vi "Core_Chem_User_Interface_v3.2_test.vi"() -> ()   [LabVIEW 2014]
uses:
  <vilib>/dex/Stream Element Allocation Mode.ctl
  C:/Program Files (x86)/National Instruments/LabVIEW 2014/examples/Data Communication/Network Streams/Simple Network Streams/support/Network Stream Command.ctl
  <vilib>/Platform/TimedLoop/XDataNode/timing_clust.ctl
  <vilib>/Platform/TimedLoop/XDataNode/nitl_modes.ctl
  <vilib>/Platform/TimedLoop/XDataNode/wakeup.ctl
  <vilib>/Utility/tcp.llb/UDP Multicast Read-Only Open.vi
  <vilib>/platform/TimedLoop/XDataNode/XDataNode.xnode
  <vilib>/Platform/TimedLoop/XDataNode/XDNodeRunTimeDep.lvlib
  <vilib>/FTP/NI_FTP.lvlib
panel:
  out "CO_fault":bool
  out "Network disconnected":bool
  out "cRIO connection status":bool
  out "Network Check error out":errorcluster
  out "SO2 Zeroing (Inflight)\nTime Remain (sec)":u32
  in  "eV6 User set time \n(Inflight) (sec)":i32=120
  in  "SO2 Inflight \nZeroing":bool
  out "Create folder error out 2":errorcluster
  out "Create folder error out":errorcluster
  in  "Confirm Flight Number":bool
  out "PRTAFT_UDP_In":string
  out "TWBOZO01":string
  out "CABOZO01":string
  out "TEIOZO01":string
  out "CHTSOO01":string
  out "CHFGGA01":string
  out "AL52CO01":string
  in  "Flight Number":string
  in  "Tab Control":T1(tab)
  out "FGGA preflight Des 17":string="Preflight - Start minimum 2 hours before take-off\n\n1. Ensure no bags/jackets are stowed on seat backs and behind seats in front of core chemistry rack at all times.\n\n2. Remove inlet covers if applicable.\n\n3. Connect Lilliput mini TFT/LCD VGA cable to FGGA VIDEO (back panel) and PS2 Keyboard/Mouse cables to FGGA Connectors (back panel). TFT/LCD screen kept in WAS/GAS rack Zargers Box. Keyboard/Mouse kept bottom of chemistry rack. (DO NOT disconnect PS2 cable). Connect TFT/LCD AC/DC PSU to 6026-8-98 Amphenol (SSP9) and make 230 Vac CB.\n\n4. Ensure all circuit breakers are pushed in, except 230Vac and 28Vdc, UPS switch off (down) and AL5002 CO Plasma Lamp switch off (down), WoW key to normal (horizontal).\n\n5. Wait for ALL network switches on the aircraft to be up and running before start-up. On the Flight Manager's Interface on the Flight Manager laptop, check SSP icons status (top row) should be all green.  \n\n6. Check AboutTime has synchronised laptop clock to aircraft timeservers (Filiberto/Gaston).\n\nClick the PowerUp Tab."
  out "FGGA preflight Des 16":string="PowerUp\n\n1.\tSSP9 forward face\tMake 3 CBs\n\n2.\tPWRDIST \t\tMake 230Vac CB \n                     Switch UPS On \t[UP]\n                     Make 28Vdc CB\n                     Check 28VDC OK Green Light comes on\n\n3.\tCore Chemistry e-Log\nComplete Core Chemistry e-Log in WordPad (Bnnn_CoreChemLog_v2.2), save on Flight Manager's laptop (192.168.101.180/      flt_folders/Bnnn); Fill in header with date, flight number and your name/initials.\n\n4. Wait for MFM flow rate to display non zero value.\n\n5.\tSAMPUMP\t\t\n - Switch WoW override key (vertical) to check pump starts, and MFM flowrate increase (>20 LPM) on the right hand plot. \n - Switch off WoW override\t\t\t\t [NORM, key horizontal]\n\nClick the 2B Ozone tab if operated, otherwise, click the UDP tab.\n\n\n"
  out "MFM":dbl(graph)
  in  "Ambient = OFF\nCabin = ON":bool
  out "FGGA preflight Des 15":string="2B Ozone Preflight\n\n1.\tSelect either Ambient or Cabin Air mode (default should be OFF for Ambient air mode).\n\n2. Check flowrate is greater than 2000 sccm on the right hand plot.\n\nClick the UDP tab."
  out "2B Ozone concentration":dbl(graph)
  out "2B Ozone flow rate":dbl(graph)
  out "2BOzone Event error out":errorcluster
  out "2BOzone command sender error out":errorcluster
  out "FGGA preflight Des 20":string="4. Check derived parameters in DECADES (192.168.101.110 & 192.168.101.108). 574 Ozone TEi49C; 588 CO AL5002; 611 SO2 TEi43i; 903 - 905 FGGA; 910 / 920 Ozone 2B."
  out "FGGA preflight Des 14":string="UDP Preflight\n1. Check all UDP packets are updating.  Unix time increasing by 1 sec (3rd parameter).\n2. Check flight number is correct.\n3. Confirm flight number and check it appears in the UDP packet (6th parameter). "
  in  "name":string="239.1.4.6"
  in  "Port":u16=50001
  out "FGGA":string
  out "CO":string
  out "TEi49 Ozone":string
  out "2B Cabin Ozone":string
  out "2B Ambient Ozone":string
  out "SO2":string
  in  "Ozone Zeroing Abort":bool
  out "Ozone Zeroing\nTime Remain (sec)":u32
  in  "Ozone Zeroing":bool
  out "TEI49 Sample Flow B":dbl(graph)
  out "TEi49 Concentration":dbl(graph)
  out "TEI49 Sample Flow A":dbl(graph)
  out "FGGA preflight Des 13":string="TEi49 Ozone PRE-FLIGHT - LAST ACTIONS BEFORE SEAT-BELTING DOWN (PRIOR TO ENGINES START)\n\n1. Ozone monitor zeroing\t\t[10 min minimum]\n\n\n2. Check TEi49 zero value and note down value in e-Log. \n"
  out "FGGA preflight Des 12":string="TEi49 Ozone Preflight\n\n1. Check nominal sample flowrate on both channels is ~0.7 LPM."
  out "Ozone Event error out":errorcluster
  out "Ozone command sender error out":errorcluster
  in  "Ozone UDP Time Offset":i32=1
  in  "eV8 span\n(sec)":i32=120
  in  "eV9 span\nflush (sec)":i32=60
  in  "SO2 Span Calibration":bool
  in  "eV9 zero\nflush (sec)":i32=15
  in  "SO2 Zero Calibration":bool
  in  "eV8 zero\n(sec)":i32=30
  in  "SO2 Calibration Abort":bool
  out "SO2 react pressure":dbl(graph)
  in  "Prepare SO2 Zero Gas":bool
  in  "Prepare SO2 Span Gas":bool
  in  "Auto Zeroing \ninterval (sec)":i32=600
  out "Next Auto Zero\nStarts in (sec)":u32
  out "Auto Zero\nIndicator":string="Auto Zero Inactive; Manual Zero Allow"
  out "SO2 Resume Zeroing\nCount down timer (sec)":u32
  in  "SO2 Pause\nAuto Zeroing":bool
  out "TEi43i Concentration scaled / raw":cluster{dbl, dbl}(graph)
  in  "SO2 Auto Zeroing":bool
  out "mean zero\ncal status":bool
  out "SO2 Sensitivity":dbl format="%.2g"
  out "SO2 Zero":dbl format="%.2g"
  in  "eV9 Flush User\nset time (sec)":i32=15
  in  "MFC_3 User Set Value":dbl=2.0
  in  "MFC_2 User Set Value":dbl=2.5
  in  "eV6 User\nset time (sec)":i32=600
  out "SO2 Flush\nTime Remain (sec)":u32
  out "TEI43i MFC3 Sample Flow":dbl(graph)
  out "TEI43C Sample Flow":dbl(graph)
  out "TEI43i MFC2 Cal Flow":dbl(graph)
  out "SO2 Zero CAL\nTime Remain (sec)":u32
  out "SO2 Zero CAL Flush\nTime Remain (sec)":u32
  in  "SO2 Zero CAL":bool
  out "FGGA preflight Des 11":string="TEi43 SO2 Inflight Zero Calibration"
  in  "SO2 GND Zeroing":bool
  out "SO2 Zeroing\nTime Remain (sec)":u32
  out "FGGA preflight Des 10":string="TEi43 SO2 PRE-FLIGHT - LAST ACTIONS BEFORE SEAT-BELTING DOWN (PRIOR TO ENGINES START)\n\n1. SO2 monitors zeroing\t\t[10 min minimum]\n\n2. Check TEi43i or TEi43C zero value and note down value in e-Log.\n\n3. Enable SO2 auto zeroing (if required) and check zeroing interval. "
  in  "SO2 Flush":bool
  out "FGGA preflight Des 9":string="TEi43 SO2 Preflight\n\n1. Check nominal sample flowrate is (2.0 LPM / 1.5 LPM) on the (TEi43i / TEi43c) right hand plot.\n\nSPAN GAS\n1. Connect SO2 Calibration gas to caldeck, then.\n\n2. Press SO2 flush button, MFC2 cal flow should increase to 2.5 SLPM.\nMonitor MFC2 flow rate to make sure the reading decreases from 2.5 SLPM to 0.0 SLPM.\nCheck pressure content and delivery gauges also reads zero.\nIf pressure content & delivery gauges do NOT read zero, press SO2 flush button again until they do.\n\n3. Back out V2, Quickly open and close cylinder valve 1, Set delivery pressure to 3 bar on V2. \n\n4. Repeat step 2) to 3) three times.\n\n5. Open cylinder valve 1, system is ready. Note down content pressure in elog.\n\n6. Press SO2 Span Calibration button to start Span calibration. \n\nZERO AIR\n1. Connect BTCA Zero Air gas to caldeck, then.\n\n2. Set ev9 flush user time to 60 secs and press SO2 Flush button.\n\n3. Press SO2 Zero Calibration button to start Zero Air calibration."
  in  "eV9 flush User\nset time (sec)":i32=30
  in  "eV8 User\nset time (sec)":i32=60
  out "SO2 Event error out":errorcluster
  out "SO2 command sender \nerror out":errorcluster
  in  "SO2 UDP Time Offset":i32=1
  in  "CO Monitor Troubleshooting":bool
  out "Lamp Temperature":dbl(graph)
  out "CO CAL Status":bool
  in  "CO CAL":bool
  out "FGGA preflight Des 8":string="CO Preflight and Inflight Calibrations\nHold down the CAL button for 2 secs then release, CAL status should then lit up.\nCheck CO LED lit up at front instrument. If not, refer to\nInflight calibration performed on 45 minutes interval or more frequently if lamp temperature > 35.5 degC."
  in  "Prepare Gases":bool
  out "FGGA preflight Des 7":string="AL5002 CO Preflight Checks\n\n1.\n\n2. Start CO Vacuum. NB: If there is problem with the software control, use manual override switch [up] on CALDECK front panel\n\n3. CO Checks - charts on the right hand side\n    Lamp Flow Controller ~ 40 ml/min\n    Monochromator Flow Controller ~ 30 ml/min\n    Fluorescence Cell Pressure ~ 7.5 Torr\n\nIf Lamp/Mono flows are low, manual valves (V1 -> V5) may still be shut, or pressure adjusting valves (ALREG1 & 2) have not been set > 2 bar\n\nIf Cell pressure is 10 Torr (max range), check that COPUMP is running and eV7 is opened (CO Vacuum eV7 is ON).\n\n4. Switch Plasma Lamp at the front panel UP\n\nDetector count rate (on 'Raw Signal' or F2 instrument touchscreen) should increase to >=10000 Hz within a minute.  Recycle plasma lamp switch (off/on) if no significant increase in count rate after 10 mins.  CO concentration should increase (100s ppb). \n     \n\n"
  in  "CO Vaccum (eV7)":bool
  out "Raw Signal":dbl(graph)
  out "CO Concentration":dbl(graph)
  out "Fluorescence Cell Pressure":dbl(graph)
  out "Monochromator Flow":dbl(graph)
  out "Lamp Flow Controller":dbl(graph)
  in  "CO UDP Time Offset":i32=1
  out "CO2 Pressure\nDelivery (PSIA)":dbl(slide) scale=0.0..100.0
  out "Std\nContent (barG)":dbl(slide) scale=0.0..220.0
  out "N2\nContent (barG)":dbl(slide) scale=0.0..220.0
  out "CO2\nContent (barG)":dbl(slide) scale=0.0..170.0
  out "CO Event error out":errorcluster
  out "CO command sender error out":errorcluster
  out "CO Zero":T2(array[cluster])
  out "CO Sensitivity":T3(array[cluster])
  in  "FGGA Calibration Abort":bool
  out "Ring Down Time RDA & RDB":cluster{dbl, dbl}(graph)
  in  "Line Lock Setting Change":bool
  out "Cell temperature":dbl(graph)
  out "Cell pressure":dbl(graph)
  in  "Manual FGGA Pump":bool
  out "CO2":dbl(graph)
  out "CH4":dbl(graph)
  out "H2O":dbl(graph)
  out "WoW Flag":string="0"
  in  "FGGA pump\nsync to WoW":bool
  out "CH4 Dry":dbl(graph)
  out "CO2 Dry":dbl(graph)
  out "MFC1 Cal Flow":dbl(graph)
  out "Flush Target Tank\nTime Remain (sec)":u32
  out "Flush Low Tank\nTime Remain (sec)":u32
  out "Flush High Tank\nTime Remain (sec)":u32
  in  "Flush Target Tank":bool
  in  "Flush Low Tank":bool
  in  "Flush High Tank":bool
  in  "FGGA Restart":bool
  out "FGGA preflight Des 6":string="FGGA Instrument Controls"
  in  "High Cal":bool
  out "High Cal\nFlush Time Remain (sec)":u32
  out "High Cal\nCal Time Remain (sec)":u32
  in  "Low Cal":bool
  in  "Target Cal":bool
  in  "Span Cal - \nHigh Cal, CO Cal, Low Cal":bool
  out "Low Cal\nFlush Time Remain (sec)":u32
  out "Low Cal\nCal Time Remain (sec)":u32
  out "Target Cal\nFlush Time Remain (sec)":u32
  out "Target Cal\nCal Time Remain (sec)":u32
  in  "MFC_1 User Set Value":dbl=2.0
  out "FGGA preflight Des 5":string="FGGA Inflight Calibrations"
  out "FGGA preflight Des 4":string="FGGA Ground Preflight Checks\n\n1. Switch FGGA pump ON\n\n2. Check cavity pressure ~50 Torr\n\n3. Switch FGGA pump OFF\n\n4. Enable FGGA pump sync to WoW\n\n5.. Check Time Synchronisation\n\n6. Check CO2 & CH4 values\n\nIf CO2 & CH4 values are -1 ppm, follow the \nchange linelock settings procedure.\n\n\n\n\n\nLAST ACTION BEFORE SEAT-BELTING \nDOWN (PRIOR TO ENGINES START)\n\n1. Disconnect Monitor & stow away. Leave Keyboard & Mouse connected. Place keyboard at the bottom\nof the rack.\n\n"
  out "FGGA preflight Des 3":string="FGGA CAL Gas Purge\n\nFor each cylinder in gas stowage, check that,\n\n1. V1 Closed\n    V3 Closed\n    V4 Make sure arrow positioned downwards (i.e. flow points to gas line)\n\n2. V3 Open (turn anti-clockwise)\n\n3. Use the button on the right according to the operating cylinder to flush the line. Monitor the MFC flow rate to make sure the reading decreases from 3 to zero. (ie fully flushed). Pressure content & delivery gauges should also read zero.\n\n4. V3 Close (turn clockwise)\n\n5. V1 Open / Close quickly\n         Check delivery pressure gauge is ~ 40 PSI \n         (Use V2 to increase if necessary)\n\n6. Repeat steps 2) to 5) three times\n\n7. V3 Close (turn clockwise)\n\n8. V1 Open, check V2 ~ 40 PSIG\n\n9. V3 Open - System is ready"
  out "FGGA command sender error out":errorcluster
  out "FGGA Event Error out":errorcluster
  in  "FGGA UDP Time Offset":i32=1
  in  "FGGA Shutdown":bool
  in  "Postflight Procedures":bool
  in  "FTP ASCII Files to Local":bool
  in  "Transfer FGGA Files":bool
  out "FGGA preflight Des 18":string="Postflight\n\n1. Perform SO2 Span Gas Calibration (if necessary). \n\n2. Press the FTP ASCII File to Local button to transfer ASCII files to flight folder.\n\n\n3. Press the Transfer FGGA Files button to transfer FGGA files to flight folder. \n\n\n4. Shutdown FGGA.\n\n\n5. View Postflight Procedures."
  out "File List":string[](array[string])
  out "FGGA File Transfer Error out":errorcluster
  out "Move to FM Error out":errorcluster
  out "USB Disk Space Used %":dbl(slide) scale=0.0..100.0
  out "PTP Sync":bool
  out "CPU Total %":dbl(graph)
  out "PRTAFT_DLU":string
  in  "Pause Auto Zero Count \nDown set time (sec)":i32=600
  out "Calibration gas cylinder \nconcentration (ppb)":dbl format="%.4g"
  in  "Save Calibration gas\ncylinder concentration to file":bool
  in  "Calibration gas cylinder \nconcentration (ppb)":dbl=500.0 format="%.4g"
  in  "Simulate MOCCA Conc":dbl
  in  "MOCCA window \ndelay time (sec)":i32=30
  in  "MOCCA Limit":i32=800
  in  "SO2 Inflight MOCCA Alarm\n(default = OFF)":bool
  in  "Offset Mean Zero Calculation (default = ON)\nOFF = User input\nOn = Mean zero calculated with ev8":bool=TRUE
  out "FGGA preflight Des 19":string="This tab controls ONLY for advanced operators."
  in  "Inst_alm_thresh":i32=220
  in  "3hr_alm_thresh":i32=80
  in  "Simulate Inst Conc":i32
  in  "Simulate 3hr Average Conc":dbl
  in  "Simulate 2B Conc":bool
  in  "Ozone eV6":bool
  in  "Simulate Conc":bool
  in  "8hr TWA Limit":i32=490
  in  "10mins STEL Limit":i32=800
  in  "SO2 Sensitivity":dbl=1.1
  in  "SO2 Zero":dbl
  in  "Simulate TWA Conc":dbl
  in  "Simulate STEL Conc":dbl
  in  "MFC_3\nSLPM Value":dbl=2.0
  in  "MFC_2\nSLPM Value":dbl
  in  "SO2 eV6":bool
  in  "eV8":bool
  in  "eV9":bool
  in  "eV4":bool
  in  "eV3":bool
  in  "MFC_1\nSLPM Value":dbl
  in  "eV2":bool
  in  "eV1":bool
  in  "cRIO File IO Stop\n(USB Flash Drive Unmount)":bool
  # "Unix time"
  # "Flight Number"
  # "concentration (scaled)\npmt_volt\nlamp_volt\nlamp_intens\ninternal_temper\nreact_temper\nreact_press\nflow\nflags\nten_min_so2\neight_hr_so2\nten_min_so2_alm\neight_hr_so2_alm\nMFC_2absolute_pres\nMFC_2temperature\nMFC_2volumetic_flow\nMFC_2mass_flow\nMFC_2set_point\nMFC_3_absolute_pres\nMFC_3_temperature\nMFC_3volumetic_flow\nMFC_3mass_flow\nMFC_3set_point\nV6\nV8\nV9\nMFC2_Set_Value\nMFC3_Set_Value\nconcentration (raw)\nmean calculation status\noffset\nsensitivity\nev8_user_set_time\nauto_zeroing_control\nev8_zero_interval\nMOCCA_inflight_alarm\nMOCCA_time_window_delay\nMOCCA_SO2_limit\n10 min STEL limit\n8 hour TWA limit\nSO2 cal gas cylin conc\nsimulate_SO2_conc_control\nMOCCA_SO2_sim_value\nMOCCA_SO2_alarm"
  # "Unix time"
  # "Unix time"
  # "Unix time"
  # "Unix time"
  # "Flight Number"
  # "Flight Number"
  # "Flight Number"
  # "Flight Number"
  # "conc\ntemp\npress\nflow\nthreehr_oz\nInst_alarm\nthreehr_alarm"
  # "ch4\nco2\nh2o\npress_torr\ntemp_c\nfit_flag\nrda_usec\nrdb_usec\nch4_dry\nco2_dry\nMFC_1_absolute_pres\nMFC_1_temperature\nMFC_1volumetic_flow\nMFC_1mass_flow\nMFC_1set_point\nV1\nV2\nV3\nV4\nrestart_FGGA\nFGGA_Pump\nCAL_MFC_1Set_Value"
  # "conc\ntemp\npress\nflow"
  # "conc\nbenchtemp\npress\ncellAint\ncellBint\nFlowA\nFlowB\nlamptemp\nflag\nV6"
  # "conc\ncounts\nsens\nzero\nlampflow\nlamptemp\nmonoflow\nmonotemp\nmonopress\ncellpress\ncalpress\ntemppmt\ncalconc\nerr\ncal_counter\nerr_counter\nCO_vacuum_status\nIn_Cal\nALEG1_press_delivery\nALREG1_press_content\nALREG2_press_content\nALREG3_press_content"
  # "TEi43c"
  # "TEi43i"
  # "SO2 Inflight ZERO CAL SETTINGS"
  # "FGGA"
  # "2B Ozone"
  # "TEi49C  - Ozone"
  # "TEi43 - SO2"
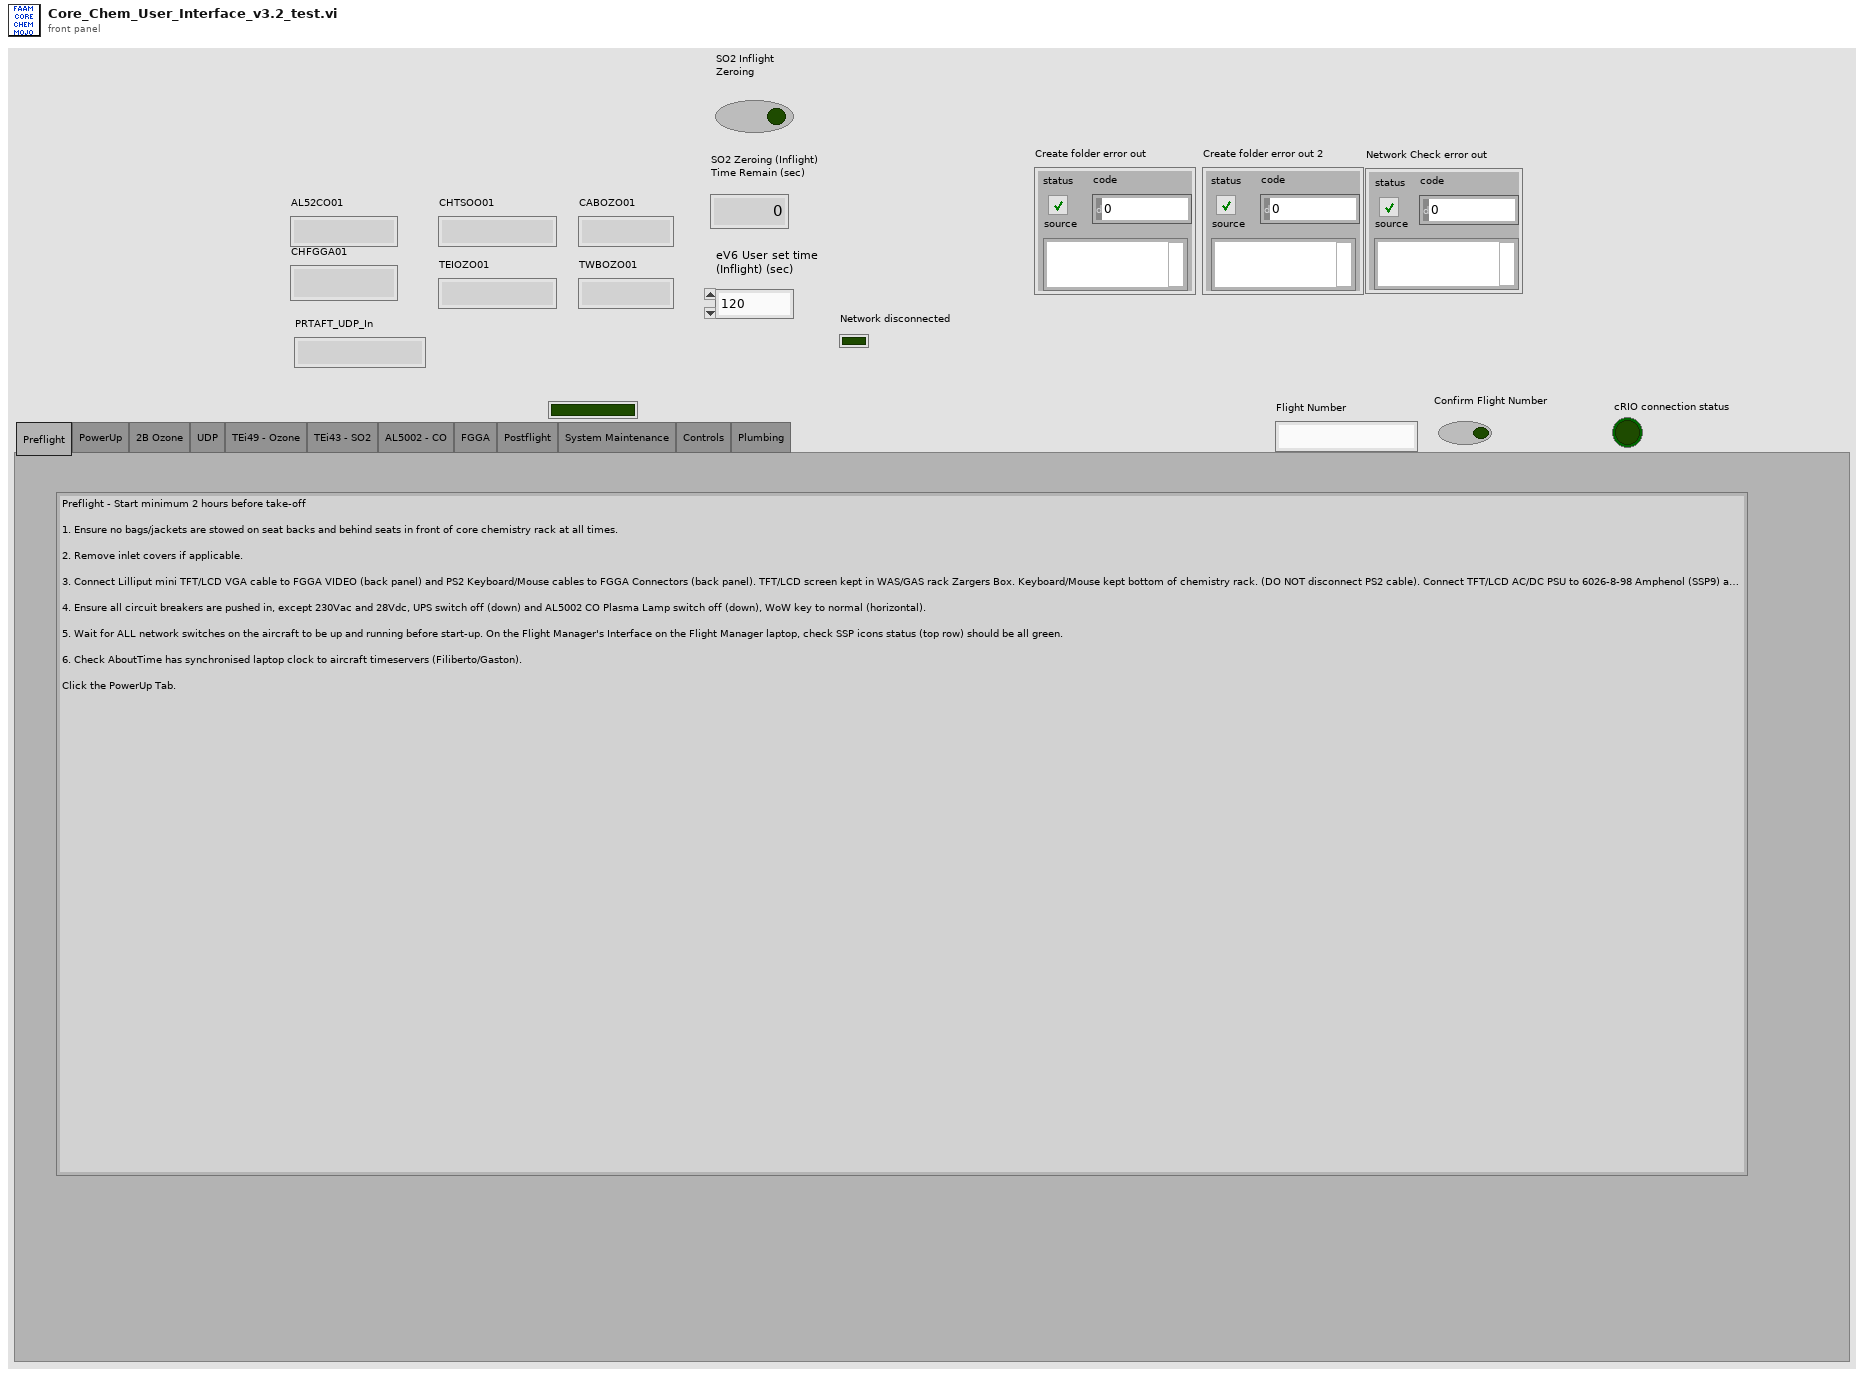
[diagram p1: front panel]
types:
  T1 = enum32{"Preflight", "PowerUp", "2B Ozone", "UDP", "TEi49 - Ozone", "TEi43 - SO2", "AL5002 - CO", "FGGA", "Postflight", "System Maintenance", "Controls", "Plumbing"}
  T2 = cluster{"time stamp":timestamp, "CO Offset":dbl}[]
  T3 = cluster{"time stamp":timestamp, "CO Sensitivity":dbl}[]
  T4 = typedef "Network Stream Command.ctl" = cluster{"Message":string, "Message Data":variant}
  T5 = typedef "Stream Element Allocation Mode.ctl" = u32
  T6 = typedef "XDNodeRunTimeDep.lvlib/timing_clust.ctl" = cluster{"Expected End [f-1]":u64, "Actual End [f-1]":u64, "Finished Late? [f-1]":bool, "Expected End [i-1]":u64, "Actual End [i-1]":u64, "Finished Late? [i-1]":bool, "Expected Start [i]":u64, "Actual Start [i]":u64, "Expected Start [f]":u64, "Actual Start [f]":u64, "Source Name":string, "Structure Name":string, "Period":i64, "Deadline":i64, "Offset":i64, "Start":i64, "Priority":i32, "Timeout":i32, "Mode":T7, "Wakeup Reason":T8, "Error":errorcluster, "Source Type":string, "Secondary Source Type":string, "Global End Time":u64, "Global Start Time":u64, "Frame Duration":u64, "Iteration Duration":u64, "Assigned CPU":i32, "I/O Scan Engine Mode":u32}
  T7 = typedef "XDNodeRunTimeDep.lvlib/nitl_modes.ctl" = enum32{"No Change", "Process missed periods, maintain original phase", "Discard missed periods, maintain original phase", "Process missed periods, ignore original phase", "Discard missed periods, ignore original phase"}
  T8 = typedef "XDNodeRunTimeDep.lvlib/wakeup.ctl" = enum32{"Normal", "Aborted", "Asynchronous wakeup", "Timing source error", "Timed loop error", "Timeout"}
  T9 = typedef "NI_FTP.lvlib/FTP Session.ctl" = refnum<k5>
  T10 = typedef "NI_FTP.lvlib/FTP File Info.ctl" = cluster{"type":enum16{"unknown", "file", "dir", "link"}, "permissions":string, "owner":string, "group":string, "size":i32, "date":string, "name":string, "link name":string}
  T11 = cluster{"Message":string, "Message 2":string, "Message 3":string}
  T12 = cluster{"Message":string, "Message 2":string, "Message 3":string, "Message 4":string}
  T13 = cluster{"Message":string, "Message 3":string, "Message 4":string}
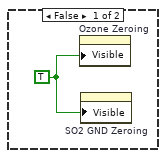
[diagram p2: hidden frame]
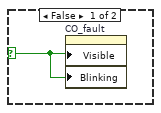
[diagram p3: hidden frame]
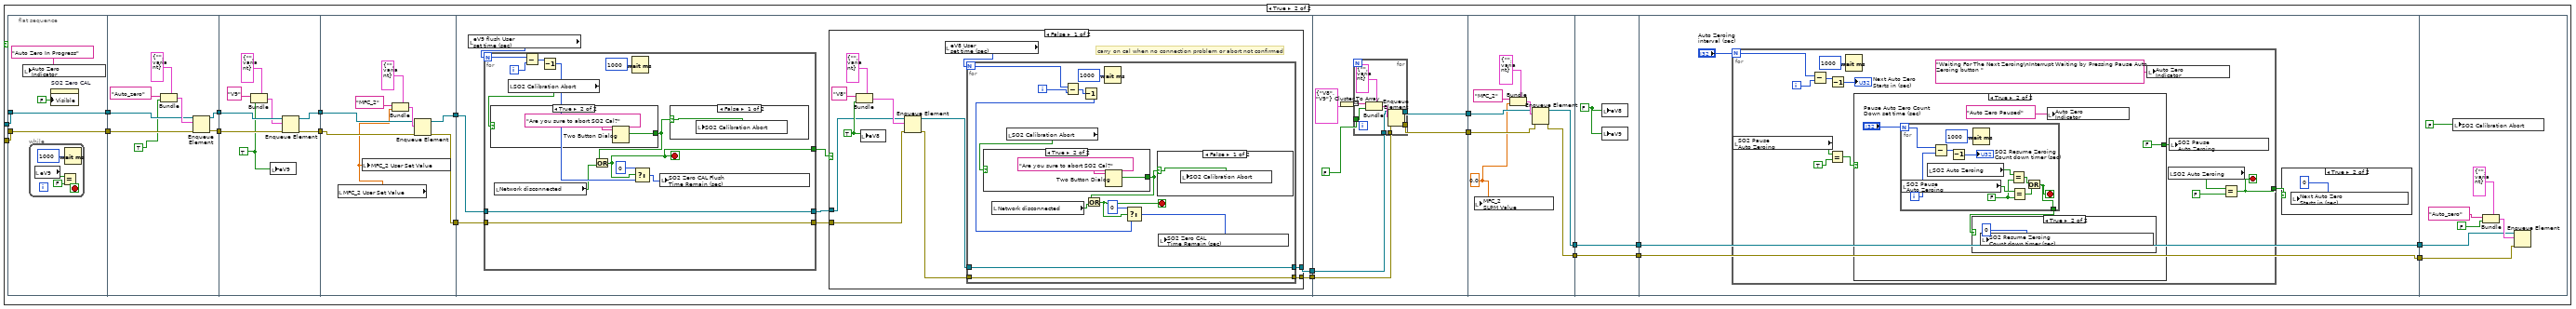
[diagram p8: hidden frame]
diagram:
  w8 = "XXXX"
  w10 = 0
  w11 = 0.0
  w17 = T4 {"Message"="", "Message Data"=variant} ("Message Cluster")
  w23 = T5 0 items=["allocate as needed", "pre-allocate"] ("element allocation mode")
  w29 = T4 {"Message"="", "Message Data"=variant} ("Message Cluster")
  w35 = T5 0 items=["allocate as needed", "pre-allocate"] ("element allocation mode")
  w40 = T4 {"Message"="", "Message Data"=variant} ("Message Cluster")
  w45 = T5 0 items=["allocate as needed", "pre-allocate"] ("element allocation mode")
  w54 = T5 0 items=["allocate as needed", "pre-allocate"] ("element allocation mode")
  w56 = T4 {"Message"="", "Message Data"=variant} ("Message Cluster")
  w63 = T5 0 items=["allocate as needed", "pre-allocate"] ("element allocation mode")
  w65 = T4 {"Message"="", "Message Data"=variant} ("Message Cluster")
  n1 = local write "cRIO File IO Stop\n(USB Flash Drive Unmount)"(FALSE ("Stop File Write")) -> ()
  n2 = local write "Flight Number"(w8) -> ()
  n3 = while {
    shift-right: [w69] -> _
    shift-left: w8 -> [w68]
    stop <- FALSE stop-if-true
    n4 = Not Equal?(x=w68, y="Flight Number") -> (x != y?=w71:bool)
    n5 = case shown="True" w71 {
      tunnel: [w74 w75] -> w69
      tunnel: "Flight Number" -> [_ w75]
      tunnel: w68 -> [w74 _]
      frame False {
      }
      frame True {
        n6 = One Button Dialog(message="Flight Number changed,\nPress flight number button to confirm") -> ()  [unwired: 1 in, 1 out]
      }
    }
    n7 = Wait (ms)(milliseconds to wait=u32 1000) -> ()  [unwired: 1 out]
  }
  n8 = while {
    stop <- FALSE stop-if-true
    # "UDP Read"
    n9 = String To IP(1:"name") -> (0:w82:u32)
    n10 = call-poly <vilib>:"UDP Multicast Open.vi"("multicast addr"=w82, "port"="Port") -> ("error out"=w80:errorcluster, "connection ID"=w79:refnum<k16>)  [unwired: 7 in, 1 out]
    n11 = Wait (ms)(milliseconds to wait=u32 1000) -> ()  [unwired: 1 out]
    n12 = case shown="No Error" w80 {
      selector: w80 -> [w86 _]
      tunnel: w79 -> [w85 _]
      frame No Error {
        w84 = ""
        n13 = while {
          tunnel: w86 -> [w132]
          tunnel: w85 -> [w131]
          shift-right: [w127] -> _
          shift-left: w84 -> [w128]
          shift-right: [w118] -> _
          shift-left: w84 -> [w120]
          shift-right: [w112] -> _
          shift-left: w84 -> [w114]
          shift-right: [w106] -> _
          shift-left: w84 -> [w107]
          shift-right: [w100] -> _
          shift-left: w84 -> [w101]
          shift-right: [w94] -> _
          shift-left: w84 -> [w95]
          shift-right: [w88] -> _
          shift-left: w84 -> [w89]
          stop <- w130 stop-if-true
          n14 = UDP Read(connection ID=w131, 8:w132) -> (data out=w87:string, error out=w130:errorcluster)  [unwired: 2 in, 3 out]
          n15 = Match Pattern(string=w87, regular expression="$TEIOZO") -> (match substring=w126:string, after substring=w125:string)  [unwired: 1 in, 2 out]
          n16 = Match Pattern(string=w87, regular expression="$TWBOZO01,") -> (match substring=w104:string, after substring=w103:string)  [unwired: 1 in, 2 out]
          n17 = Match Pattern(string=w87, regular expression="$CABOZO01,") -> (match substring=w110:string, after substring=w109:string)  [unwired: 1 in, 2 out]
          n18 = Match Pattern(string=w87, regular expression="$CHTSOO") -> (match substring=w98:string, after substring=w97:string)  [unwired: 1 in, 2 out]
          n19 = Match Pattern(string=w87, regular expression="$CHFGGA01,") -> (match substring=w122:string, after substring=w121:string)  [unwired: 1 in, 2 out]
          n20 = Match Pattern(string=w87, regular expression="$AL52CO01,") -> (match substring=w116:string, after substring=w115:string)  [unwired: 1 in, 2 out]
          n21 = Match Pattern(string=w87, regular expression="$PRTAFT01,") -> (match substring=w93:string, after substring=w92:string)  [unwired: 1 in, 2 out]
          n22 = Concatenate Strings(w126, w125) -> (w124:string)
          n23 = Concatenate Strings(w104, w103) -> (w102:string)
          n24 = Concatenate Strings(w110, w109) -> (w108:string)
          n25 = Concatenate Strings(w98, w97) -> (w96:string)
          n26 = Concatenate Strings(w122, w121) -> (w119:string)
          n27 = Concatenate Strings(w116, w115) -> (w113:string)
          n28 = Concatenate Strings(w93, w92) -> (w90:string)
          n29 = Replace Substring(4:w102, 5:w101) -> (1:w100:string)  [unwired: 2 in, 1 out]
          "TWBOZO01" <- w100
          n30 = Replace Substring(4:w124, 5:w128) -> (1:w127:string)  [unwired: 2 in, 1 out]
          "TEIOZO01" <- w127
          n31 = Replace Substring(4:w108, 5:w107) -> (1:w106:string)  [unwired: 2 in, 1 out]
          "CABOZO01" <- w106
          n32 = Replace Substring(4:w96, 5:w95) -> (1:w94:string)  [unwired: 2 in, 1 out]
          "CHTSOO01" <- w94
          n33 = Replace Substring(4:w113, 5:w114) -> (1:w112:string)  [unwired: 2 in, 1 out]
          "AL52CO01" <- w112
          n34 = Replace Substring(4:w119, 5:w120) -> (1:w118:string)  [unwired: 2 in, 1 out]
          "CHFGGA01" <- w118
          n35 = Replace Substring(4:w90, 5:w89) -> (1:w88:string)  [unwired: 2 in, 1 out]
          "PRTAFT_UDP_In" <- w88
        }
      }
      frame Error {
      }
    }
  }
  n36 = Obtain Queue(name (unnamed)="CO_Command", element data type=w65) -> (queue out=w16:refnum<queue>, error out=w59:errorcluster)  [unwired: 3 in, 1 out]
  n37 = Create Network Stream Writer Endpoint(6:w63, 7:10 ("writer buffer size"), 9:w65, 10:"//192.168.101.17/command/reader/CO" ("reader url"), 11:"/command/writer/CO" ("writer name")) -> (0:w62:errorcluster, 3:w61:refnum<k21>)  [unwired: 2 in]
  n38 = while {
    tunnel: w16 -> [w136]
    tunnel: w59 -> [w135]
    tunnel: [w133] -> _
    stop <- FALSE stop-if-true
    # "CO UI Event Handler Loop"
    n39 = event shown="[4] \"Confirm Flight Number\": Value Change" {
      selector: _ -> [_ _ _ _ _]
      dyn-events: _ -> [_ _ _ _ _]
      timeout: _ -> [_ _ _ _ _]
      tunnel: w136 -> [w143 w150 w154 w161 w169]
      tunnel: w135 -> [w142 w149 w153 w160 w168]
      tunnel: [w137 w144 w152 w159 w167] -> w133
      event "CO CAL": Value Change {
        n40 = event-data() -> ("NewVal"=w140:bool)  [unwired: 1 in]
        n41 = Bundle(cluster=T4 {"Message"="", "Message Data"=variant} ("Message Cluster"), "Message"="CO CAL", "Message Data"=w140) -> (w138:T4)
        n42 = Enqueue Element(queue=w143, element=w138, error in (no error)=w142) -> (error out=w137:errorcluster)  [unwired: 1 in, 2 out]
      }
      event "CO UDP Time Offset": Value Change {
        n43 = event-data() -> ("NewVal"=w147:i32)  [unwired: 1 in]
        n44 = Bundle(cluster=T4 {"Message"="", "Message Data"=variant} ("Message Cluster"), "Message"="UDP Time Offset", "Message Data"=w147) -> (w145:T4)
        n45 = Enqueue Element(queue=w150, element=w145, error in (no error)=w149) -> (error out=w144:errorcluster)  [unwired: 1 in, 2 out]
      }
      event "CO Vaccum (eV7)": Value Change {
        n46 = event-data() -> ("NewVal"=w151:bool)  [unwired: 1 in]
        n47 = Bundle(cluster=T4 {"Message"="", "Message Data"=variant} ("Message Cluster"), "Message"="CO Vacuum", "Message Data"=w151) -> (w155:T4)
        n48 = Enqueue Element(queue=w154, element=w155, error in (no error)=w153) -> (error out=w152:errorcluster)  [unwired: 1 in, 2 out]
      }
      event "cRIO File IO Stop\n(USB Flash Drive Unmount)": Value Change {
        n49 = event-data() -> ("NewVal"=w158:bool)  [unwired: 1 in]
        n50 = Bundle(cluster=T4 {"Message"="", "Message Data"=variant} ("Message Cluster"), "Message"="Stop File Write", "Message Data"=w158) -> (w162:T4)
        n51 = Enqueue Element(queue=w161, element=w162, error in (no error)=w160) -> (error out=w159:errorcluster)  [unwired: 1 in, 2 out]
      }
      event "Confirm Flight Number": Value Change {
        n52 = event-data() -> ()  [unwired: 1 in, 1 out]
        n53 = flat-sequence {
          tunnel: w168 -> [w171]
          tunnel: w169 -> [w172]
          tunnel: [w172] -> w166
          tunnel: [w171] -> w165
          tunnel: [w174] -> w167
          tunnel: w166 -> [w176]
          tunnel: w165 -> [w175]
          frame #0 {
            n54 = local write "cRIO File IO Stop\n(USB Flash Drive Unmount)"(FALSE ("cRIO File IO Stop\n(USB Flash Drive Unmount)")) -> ()
          }
          frame #1 {
            n55 = local read "Flight Number"() -> (w173:string)
            n56 = Bundle(cluster=T4 {"Message"="", "Message Data"=variant} ("Message Cluster"), "Message"="Flight Number", "Message Data"=w173) -> (w177:T4)
            n57 = Enqueue Element(queue=w176, element=w177, error in (no error)=w175) -> (error out=w174:errorcluster)  [unwired: 1 in, 2 out]
          }
        }
      }
    }
    "CO Event error out" <- w133
  }
  n58 = while {
    tunnel: w16 -> [w187]
    shift-right: [w182] -> _
    shift-left: w61 -> [w184]
    shift-right: [w180] -> w50
    shift-left: w62 -> [w186]
    tunnel: w59 -> [w181]
    stop <- w180 stop-if-true
    # "CO UI Command Sender"
    n59 = Dequeue Element(queue=w187, error in (no error)=w181) -> (element=w183:T4)  [unwired: 1 in, 3 out]
    n60 = Unbundle By Name(w183) -> ("Message"=w185:string)
    n61 = case shown="\"UDP Time Offset\"" w185 {
      tunnel: w186 -> [w188 w192 w199 w206 w213 w220]
      tunnel: w184 -> [w189 w195 w202 w209 w216 w223]
      tunnel: w183 -> [_ w194 w201 w208 w215 w222]
      tunnel: [w188 w191 w198 w205 w212 w219] -> w180
      tunnel: [w189 w190 w197 w204 w211 w218] -> w182
      frame "False", Default {
      }
      frame "CO CAL" {
        n62 = shared-variable-write(w195, w192, w194) -> (w193:refnum<k21>, w196:errorcluster)  [unwired: 1 in, 1 out]
        n63 = Flush Stream(8:w196, 11:w193) -> (0:w191:errorcluster, 3:w190:refnum<k21>)  [unwired: 2 in, 1 out]
      }
      frame "UDP Time Offset" {
        n64 = shared-variable-write(w202, w199, w201) -> (w200:refnum<k21>, w203:errorcluster)  [unwired: 1 in, 1 out]
        n65 = Flush Stream(8:w203, 11:w200) -> (0:w198:errorcluster, 3:w197:refnum<k21>)  [unwired: 2 in, 1 out]
      }
      frame "Stop File Write" {
        n66 = shared-variable-write(w209, w206, w208) -> (w207:refnum<k21>, w210:errorcluster)  [unwired: 1 in, 1 out]
        n67 = Flush Stream(8:w210, 11:w207) -> (0:w205:errorcluster, 3:w204:refnum<k21>)  [unwired: 2 in, 1 out]
      }
      frame "Flight Number" {
        n68 = shared-variable-write(w216, w213, w215) -> (w214:refnum<k21>, w217:errorcluster)  [unwired: 1 in, 1 out]
        n69 = Flush Stream(8:w217, 11:w214) -> (0:w212:errorcluster, 3:w211:refnum<k21>)  [unwired: 2 in, 1 out]
      }
      frame "CO Vacuum" {
        n70 = shared-variable-write(w223, w220, w222) -> (w221:refnum<k21>, w224:errorcluster)  [unwired: 1 in, 1 out]
        n71 = Flush Stream(8:w224, 11:w221) -> (0:w219:errorcluster, 3:w218:refnum<k21>)  [unwired: 2 in, 1 out]
      }
    }
  }
  "CO command sender error out" <- w50
  n72 = node-c288() -> (w15:T6)  [unwired: 4 in]
  n73 = Initialize Array(cluster{"time stamp":timestamp, "Y":dbl} {"time stamp"=timestamp(0 s since 1904-01-01), "Y"=0.0}, 30 ("dimension size")) -> (w12:cluster{"time stamp":timestamp, "Y":dbl}[])
  n74 = timed-loop {
    timing: w15 -> [_]
    timing-out: [_] -> w14
    stop <- _ stop-if-true
    # "PC Tasks"
    n75 = node-c288() -> ()  [unwired: 1 in, 1 out]
    n76 = event shown="[1] \"Transfer FGGA Files\": Value Change" {
      selector: _ -> [_ _ _ _]
      dyn-events: _ -> [_ _ _ _]
      timeout: _ -> [_ _ _ _]
      event "FTP ASCII Files to Local": Value Change {
        n77 = event-data() -> ()  [unwired: 1 in, 1 out]
        n78 = flat-sequence {
          tunnel: [w233] -> w227
          tunnel: [w245] -> w232
          tunnel: [w244] -> w230
          tunnel: [w243] -> w228
          tunnel: w227 -> [w243]
          tunnel: w232 -> [w303]
          tunnel: [w303] -> w231
          tunnel: w230 -> [w299]
          tunnel: [w298] -> w229
          tunnel: w228 -> [w298]
          tunnel: w231 -> [w309]
          tunnel: w229 -> [w304]
          frame #0 {
            n79 = local read "Flight Number"() -> (w235:string)
            n80 = Concatenate Strings("Confirm Flight Number" ("message"), "\n", w235) -> (w239:string)
            n81 = Two Button Dialog(message=w239, 1:"No" ("F button name (\"Cancel\")"), 2:"Yes" ("T button name (\"OK\")")) -> (T button?=w236:bool)
            n82 = case shown="False" w236 {
              tunnel: w235 -> [_ w242]
              tunnel: [w241 w242] -> w233
              frame False {
                n83 = call "Prompt User for Flight Number2"() -> ("Flight Number BXXX"=w241:string)  [unwired: 17 in, 2 out]
              }
              frame True {
              }
            }
          }
          frame #1 {
            n84 = Get Date/Time In Seconds() -> (seconds since 1Jan1904=w249:timestamp)
            n85 = Format Date/Time String(time format string (%c)="%Y%m%d", seconds (now)=w249) -> (date/time string=w247:string)  [unwired: 1 in]
            n86 = call <vilib>:"FTP Open Session.vi"("address"="192.168.101.17") -> ("error out"=w264:errorcluster, "ftp session"=w265:T9)  [unwired: 7 in, 2 out]
            n87 = Concatenate Strings("Use Today's Date" ("message"), "\r", w247) -> (w253:string)
            n88 = call <vilib>:"FTP Logon.vi"("error in (no error)"=w264, "password"="", "user"="anonymous", "ftp session"=w265) -> ("error out"=w261:errorcluster, "ftp session out"=w260:T9)  [unwired: 4 in, 2 out]
            n89 = Two Button Dialog(message=w253, 1:"No" ("F button name (\"Cancel\")"), 2:"Yes" ("T button name (\"OK\")")) -> (T button?=w250:bool)
            n90 = case shown="False" w250 {
              tunnel: [w268 w269] -> w244
              tunnel: w247 -> [_ w269]
              frame False {
                n91 = call "Prompt User for Date"() -> ("Date"=w268:string)  [unwired: 17 in, 2 out]
              }
              frame True {
              }
            }
            n92 = call <vilib>:"FTP Directory Listing.vi"("error in (no error)"=w261, "directory path"="/U:/data", "ftp session"=w260) -> ("dir list"=w259:T10[])  [unwired: 4 in, 4 out]
            n93 = for {
              tunnel: w259 -> [w289] mode=indexing
              tunnel: [w288] -> w256 mode=indexing
              tunnel: w244 -> [w287]
              # "Extract File Name According to the Date"
              n94 = Unbundle By Name(w289) -> ("name"=w295:string, "name"=w294:string)
              n95 = Match Pattern(string=w294, regular expression="_[0-9]+") -> (match substring=w292:string)  [unwired: 1 in, 3 out]
              n96 = String Subset(string=w292, offset (0)=1) -> (substring=w290:string)  [unwired: 1 in]
              n97 = Equal?(x=w290, y=w287) -> (x = y?=w296:bool)
              n98 = case shown="False" w296 {
                tunnel: w295 -> [_ w297]
                tunnel: [_ w297] -> w288
                frame False {
                }
                frame True {
                }
              }
            }
            n99 = Array Size(array=w256) -> (size(s)=w258:i32)
            n100 = for {
              N: w258 -> [_]
              shift-right: [w276] -> w246
              shift-left: w256 -> [w277]
              shift-right: [w274] -> _
              shift-left: 0 -> [w275]
              # "Remove Empty Array"
              n101 = Index Array(array=w277, index=w275) -> (element=w279:string)
              n102 = Equal?(x=w279, y="") -> (x = y?=w278:bool)
              n103 = case shown="True" w278 {
                tunnel: w277 -> [w283 w286]
                tunnel: w275 -> [w282 w284]
                tunnel: [w283 w285] -> w276
                tunnel: [w281 w284] -> w274
                frame False {
                  n104 = Increment(x=w282) -> (x+1=w281:i32)
                }
                frame True {
                  n105 = Delete From Array(array=w286, index=w284) -> (array with subset deleted=w285:string[])  [unwired: 1 in, 1 out]
                }
              }
            }
            "File List" <- w246
            n106 = for {
              tunnel: w246 -> [w272] mode=indexing
              tunnel: [w270] -> w245 mode=indexing
              # "Specify destination path for each file"
              n107 = Concatenate Strings("C:\\temp\\", w272) -> (w271:string)
              n108 = String To Path(string=w271) -> (path=w270:path)
            }
          }
          frame #2 {
            # "FTP a list of files"
            n109 = call <vilib>:"System Exec.vi"("wait until completion? (T)"=TRUE, "working directory"=path "C:/temp", "standard input"=w299, "command line"="C:\\temp\\transfer_ascii_files.bat") -> ()  [unwired: 4 in, 4 out]
          }
          frame #3 {
            # "Move file from local PC to Flight Folder"
            n110 = Build Path(base path=path "\\\\192.168.101.180\\flt_folders" ("path"), name or relative path=w304) -> (appended path=w311:path)
            n111 = Concatenate Strings(w304, "_" ("string"), "corechem" ("string")) -> (w310:string)
            n112 = Build Path(base path=w311, name or relative path=w310) -> (appended path=w306:path)
            n113 = Create Folder(path (use dialog)=w306) -> (created path=w305:path, error out=→"Create folder error out 2":errorcluster)  [unwired: 2 in, 1 out]
            n114 = for {
              tunnel: w305 -> [w318]
              tunnel: [w317] -> w308
              tunnel: w309 -> [w315] mode=indexing
              n115 = Copy(9:TRUE ("overwrite (F)"), 10:w318, 11:w315) -> (0:w317:errorcluster)  [unwired: 2 in, 2 out]
            }
            "Move to FM Error out" <- w308
          }
          frame #4 {
            n116 = local write "FTP ASCII Files to Local"(FALSE ("FTP Files to Local")) -> ()
          }
        }
      }
      event "Transfer FGGA Files": Value Change {
        n117 = event-data() -> ()  [unwired: 1 in, 6 out]
        n118 = flat-sequence {
          tunnel: [w324] -> w323
          tunnel: w323 -> [w336]
          tunnel: [w336] -> w322
          tunnel: [w335] -> w321
          tunnel: [w334] -> w320
          tunnel: w322 -> [w346]
          tunnel: w321 -> [w345]
          tunnel: w320 -> [w347]
          frame #0 {
            n119 = local read "Flight Number"() -> (w325:string)
            n120 = Concatenate Strings("Confirm Flight Number" ("message"), "\n", w325) -> (w327:string)
            n121 = Two Button Dialog(message=w327, 1:"No" ("F button name (\"Cancel\")"), 2:"Yes" ("T button name (\"OK\")")) -> (T button?=w331:bool)
            n122 = case shown="False" w331 {
              tunnel: w325 -> [_ w333]
              tunnel: [w332 w333] -> w324
              frame False {
                n123 = call "Prompt User for Flight Number"() -> ("Flight Number BXXX"=w332:string)  [unwired: 17 in, 2 out]
              }
              frame True {
              }
            }
          }
          frame #1 {
            n124 = Two Button Dialog(message="Get FGGA Files\nof Today's Date?", 1:"No" ("F button name (\"Cancel\")"), 2:"Yes" ("T button name (\"OK\")")) -> (T button?=w340:bool)
            n125 = case shown="False" w340 {
              selector: w340 -> [w342 w343]
              tunnel: [w342 w343] -> w334
              tunnel: [w341 _] -> w335
              frame False {
                n126 = call "Prompt User for Date"() -> ("Date"=w341:string)  [unwired: 17 in, 2 out]
              }
              frame True {
              }
            }
          }
          frame #2 {
            n127 = Build Path(base path=path "\\\\192.168.101.180\\flt_folders" ("path"), name or relative path=w346) -> (appended path=w351:path)
            n128 = Concatenate Strings(w346, "_" ("string"), "corechem" ("string")) -> (w350:string)
            n129 = Build Path(base path=w351, name or relative path=w350) -> (appended path=w344:path)
            n130 = Create Folder(path (use dialog)=w344) -> (error out=→"Create folder error out":errorcluster)  [unwired: 2 in, 2 out]
            n131 = call "labSSH_FGGA_Files_Transfer.vi"("Flight_num"=w346, "Get current?"=w347, "Date"=w345, "Flight Folder Path"=w344) -> ("error IO"=→"FGGA File Transfer Error out":errorcluster)  [unwired: 11 in]
          }
          frame #3 {
            n132 = local write "Transfer FGGA Files"(FALSE) -> ()
          }
        }
      }
      event "FGGA Restart": Value Change {
        n133 = event-data() -> ()  [unwired: 1 in, 6 out]
        n134 = flat-sequence {
          frame #0 {
            n135 = Two Button Dialog(message="FGGA will be restarted,\nARE YOU SURE?") -> (T button?=w357:bool)  [unwired: 2 in]
            n136 = case shown="True" w357 {
              frame False {
              }
              frame True {
                n137 = call "labSSH_Commands.vi"("Data"="reboot") -> ()  [unwired: 14 in, 1 out]
              }
            }
          }
          frame #1 {
            n138 = local write "FGGA Restart"(FALSE ("FGGA Restart")) -> ()
          }
        }
      }
      event "FGGA Shutdown": Value Change {
        n139 = event-data() -> ()  [unwired: 1 in, 6 out]
        n140 = flat-sequence {
          frame #0 {
            n141 = Two Button Dialog(message="FGGA will be shutdown,\nARE YOU SURE?") -> (T button?=w361:bool)  [unwired: 2 in]
            n142 = case shown="True" w361 {
              frame False {
              }
              frame True {
                n143 = call "labSSH_Commands.vi"("Data"="halt") -> ()  [unwired: 14 in, 1 out]
              }
            }
          }
          frame #1 {
            n144 = local write "FGGA Shutdown"(FALSE ("FGGA Restart")) -> ()
          }
        }
      }
    }
    n145 = node-c288() -> ()  [unwired: 1 in, 1 out]
  }
  n146 = local write "Network disconnected"(FALSE ("Network disconnect")) -> ()
  n147 = while {
    shift-right: [w485] -> _
    shift-left: w11 -> [w483]
    shift-right: [w487] -> _
    shift-left: w10 -> [w488]
    shift-right: [w486] -> _
    shift-left: w12 -> [w490]
    shift-right: [w479] -> _
    shift-left: w12 -> [w481]
    shift-right: [w476] -> _
    shift-left: w11 -> [w475]
    shift-right: [w478] -> _
    shift-left: w10 -> [w480]
    stop <- FALSE stop-if-true
    w421 = ""
    w416 = "%s" ("format string")
    w607 = "%s" ("format string")
    w612 = "%s" ("format string")
    w617 = "%s" ("format string")
    w623 = "%s" ("format string")
    w629 = "%s" ("format string")
    w633 = "%s" ("format string")
    # "UDP Data Processing"
    n148 = local read "CHFGGA01"() -> (w636:string)
    n149 = local read "TWBOZO01"() -> (w611:string)
    n150 = local read "AL52CO01"() -> (w628:string)
    n151 = local read "CABOZO01"() -> (w616:string)
    n152 = local read "TEIOZO01"() -> (w622:string)
    n153 = local read "CHTSOO01"() -> (w606:string)
    n154 = local read "Ambient = OFF\nCabin = ON"() -> (w511:bool)
    n155 = Spreadsheet String To Array(delimiter (Tab)=",", format string=w633, spreadsheet string=w636, array type (2D Dbl)=string[] []) -> (array=w583:string[])
    n156 = Spreadsheet String To Array(delimiter (Tab)=",", format string=w629, spreadsheet string=w628, array type (2D Dbl)=string[] []) -> (array=w604:string[])
    n157 = Spreadsheet String To Array(delimiter (Tab)=",", format string=w617, spreadsheet string=w616, array type (2D Dbl)=string[] []) -> (array=w508:string[])
    n158 = Spreadsheet String To Array(delimiter (Tab)=",", format string=w623, spreadsheet string=w622, array type (2D Dbl)=string[] []) -> (array=w581:string[])
    n159 = Spreadsheet String To Array(delimiter (Tab)=",", format string=w612, spreadsheet string=w611, array type (2D Dbl)=string[] []) -> (array=w507:string[])
    n160 = Spreadsheet String To Array(delimiter (Tab)=",", format string=w607, spreadsheet string=w606, array type (2D Dbl)=string[] []) -> (array=w579:string[])
    n161 = Array To Spreadsheet String(delimiter (Tab)="\r", array=w583, 3:w633) -> (spreadsheet string=→"FGGA":string)
    n162 = Array To Spreadsheet String(delimiter (Tab)="\r", array=w604, 3:w629) -> (spreadsheet string=→"CO":string)
    n163 = Array To Spreadsheet String(delimiter (Tab)="\r", array=w508, 3:w617) -> (spreadsheet string=→"2B Cabin Ozone":string)
    n164 = Array To Spreadsheet String(delimiter (Tab)="\r", array=w581, 3:w623) -> (spreadsheet string=→"TEi49 Ozone":string)
    n165 = Array To Spreadsheet String(delimiter (Tab)="\r", array=w507, 3:w612) -> (spreadsheet string=→"2B Ambient Ozone":string)
    n166 = Array To Spreadsheet String(delimiter (Tab)="\r", array=w579, 3:w607) -> (spreadsheet string=→"SO2":string)
    n167 = Select(t=w508, s=w511, f=w507) -> (s? t:f=w506:string[])
    n168 = Index Array(array=w579, index #1=6 ("index"), index #2=4 ("index"), index #3=3 ("index"), index #4=7 ("index"), index #5=8 ("index"), index #6=15 ("index"), index #7=24 ("index"), index #8=29 ("index"), index #9=36 ("index"), index #10=37 ("index"), index #11=38 ("index"), index #12=39 ("index"), index #13=48 ("index"), index #14=14 ("index")) -> (element #1=w498:string, element #2=w562:string, element #3=w557:string, element #4=w550:string, element #5=w526:string, element #6=w525:string, element #7=w439:string, element #8=w438:string, element #9=w387:string, element #10=w383:string, element #11=w379:string, element #12=w377:string, element #13=w369:string, element #14=w367:string)
    n169 = Index Array(array=w506, index #1=8 ("index"), index #2=11 ("index")) -> (element #1=w500:string, element #2=w501:string)
    n170 = Index Array(array=w581, index #1=6 ("index"), index #2=4 ("index"), index #3=3 ("index"), index #4=7 ("index"), index #5=9 ("index"), index #6=14 ("index"), index #7=15 ("index")) -> (element #1=w575:string, element #2=w563:string, element #3=w558:string, element #4=w543:string, element #5=w517:string, element #6=w516:string, element #7=w515:string)
    n171 = Scan Value(string=w500, format string="%f") -> (value=→"2B Ozone concentration":dbl)  [unwired: 1 in, 1 out]
    n172 = Scan Value(string=w501, format string="%4f") -> (value=→"2B Ozone flow rate":dbl)  [unwired: 1 in, 1 out]
    n173 = Index Array(array=w583, index #1=6 ("index"), index #2=4 ("index"), index #3=3 ("index"), index #4=7 ("index"), index #5=8 ("index"), index #6=9 ("index"), index #7=10 ("index"), index #8=17 ("index"), index #9=16 ("index"), index #10=11 ("index"), index #11=12 ("index"), index #12=21 ("index"), index #13=14 ("index"), index #14=15 ("index")) -> (element #1=w577:string, element #2=w565:string, element #3=w560:string, element #4=w545:string, element #5=w463:string, element #6=w460:string, element #7=w455:string, element #8=w453:string, element #9=w450:string, element #10=w445:string, element #11=w444:string, element #12=w431:string, element #13=w397:string, element #14=w396:string)
    n174 = Index Array(array=w604, index #1=2 ("index"), index #2=27 ("index"), index #3=28 ("index"), index #4=29 ("index"), index #5=30 ("index"), index #6=31 ("index"), index #7=6 ("index"), index #8=4 ("index"), index #9=3 ("index"), index #10=8 ("index"), index #11=14 ("index"), index #12=16 ("index"), index #13=19 ("index"), index #14=12 ("index"), index #15=13 ("index"), index #16=10 ("index"), index #17=11 ("index"), index #18=15 ("index")) -> (element #1=w473:string, element #2=w547:string, element #3=w594:string, element #4=w588:string, element #5=w586:string, element #6=w587:string, element #7=w576:string, element #8=w564:string, element #9=w559:string, element #10=w548:string, element #11=w535:string, element #12=w532:string, element #13=w531:string, element #14=w493:string, element #15=w492:string, element #16=w427:string, element #17=w408:string, element #18=w402:string)
    n175 = Scan Value(string=w369, format string="%f") -> (value=→"Calibration gas cylinder \nconcentration (ppb)":dbl)  [unwired: 1 in, 1 out]
    n176 = Scan Value(string=w439, format string="%f") -> (value=→"TEI43i MFC2 Cal Flow":dbl)  [unwired: 1 in, 1 out]
    n177 = Scan Value(string=w438, format string="%f") -> (value=→"TEI43i MFC3 Sample Flow":dbl)  [unwired: 1 in, 1 out]
    n178 = Scan Value(string=w387, format string="%f") -> (value=w373:dbl)  [unwired: 1 in, 1 out]
    n179 = Scan Value(string=w383, format string="%d", default (0 dbl)=0) -> (value=w381:i32)  [unwired: 1 out]
    n180 = Scan Value(string=w367, format string="%f") -> (value=→"SO2 react pressure":dbl)  [unwired: 1 in, 1 out]
    n181 = Scan Value(string=w377, format string="%f") -> (value=→"SO2 Sensitivity":dbl)  [unwired: 1 in, 1 out]
    n182 = Scan Value(string=w379, format string="%f") -> (value=→"SO2 Zero":dbl)  [unwired: 1 in, 1 out]
    n183 = Scan Value(string=w526, format string="%f") -> (value=w374:dbl)  [unwired: 1 in, 1 out]
    n184 = Scan Value(string=w525, format string="%f") -> (value=→"TEI43C Sample Flow":dbl)  [unwired: 1 in, 1 out]
    n185 = Not Equal To 0?(x=w381) -> (x != 0?=→"mean zero\ncal status":bool)
    n186 = Decimal String To Number(string=w473) -> (number=w471:i32)  [unwired: 2 in, 1 out]
    n187 = call "Find_Data_SubVI.vi"("FGGA"=w577, "CO"=w576, "Ozone"=w575, "SO2"=w498) -> ("Output Value"=→"CPU Total %":dbl)  [unwired: 11 in]
    n188 = call "Find_Data_SubVI.vi"("FGGA"=w565, "CO"=w564, "Ozone"=w563, "SO2"=w562) -> ("Output Value"=→"MFM":dbl)  [unwired: 11 in]
    n189 = call "Find_Data_SubVI.vi"("FGGA"=w560, "CO"=w559, "Ozone"=w558, "SO2"=w557) -> ("Output Value"=w556:dbl)  [unwired: 11 in]
    n190 = call "Find_Data_SubVI.vi"("FGGA"=w545, "CO"=w548, "Ozone"=w543, "SO2"=w550) -> ("Output Value"=→"USB Disk Space Used %":dbl)  [unwired: 11 in]
    n191 = Not Equal To 0?(x=w556) -> (x != 0?=→"PTP Sync":bool)
    n192 = Add(x=w471, y=u32 2082844800) -> (x+y=w470:u32)
    n193 = Scan Value(string=w431, format string="%f") -> (value=→"MFC1 Cal Flow":dbl)  [unwired: 1 in, 1 out]
    n194 = Scan Value(string=w397, format string="%f") -> (value=w395:dbl)  [unwired: 1 in, 1 out]
    n195 = Scan Value(string=w396, format string="%f") -> (value=w393:dbl)  [unwired: 1 in, 1 out]
    n196 = Scan Value(string=w444, format string="%f") -> (value=→"Cell temperature":dbl)  [unwired: 1 in, 1 out]
    n197 = Scan Value(string=w445, format string="%f") -> (value=→"Cell pressure":dbl)  [unwired: 1 in, 1 out]
    n198 = Scan Value(string=w450, format string="%f") -> (value=→"CH4 Dry":dbl)  [unwired: 1 in, 1 out]
    n199 = Scan Value(string=w453, format string="%f") -> (value=→"CO2 Dry":dbl)  [unwired: 1 in, 1 out]
    n200 = Scan Value(string=w455, format string="%f") -> (value=→"H2O":dbl)  [unwired: 1 in, 1 out]
    n201 = Scan Value(string=w460, format string="%f") -> (value=→"CO2":dbl)  [unwired: 1 in, 1 out]
    n202 = Scan Value(string=w463, format string="%f") -> (value=→"CH4":dbl)  [unwired: 1 in, 1 out]
    n203 = local read "PRTAFT_UDP_In"() -> (w414:string)
    n204 = Scan Value(string=w587, format string="%f") -> (value=→"Std\nContent (barG)":dbl)  [unwired: 1 in, 1 out]
    n205 = Scan Value(string=w547, format string="%d", default (0 dbl)=u32 0) -> (value=w601:u32)  [unwired: 1 out]
    n206 = Scan Value(string=w586, format string="%f") -> (value=→"N2\nContent (barG)":dbl)  [unwired: 1 in, 1 out]
    n207 = Scan Value(string=w588, format string="%f") -> (value=→"CO2\nContent (barG)":dbl)  [unwired: 1 in, 1 out]
    n208 = Scan Value(string=w594, format string="%f") -> (value=→"CO2 Pressure\nDelivery (PSIA)":dbl)  [unwired: 1 in, 1 out]
    n209 = Bundle(w374, w373) -> (→"TEi43i Concentration scaled / raw":cluster{dbl, dbl})  [unwired: 1 in]
    n210 = To Time Stamp(1:w470) -> (0:w474:timestamp)
    n211 = Scan Value(string=w535, format string="%f") -> (value=→"Lamp Flow Controller":dbl)  [unwired: 1 in, 1 out]
    n212 = Scan Value(string=w408, format string="%f") -> (value=→"Raw Signal":dbl)  [unwired: 1 in, 1 out]
    n213 = Scan Value(string=w402, format string="%f") -> (value=→"Lamp Temperature":dbl)  [unwired: 1 in, 1 out]
    n214 = Scan Value(string=w427, format string="%f") -> (value=→"CO Concentration":dbl)  [unwired: 1 in, 1 out]
    n215 = Scan Value(string=w532, format string="%f") -> (value=→"Monochromator Flow":dbl)  [unwired: 1 in, 1 out]
    n216 = Scan Value(string=w531, format string="%f") -> (value=→"Fluorescence Cell Pressure":dbl)  [unwired: 1 in, 1 out]
    n217 = Not Equal To 0?(x=w601) -> (x != 0?=→"CO CAL Status":bool)
    n218 = Scan Value(string=w515, format string="%f") -> (value=→"TEI49 Sample Flow B":dbl)  [unwired: 1 in, 1 out]
    n219 = Scan Value(string=w517, format string="%f") -> (value=→"TEi49 Concentration":dbl)  [unwired: 1 in, 1 out]
    n220 = Scan Value(string=w516, format string="%f") -> (value=→"TEI49 Sample Flow A":dbl)  [unwired: 1 in, 1 out]
    n221 = Scan Value(string=w493, format string="%f") -> (value=w484:dbl)  [unwired: 1 in, 1 out]
    n222 = Scan Value(string=w492, format string="%f") -> (value=w477:dbl)  [unwired: 1 in, 1 out]
    n223 = Not Equal?(x=w483, y=w484) -> (x != y?=w489:bool)
    n224 = Not Equal?(x=w475, y=w477) -> (x != y?=w482:bool)
    n225 = Spreadsheet String To Array(delimiter (Tab)=",", format string=w416, spreadsheet string=w414, array type (2D Dbl)=string[] []) -> (array=w415:string[])
    n226 = case shown="True" w489 {
      tunnel: w490 -> [w657 w666]
      tunnel: w488 -> [w658 w665]
      tunnel: [w658 w664] -> w487
      tunnel: w474 -> [_ w660]
      tunnel: w484 -> [_ w661]
      tunnel: [w657 w663] -> w486
      tunnel: [w656 w662] -> w485
      tunnel: w484 -> [_ w662]
      tunnel: w483 -> [w656 _]
      frame False {
      }
      frame True {
        n227 = Bundle(w660, w661) -> (w659:cluster{timestamp, dbl})  [unwired: 1 in]
        n228 = Replace Array Subset(array=w666, new element=w659, index=w665) -> (w663:cluster{"time stamp":timestamp, "Y":dbl}[])
        n229 = Increment(x=w665) -> (x+1=w664:i32)
      }
    }
    "CO Sensitivity" <- w486
    n230 = case shown="True" w482 {
      tunnel: w481 -> [w646 w655]
      tunnel: w480 -> [w647 w654]
      tunnel: [w647 w653] -> w478
      tunnel: w474 -> [_ w652]
      tunnel: w477 -> [_ w651]
      tunnel: [w646 w650] -> w479
      tunnel: [w645 w649] -> w476
      tunnel: w477 -> [_ w649]
      tunnel: w475 -> [w645 _]
      frame False {
      }
      frame True {
        n231 = Bundle(w652, w651) -> (w648:cluster{timestamp, dbl})  [unwired: 1 in]
        n232 = Replace Array Subset(array=w655, new element=w648, index=w654) -> (w650:cluster{"time stamp":timestamp, "Y":dbl}[])
        n233 = Increment(x=w654) -> (x+1=w653:i32)
      }
    }
    "CO Zero" <- w479
    n234 = Array To Spreadsheet String(delimiter (Tab)="\r", array=w415, 3:w416) -> (spreadsheet string=→"PRTAFT_DLU":string)
    n235 = Index Array(array=w415, index #1=5 ("index"), index #2=19 ("index")) -> (element #1=w419:string, element #2=w417:string)
    n236 = Not Equal?(x=w419, y=w421) -> (x != y?=w420:bool)
    n237 = Not Equal?(x=w417, y=w421) -> (x != y?=w418:bool)
    n238 = Bundle(w395, w393) -> (→"Ring Down Time RDA & RDB":cluster{dbl, dbl})  [unwired: 1 in]
    n239 = case shown="False" w418 {
      tunnel: ["1" w642] -> w411
      tunnel: w417 -> [_ w642]
      frame False {
      }
      frame True {
      }
    }
    n240 = case shown="False" w420 {
      tunnel: ["XXXX" w644] -> w412
      tunnel: w419 -> [_ w644]
      frame False {
      }
      frame True {
      }
    }
    n241 = Wait (ms)(milliseconds to wait=u32 1000) -> ()  [unwired: 1 out]
    n242 = local write "WoW Flag"(w411) -> ()
    n243 = local write "Flight Number"(w412) -> ()
  }
  n244 = while {
    stop <- FALSE stop-if-true
    # "Check Connection with the cRIO continuously"
    n245 = node-c288() -> (w668:T6)  [unwired: 4 in]
    n246 = TCP Open Connection(address="192.168.101.17", remote port or service name=u16 7001) -> (connection ID=w677:refnum<k5>, error out=w678:errorcluster)  [unwired: 3 in]
    n247 = timed-loop {
      tunnel: w678 -> [w693]
      tunnel: w677 -> [w690]
      tunnel: [w686] -> w670
      tunnel: [w687] -> w674
      shift-right: [w682] -> _
      shift-left: FALSE -> [w683]
      timing: w668 -> [_]
      timing-out: [_] -> w667
      stop <- w686 stop-if-true
      # "Maintain live connecton to cRIO for connection watchdog"
      n248 = node-c288() -> ()  [unwired: 1 in, 1 out]
      n249 = TCP Write(connection ID=w690, data in="1", error in (no error)=w693, 9:2000 ("timeout ms (25000)")) -> (connection ID out=w691:refnum<k5>, bytes written=w688:i32, error out=w692:errorcluster)
      n250 = Select(t=FALSE, s=w683, f=TRUE) -> (s? t:f=w682:bool)
      "cRIO connection status" <- w682
      n251 = local write "Network disconnected"(FALSE ("Network disconnect")) -> ()
      n252 = TCP Read(connection ID=w691, bytes to read=w688, error in (no error)=w692, 9:2000 ("timeout ms (25000)")) -> (connection ID out=w687:refnum<k5>, error out=w686:errorcluster)  [unwired: 1 in, 1 out]
      n253 = node-c288() -> ()  [unwired: 1 in, 1 out]
    }
    n254 = node-c288(w667) -> ()  [unwired: 1 out]
    n255 = TCP Close Connection(connection ID=w674, error in (no error)=w670) -> (error out=w669:errorcluster)  [unwired: 1 in, 1 out]
    "Network Check error out" <- w669
    n256 = Unbundle By Name(w669) -> ("status"=w671:bool)
    "Network disconnected" <- w671
    n257 = case shown="True" w671 {
      frame False {
      }
      frame True {
        n258 = One Button Dialog(message="Connection to cRIO lost\nAll Calibration(s) will be terminated") -> ()  [unwired: 1 in, 1 out]
      }
    }
  }
  n259 = while {
    stop <- FALSE stop-if-true
    # "Preflight Sub VI Descriptions"
    n260 = Wait (ms)(milliseconds to wait=u32 500) -> ()  [unwired: 1 out]
    n261 = case shown="True" "Line Lock Setting Change" {
      frame False {
      }
      frame True {
        n262 = call "FGGA Linelock Settings Procedures.vi"() -> ()  [unwired: 12 in]
      }
    }
  }
  n263 = while {
    stop <- FALSE stop-if-true
    # "Postflight Sub VI Descriptions"
    n264 = case shown="True" "Postflight Procedures" {
      frame False {
      }
      frame True {
        n265 = call "PostFlight Procedures.vi"() -> ()  [unwired: 12 in]
      }
    }
    n266 = Wait (ms)(milliseconds to wait=u32 500) -> ()  [unwired: 1 out]
  }
  n267 = while {
    stop <- FALSE stop-if-true
    # "Preflight Sub VI Descriptions"
    n268 = case shown="True" "Prepare Gases" {
      frame False {
      }
      frame True {
        n269 = call "CO Gas Preparation.vi"() -> ()  [unwired: 12 in]
      }
    }
    n270 = Wait (ms)(milliseconds to wait=u32 500) -> ()  [unwired: 1 out]
  }
  n271 = while {
    stop <- FALSE stop-if-true
    # "Preflight Sub VI Descriptions"
    n272 = case shown="True" "Prepare SO2 Span Gas" {
      frame False {
      }
      frame True {
        n273 = call "SO2 Span Gas Preparation.vi"() -> ()  [unwired: 12 in]
      }
    }
    n274 = Wait (ms)(milliseconds to wait=u32 500) -> ()  [unwired: 1 out]
  }
  n275 = while {
    stop <- FALSE stop-if-true
    # "Preflight Sub VI Descriptions"
    n276 = case shown="True" "Prepare SO2 Zero Gas" {
      frame False {
      }
      frame True {
        n277 = call "SO2 ZeroAir Gas Preparation.vi"() -> ()  [unwired: 12 in]
      }
    }
    n278 = Wait (ms)(milliseconds to wait=u32 500) -> ()  [unwired: 1 out]
  }
  n279 = Obtain Queue(name (unnamed)="FGGA_Command", element data type=w56) -> (queue out=w6:refnum<queue>, error out=w5:errorcluster)  [unwired: 3 in, 1 out]
  n280 = while {
    stop <- FALSE stop-if-true
    # "Preflight Sub VI Descriptions"
    n281 = case shown="True" "CO Monitor Troubleshooting" {
      frame False {
      }
      frame True {
        n282 = call "CO Monitor Troubleshooting.vi"() -> ()  [unwired: 12 in]
      }
    }
    n283 = Wait (ms)(milliseconds to wait=u32 500) -> ()  [unwired: 1 out]
  }
  n284 = while {
    shift-right: [w720] -> _
    shift-left: u8 1 -> [w721]
    tunnel: w6 -> [w718]
    tunnel: w5 -> [w717]
    stop <- FALSE stop-if-true
    # "FGGA pump synchronise to WoW Wait on Wheel Flag"
    n285 = Wait (ms)(milliseconds to wait=u32 1000) -> ()  [unwired: 1 out]
    n286 = case shown="True" "FGGA pump\nsync to WoW" {
      tunnel: [w724 w729] -> w720
      tunnel: w721 -> [w724 w728]
      tunnel: w718 -> [_ w727]
      tunnel: w717 -> [_ w726]
      frame False {
      }
      frame True {
        n287 = local read "WoW Flag"() -> (w725:string)
        n288 = Scan Value(string=w725, format string="%d", default (0 dbl)=u8 0) -> (value=w729:u8)  [unwired: 1 out]
        n289 = Not Equal?(x=w729, y=w728) -> (x != y?=w732:bool)
        n290 = case shown="True" w732 {
          tunnel: w729 -> [_ w735]
          tunnel: w727 -> [_ w734]
          tunnel: w726 -> [_ w733]
          frame False {
          }
          frame True {
            n291 = Equal?(x=w735, y=u8 0) -> (x = y?=w740:bool)
            n292 = case shown="True" w740 {
              selector: w740 -> [w742 w743]
              tunnel: [w742 w743] -> w736
              frame False {
              }
              frame True {
              }
            }
            n293 = local write "Manual FGGA Pump"(w736) -> ()
            n294 = Bundle(cluster=T4 {"Message"="", "Message Data"=variant} ("Message Cluster"), "Message"="FGGA_pump", "Message Data"=w736) -> (w737:T4)
            n295 = Enqueue Element(queue=w734, element=w737, error in (no error)=w733) -> ()  [unwired: 1 in, 3 out]
          }
        }
      }
    }
  }
  n296 = while {
    stop <- FALSE stop-if-true
    # "Error Warning to User Loop"
    n297 = local read "WoW Flag"() -> (w746:string)
    n298 = Scan Value(string=w746, format string="%d", default (0 dbl)=u8 0) -> (value=w745:u8)  [unwired: 1 out]
    n299 = Wait (ms)(milliseconds to wait=u32 1000) -> ()  [unwired: 1 out]
    n300 = Equal To 0?(x=w745) -> (x = 0?=w744:bool)
    n301 = case shown="True" w744 {
      frame False {
        w751 = TRUE
        n302 = property on="Ozone Zeroing" class="Bool (strict)"("Visible"=w751) -> ()  [unwired: 2 in, 2 out]
        n303 = property on="SO2 GND Zeroing" class="Bool (strict)"("Visible"=w751) -> ()  [unwired: 2 in, 2 out]
      }
      frame True {
        w752 = FALSE ("Visible")
        n304 = local read "Fluorescence Cell Pressure"() -> (w762:dbl)
        n305 = local read "Monochromator Flow"() -> (w757:dbl)
        n306 = local read "Lamp Flow Controller"() -> (w759:dbl)
        n307 = Less?(x=w762, y=7.2) -> (x < y?=w760:bool)
        n308 = Less?(x=w757, y=29.0) -> (x < y?=w754:bool)
        n309 = Less?(x=w759, y=39.0) -> (x < y?=w755:bool)
        n310 = Compound Arithmetic op=OR(w760, w755, w754) -> (w753:bool)
        n311 = case shown="True" w753 {
          selector: w753 -> [w763 w764]
          frame False {
            n312 = property on="CO_fault" class="Bool (strict)"("Visible"=w763, "Blinking"=w763) -> ()  [unwired: 2 in, 2 out]
          }
          frame True {
            n313 = property on="CO_fault" class="Bool (strict)"("Visible"=w764, "Blinking"=w764) -> ()  [unwired: 2 in, 2 out]
          }
        }
        n314 = property on="Ozone Zeroing" class="Bool (strict)"("Visible"=w752) -> ()  [unwired: 2 in, 2 out]
        n315 = property on="SO2 GND Zeroing" class="Bool (strict)"("Visible"=w752) -> ()  [unwired: 2 in, 2 out]
      }
    }
  }
  n316 = while {
    tunnel: w6 -> [w766]
    tunnel: w5 -> [w765]
    tunnel: [w768] -> _
    tunnel: w16 -> [w767]
    stop <- FALSE stop-if-true
    # "FGGA UI Event Handler Loop"
    n317 = event shown="[9] \"Span Cal -  High Cal, CO Cal, Low Cal\": Value Change" {
      selector: _ -> [_ _ _ _ _ _ _ _ _ _ _ _ _ _ _ _ _]
      dyn-events: _ -> [_ _ _ _ _ _ _ _ _ _ _ _ _ _ _ _ _]
      timeout: _ -> [_ _ _ _ _ _ _ _ _ _ _ _ _ _ _ _ _]
      tunnel: w766 -> [w776 w780 w787 w794 w801 w809 w823 w830 w845 w986 w1237 w1307 w1377 w1433 w1547 w1646 w1653]
      tunnel: w765 -> [w775 w779 w786 w793 w800 w808 w822 w829 w844 w985 w1236 w1306 w1376 w1432 w1546 w1645 w1652]
      tunnel: [w770 w778 w785 w792 w799 w807 w821 w828 w835 w959 w1229 w1299 w1369 w1423 w1539 w1644 w1651] -> w768
      tunnel: w767 -> [_ _ _ _ _ _ _ _ _ w973 _ _ _ _ _ _ _]
      event "eV1": Value Change {
        n318 = event-data() -> ("NewVal"=w773:bool)  [unwired: 1 in]
        n319 = Bundle(cluster=T4 {"Message"="", "Message Data"=variant} ("Message Cluster"), "Message"="V1", "Message Data"=w773) -> (w771:T4)
        n320 = Enqueue Element(queue=w776, element=w771, error in (no error)=w775) -> (error out=w770:errorcluster)  [unwired: 1 in, 2 out]
      }
      event "eV2": Value Change {
        n321 = event-data() -> ("NewVal"=w777:bool)  [unwired: 1 in]
        n322 = Bundle(cluster=T4 {"Message"="", "Message Data"=variant} ("Message Cluster"), "Message"="V2", "Message Data"=w777) -> (w781:T4)
        n323 = Enqueue Element(queue=w780, element=w781, error in (no error)=w779) -> (error out=w778:errorcluster)  [unwired: 1 in, 2 out]
      }
      event "eV3": Value Change {
        n324 = event-data() -> ("NewVal"=w784:bool)  [unwired: 1 in]
        n325 = Bundle(cluster=T4 {"Message"="", "Message Data"=variant} ("Message Cluster"), "Message"="V3", "Message Data"=w784) -> (w788:T4)
        n326 = Enqueue Element(queue=w787, element=w788, error in (no error)=w786) -> (error out=w785:errorcluster)  [unwired: 1 in, 2 out]
      }
      event "eV4": Value Change {
        n327 = event-data() -> ("NewVal"=w791:bool)  [unwired: 1 in]
        n328 = Bundle(cluster=T4 {"Message"="", "Message Data"=variant} ("Message Cluster"), "Message"="V4", "Message Data"=w791) -> (w795:T4)
        n329 = Enqueue Element(queue=w794, element=w795, error in (no error)=w793) -> (error out=w792:errorcluster)  [unwired: 1 in, 2 out]
      }
      event "Manual FGGA Pump": Value Change {
        n330 = event-data() -> ("NewVal"=w798:bool)  [unwired: 1 in]
        n331 = Bundle(cluster=T4 {"Message"="", "Message Data"=variant} ("Message Cluster"), "Message"="FGGA_pump", "Message Data"=w798) -> (w802:T4)
        n332 = Enqueue Element(queue=w801, element=w802, error in (no error)=w800) -> (error out=w799:errorcluster)  [unwired: 1 in, 2 out]
      }
      event "Confirm Flight Number": Value Change {
        n333 = event-data() -> ()  [unwired: 1 in, 6 out]
        n334 = flat-sequence {
          tunnel: w808 -> [w811]
          tunnel: w809 -> [w812]
          tunnel: [w812] -> w806
          tunnel: [w811] -> w805
          tunnel: [w814] -> w807
          tunnel: w806 -> [w816]
          tunnel: w805 -> [w815]
          frame #0 {
            n335 = local write "cRIO File IO Stop\n(USB Flash Drive Unmount)"(FALSE ("cRIO File IO Stop\n(USB Flash Drive Unmount)")) -> ()
          }
          frame #1 {
            n336 = local read "Flight Number"() -> (w813:string)
            n337 = Bundle(cluster=T4 {"Message"="", "Message Data"=variant} ("Message Cluster"), "Message"="Flight Number", "Message Data"=w813) -> (w817:T4)
            n338 = Enqueue Element(queue=w816, element=w817, error in (no error)=w815) -> (error out=w814:errorcluster)  [unwired: 1 in, 2 out]
          }
        }
      }
      event "FGGA Restart": Value Change {
        n339 = event-data() -> ("NewVal"=w820:bool)  [unwired: 1 in]
        n340 = Bundle(cluster=T4 {"Message"="", "Message Data"=variant} ("Message Cluster"), "Message"="FGGA_restart", "Message Data"=w820) -> (w824:T4)
        n341 = Enqueue Element(queue=w823, element=w824, error in (no error)=w822) -> (error out=w821:errorcluster)  [unwired: 1 in, 2 out]
      }
      event "cRIO File IO Stop\n(USB Flash Drive Unmount)": Value Change {
        n342 = event-data() -> ("NewVal"=w827:bool)  [unwired: 1 in]
        n343 = Bundle(cluster=T4 {"Message"="", "Message Data"=variant} ("Message Cluster"), "Message"="Stop File Write", "Message Data"=w827) -> (w831:T4)
        n344 = Enqueue Element(queue=w830, element=w831, error in (no error)=w829) -> (error out=w828:errorcluster)  [unwired: 1 in, 2 out]
      }
      event "High Cal": Value Change {
        n345 = event-data() -> ()  [unwired: 1 in, 1 out]
        n346 = flat-sequence {
          tunnel: w845 -> [w850]
          tunnel: w844 -> [w849]
          tunnel: [w848] -> w843
          tunnel: [w847] -> w842
          tunnel: w843 -> [w866]
          tunnel: w842 -> [w865]
          tunnel: [w863] -> w841
          tunnel: [w862] -> w840
          tunnel: [w870] -> w839
          tunnel: [w871] -> w838
          tunnel: w840 -> [w875]
          tunnel: w841 -> [w874]
          tunnel: w839 -> [w928]
          tunnel: w838 -> [w927]
          tunnel: [w925] -> w837
          tunnel: [w924] -> w836
          tunnel: w837 -> [w942]
          tunnel: w836 -> [w941]
          tunnel: [w939] -> w834
          tunnel: [w947] -> w835
          tunnel: w834 -> [w947]
          frame #0 {
            w846 = TRUE
            n347 = Cluster To Array(cluster=T11 {"Message"="V2", "Message 2"="V3", "Message 3"="V4"}) -> (array=w851:string[])
            n348 = for {
              tunnel: w851 -> [w858] mode=indexing
              tunnel: w850 -> [w857]
              tunnel: w849 -> [w856]
              tunnel: [w855] -> w848
              tunnel: [w854] -> w847
              tunnel: w846 -> [w853]
              n349 = Bundle(cluster=T4 {"Message"="", "Message Data"=variant} ("Message Cluster"), "Message"=w858, "Message Data"=w853) -> (w860:T4)
              n350 = Enqueue Element(queue=w857, element=w860, error in (no error)=w856) -> (queue out=w855:refnum<queue>, error out=w854:errorcluster)  [unwired: 1 in, 1 out]
            }
            n351 = local write "eV2"(w846) -> ()
            n352 = local write "eV4"(w846) -> ()
            n353 = local write "eV3"(w846) -> ()
          }
          frame #1 {
            n354 = local read "MFC_1 User Set Value"() -> (w861:dbl)
            n355 = local write "MFC_1\nSLPM Value"(w861) -> ()
            n356 = Bundle(cluster=T4 {"Message"="", "Message Data"=variant} ("Message Cluster"), "Message"="MFC_1", "Message Data"=w861) -> (w864:T4)
            n357 = Enqueue Element(queue=w866, element=w864, error in (no error)=w865) -> (queue out=w863:refnum<queue>, error out=w862:errorcluster)  [unwired: 1 in, 1 out]
          }
          frame #2 {
            n358 = for {
              N: 45 -> [w918]
              tunnel: w875 -> [w908]
              tunnel: w874 -> [w909]
              tunnel: [w909] -> w873
              tunnel: [w908] -> w872
              tunnel: [w907] -> w869
              i -> [w917]
              stop <- w907 stop-if-true
              n359 = Subtract(x=w918, y=w917) -> (x-y=w916:i32)
              n360 = Decrement(x=w916) -> (x-1=w915:i32)
              n361 = local read "FGGA Calibration Abort"() -> (w912:bool)
              n362 = case shown="True" w912 {
                selector: w912 -> [w921 _]
                tunnel: [w921 w922] -> w910
                frame False {
                }
                frame True {
                  n363 = Two Button Dialog(message="Are you sure to abort FGGA High Cal?") -> (T button?=w922:bool)  [unwired: 2 in]
                }
              }
              n364 = Wait (ms)(milliseconds to wait=u32 1000) -> ()  [unwired: 1 out]
              n365 = local read "Network disconnected"() -> (w911:bool)
              n366 = Or(x=w911, y=w910) -> (x .or. y?=w907:bool)
              n367 = case shown="False" w910 {
                selector: w910 -> [w920 _]
                frame False {
                  n368 = local write "FGGA Calibration Abort"(w920) -> ()
                }
                frame True {
                }
              }
              n369 = Select(t=0, s=w907, f=w915) -> (s? t:f=→"High Cal\nFlush Time Remain (sec)":i32)
            }
            n370 = case shown="False" w869 {
              tunnel: w873 -> [w882 w906]
              tunnel: w872 -> [w881 w905]
              tunnel: [w878 w905] -> w871
              tunnel: [w877 w906] -> w870
              frame False {
                w883 = TRUE
                # "Carry on if connection to cRIO is made\nor calibration not abort"
                n371 = Bundle(cluster=T4 {"Message"="", "Message Data"=variant} ("Message Cluster"), "Message"="V1", "Message Data"=w883) -> (w884:T4)
                n372 = local write "eV1"(w883) -> ()
                n373 = Enqueue Element(queue=w882, element=w884, error in (no error)=w881) -> (queue out=w879:refnum<queue>, error out=w880:errorcluster)  [unwired: 1 in, 1 out]
                n374 = for {
                  N: 60 -> [w899]
                  tunnel: w880 -> [w889]
                  tunnel: w879 -> [w888]
                  tunnel: [w889] -> w878
                  tunnel: [w888] -> w877
                  i -> [w898]
                  stop <- w890 stop-if-true
                  n375 = local read "FGGA Calibration Abort"() -> (w893:bool)
                  n376 = Subtract(x=w899, y=w898) -> (x-y=w897:i32)
                  n377 = case shown="True" w893 {
                    selector: w893 -> [w902 _]
                    tunnel: [w902 w903] -> w891
                    frame False {
                    }
                    frame True {
                      n378 = Two Button Dialog(message="Are you sure to abort FGGA High Cal?") -> (T button?=w903:bool)  [unwired: 2 in]
                    }
                  }
                  n379 = local read "Network disconnected"() -> (w892:bool)
                  n380 = Wait (ms)(milliseconds to wait=u32 1000) -> ()  [unwired: 1 out]
                  n381 = Decrement(x=w897) -> (x-1=w894:i32)
                  n382 = Or(x=w892, y=w891) -> (x .or. y?=w890:bool)
                  n383 = case shown="False" w891 {
                    selector: w891 -> [w901 _]
                    frame False {
                      n384 = local write "FGGA Calibration Abort"(w901) -> ()
                    }
                    frame True {
                    }
                  }
                  n385 = Select(t=0, s=w890, f=w894) -> (s? t:f=→"High Cal\nCal Time Remain (sec)":i32)
                }
              }
              frame True {
              }
            }
          }
          frame #3 {
            w926 = FALSE
            n386 = Cluster To Array(cluster=T12 {"Message"="V2", "Message 2"="V3", "Message 3"="V4", "Message 4"="V1"}) -> (array=w929:string[])
            n387 = for {
              tunnel: w929 -> [w936] mode=indexing
              tunnel: [w935] -> w925
              tunnel: [w934] -> w924
              tunnel: w926 -> [w933]
              tunnel: w928 -> [w932]
              tunnel: w927 -> [w931]
              n388 = Bundle(cluster=T4 {"Message"="", "Message Data"=variant} ("Message Cluster"), "Message"=w936, "Message Data"=w933) -> (w938:T4)
              n389 = Enqueue Element(queue=w932, element=w938, error in (no error)=w931) -> (queue out=w935:refnum<queue>, error out=w934:errorcluster)  [unwired: 1 in, 1 out]
            }
            n390 = local write "eV2"(w926) -> ()
            n391 = local write "eV4"(w926) -> ()
            n392 = local write "eV3"(w926) -> ()
            n393 = local write "eV1"(w926) -> ()
          }
          frame #4 {
            w940 = 0.0 ("MFC_1\nSLPM Value")
            n394 = local write "MFC_1\nSLPM Value"(w940) -> ()
            n395 = Bundle(cluster=T4 {"Message"="", "Message Data"=variant} ("Message Cluster"), "Message"="MFC_1", "Message Data"=w940) -> (w944:T4)
            n396 = Enqueue Element(queue=w942, element=w944, error in (no error)=w941) -> (error out=w939:errorcluster)  [unwired: 1 in, 2 out]
          }
          frame #5 {
            w946 = FALSE ("High Cal")
            n397 = local write "High Cal"(w946) -> ()
            n398 = local write "FGGA Calibration Abort"(w946) -> ()
          }
        }
      }
      event "Span Cal - \nHigh Cal, CO Cal, Low Cal": Value Change {
        n399 = event-data() -> ()  [unwired: 1 in, 1 out]
        n400 = flat-sequence {
          tunnel: w986 -> [w992]
          tunnel: w985 -> [w991]
          tunnel: [w990] -> w984
          tunnel: [w989] -> w983
          tunnel: w984 -> [w1008]
          tunnel: w983 -> [w1007]
          tunnel: [w1005] -> w981
          tunnel: [w1004] -> w979
          tunnel: [w1014] -> w982
          tunnel: w981 -> [w1014]
          tunnel: [w1013] -> w980
          tunnel: w979 -> [w1013]
          tunnel: [w1011] -> w958
          tunnel: [w1011] -> w955
          tunnel: w982 -> [w1032]
          tunnel: w980 -> [w1033]
          tunnel: [w1033] -> w965
          tunnel: w973 -> [w1034]
          tunnel: [w1034] -> w963
          tunnel: [w1032] -> w961
          tunnel: w958 -> [w1031]
          tunnel: [w1030] -> w956
          tunnel: w955 -> [w1030]
          tunnel: w965 -> [w1044]
          tunnel: [w1044] -> w964
          tunnel: w963 -> [w1043]
          tunnel: [w1043] -> w962
          tunnel: w961 -> [w1041]
          tunnel: [w1041] -> w960
          tunnel: [w1040] -> w957
          tunnel: w956 -> [w1040]
          tunnel: [w1048] -> w978
          tunnel: [w1047] -> w977
          tunnel: w960 -> [w1049]
          tunnel: w962 -> [w1055]
          tunnel: w964 -> [w1050]
          tunnel: w957 -> [w1046]
          tunnel: [w1046] -> w951
          tunnel: [w1045] -> w948
          tunnel: w978 -> [w1094]
          tunnel: w977 -> [w1093]
          tunnel: [w1091] -> w976
          tunnel: [w1090] -> w975
          tunnel: [w1089] -> w952
          tunnel: w951 -> [w1089]
          tunnel: [w1088] -> w949
          tunnel: w948 -> [w1088]
          tunnel: w976 -> [w1111]
          tunnel: w975 -> [w1110]
          tunnel: [w1108] -> w974
          tunnel: [w1107] -> w970
          tunnel: [w1106] -> w953
          tunnel: w952 -> [w1106]
          tunnel: [w1105] -> w950
          tunnel: w949 -> [w1105]
          tunnel: w974 -> [w1120]
          tunnel: [w1120] -> w972
          tunnel: [w1118] -> w971
          tunnel: w970 -> [w1118]
          tunnel: [w1117] -> w954
          tunnel: w953 -> [w1116]
          tunnel: w950 -> [w1115]
          tunnel: [w1125] -> w969
          tunnel: [w1124] -> w968
          tunnel: w972 -> [w1122]
          tunnel: w971 -> [w1123]
          tunnel: w954 -> [w1121]
          tunnel: w969 -> [w1207]
          tunnel: w968 -> [w1206]
          tunnel: [w1204] -> w967
          tunnel: [w1203] -> w966
          tunnel: w967 -> [w1222]
          tunnel: w966 -> [w1221]
          tunnel: [w1219] -> w959
          frame #0 {
            w988 = TRUE
            n401 = Cluster To Array(cluster=T11 {"Message"="V2", "Message 2"="V3", "Message 3"="V4"}) -> (array=w993:string[])
            n402 = for {
              tunnel: w993 -> [w1000] mode=indexing
              tunnel: w992 -> [w999]
              tunnel: w991 -> [w998]
              tunnel: [w997] -> w990
              tunnel: [w996] -> w989
              tunnel: w988 -> [w995]
              n403 = Bundle(cluster=T4 {"Message"="", "Message Data"=variant} ("Message Cluster"), "Message"=w1000, "Message Data"=w995) -> (w1002:T4)
              n404 = Enqueue Element(queue=w999, element=w1002, error in (no error)=w998) -> (queue out=w997:refnum<queue>, error out=w996:errorcluster)  [unwired: 1 in, 1 out]
            }
            n405 = local write "High Cal"(TRUE ("High Cal")) -> ()
            n406 = local write "eV2"(w988) -> ()
            n407 = local write "eV4"(w988) -> ()
            n408 = local write "eV3"(w988) -> ()
          }
          frame #1 {
            n409 = local read "MFC_1 User Set Value"() -> (w1003:dbl)
            n410 = local write "MFC_1\nSLPM Value"(w1003) -> ()
            n411 = Bundle(cluster=T4 {"Message"="", "Message Data"=variant} ("Message Cluster"), "Message"="MFC_1", "Message Data"=w1003) -> (w1006:T4)
            n412 = Enqueue Element(queue=w1008, element=w1006, error in (no error)=w1007) -> (queue out=w1005:refnum<queue>, error out=w1004:errorcluster)  [unwired: 1 in, 1 out]
          }
          frame #2 {
            n413 = for {
              N: 45 -> [w1024]
              tunnel: [w1016] -> w1011
              i -> [w1023]
              stop <- w1016 stop-if-true
              n414 = local read "FGGA Calibration Abort"() -> (w1017:bool)
              n415 = case shown="True" w1017 {
                selector: w1017 -> [w1027 _]
                tunnel: [w1027 w1028] -> w1015
                frame False {
                }
                frame True {
                  n416 = Two Button Dialog(message="Are you sure to abort FGGA Span Cal?") -> (T button?=w1028:bool)  [unwired: 2 in]
                }
              }
              n417 = local read "Network disconnected"() -> (w1018:bool)
              n418 = Subtract(x=w1024, y=w1023) -> (x-y=w1022:i32)
              n419 = Decrement(x=w1022) -> (x-1=w1020:i32)
              n420 = Wait (ms)(milliseconds to wait=u32 1000) -> ()  [unwired: 1 out]
              n421 = Or(x=w1018, y=w1015) -> (x .or. y?=w1016:bool)
              n422 = case shown="False" w1015 {
                selector: w1015 -> [w1026 _]
                frame False {
                  n423 = local write "FGGA Calibration Abort"(w1026) -> ()
                }
                frame True {
                }
              }
              n424 = Select(t=0, s=w1016, f=w1020) -> (s? t:f=w1019:i32)
              n425 = local write "High Cal\nFlush Time Remain (sec)"(w1019) -> ()
            }
          }
          frame #3 {
            n426 = case shown="False" w1031 {
              tunnel: w1034 -> [w1035 _]
              frame False {
                # "CO Cal if no network\ndisconnect or abort cal"
                n427 = Bundle(cluster=T4 {"Message"="", "Message Data"=variant} ("Message Cluster"), "Message"="CO CAL", "Message Data"=TRUE) -> (w1037:T4)
                n428 = Enqueue Element(queue=w1035, element=w1037) -> ()  [unwired: 2 in, 3 out]
              }
              frame True {
              }
            }
          }
          frame #4 {
            # "To Ensure\nCO CAL\nis certain"
            n429 = Wait (ms)(milliseconds to wait=u32 1000) -> ()  [unwired: 1 out]
          }
          frame #5 {
            n430 = Bundle(cluster=T4 {"Message"="", "Message Data"=variant} ("Message Cluster"), "Message"="CO CAL", "Message Data"=FALSE) -> (w1051:T4)
            n431 = Enqueue Element(queue=w1055, element=w1051) -> ()  [unwired: 2 in, 3 out]
            n432 = case shown="False" w1046 {
              selector: w1046 -> [_ w1085]
              tunnel: w1050 -> [w1062 w1086]
              tunnel: w1049 -> [w1061 w1087]
              tunnel: [w1058 w1087] -> w1048
              tunnel: [w1057 w1086] -> w1047
              tunnel: [w1056 w1085] -> w1045
              frame False {
                w1066 = TRUE
                # "Carry on if connection to cRIO is made\nor calibration not abort"
                n433 = Bundle(cluster=T4 {"Message"="", "Message Data"=variant} ("Message Cluster"), "Message"="V1", "Message Data"=w1066) -> (w1065:T4)
                n434 = local write "eV1"(w1066) -> ()
                n435 = Enqueue Element(queue=w1061, element=w1065, error in (no error)=w1062) -> (queue out=w1060:refnum<queue>, error out=w1059:errorcluster)  [unwired: 1 in, 1 out]
                n436 = for {
                  N: 60 -> [w1079]
                  tunnel: w1060 -> [w1070]
                  tunnel: w1059 -> [w1069]
                  tunnel: [w1070] -> w1058
                  tunnel: [w1069] -> w1057
                  tunnel: [w1068] -> w1056
                  i -> [w1078]
                  stop <- w1068 stop-if-true
                  n437 = local read "FGGA Calibration Abort"() -> (w1073:bool)
                  n438 = case shown="True" w1073 {
                    selector: w1073 -> [w1082 _]
                    tunnel: [w1082 w1083] -> w1071
                    frame False {
                    }
                    frame True {
                      n439 = Two Button Dialog(message="Are you sure to abort FGGA Span Cal?") -> (T button?=w1083:bool)  [unwired: 2 in]
                    }
                  }
                  n440 = Subtract(x=w1079, y=w1078) -> (x-y=w1077:i32)
                  n441 = Decrement(x=w1077) -> (x-1=w1075:i32)
                  n442 = Wait (ms)(milliseconds to wait=u32 1000) -> ()  [unwired: 1 out]
                  n443 = local read "Network disconnected"() -> (w1072:bool)
                  n444 = Or(x=w1072, y=w1071) -> (x .or. y?=w1068:bool)
                  n445 = Select(t=0, s=w1068, f=w1075) -> (s? t:f=w1074:i32)
                  n446 = local write "High Cal\nCal Time Remain (sec)"(w1074) -> ()
                  n447 = case shown="False" w1071 {
                    selector: w1071 -> [w1081 _]
                    frame False {
                      n448 = local write "FGGA Calibration Abort"(w1081) -> ()
                    }
                    frame True {
                    }
                  }
                }
              }
              frame True {
              }
            }
          }
          frame #6 {
            w1092 = FALSE
            n449 = Cluster To Array(cluster=T12 {"Message"="V2", "Message 2"="V3", "Message 3"="V4", "Message 4"="V1"}) -> (array=w1095:string[])
            n450 = for {
              tunnel: w1095 -> [w1102] mode=indexing
              tunnel: [w1101] -> w1091
              tunnel: [w1100] -> w1090
              tunnel: w1092 -> [w1099]
              tunnel: w1094 -> [w1098]
              tunnel: w1093 -> [w1097]
              n451 = Bundle(cluster=T4 {"Message"="", "Message Data"=variant} ("Message Cluster"), "Message"=w1102, "Message Data"=w1099) -> (w1104:T4)
              n452 = Enqueue Element(queue=w1098, element=w1104, error in (no error)=w1097) -> (queue out=w1101:refnum<queue>, error out=w1100:errorcluster)  [unwired: 1 in, 1 out]
            }
            n453 = local write "eV2"(w1092) -> ()
            n454 = local write "eV4"(w1092) -> ()
            n455 = local write "eV3"(w1092) -> ()
            n456 = local write "eV1"(w1092) -> ()
          }
          frame #7 {
            w1109 = 0.0 ("MFC_1\nSLPM Value")
            n457 = local write "MFC_1\nSLPM Value"(w1109) -> ()
            n458 = Bundle(cluster=T4 {"Message"="", "Message Data"=variant} ("Message Cluster"), "Message"="MFC_1", "Message Data"=w1109) -> (w1113:T4)
            n459 = Enqueue Element(queue=w1111, element=w1113, error in (no error)=w1110) -> (queue out=w1107:refnum<queue>, error out=w1108:errorcluster)  [unwired: 1 in, 1 out]
          }
          frame #8 {
            n460 = local write "High Cal"(FALSE ("High Cal")) -> ()
            n461 = Or(x=w1116, y=w1115) -> (x .or. y?=w1117:bool)
          }
          frame #9 {
            n462 = case shown="False" w1121 {
              tunnel: [w1128 w1202] -> w1125
              tunnel: [w1127 w1201] -> w1124
              tunnel: w1123 -> [w1137 w1202]
              tunnel: w1122 -> [w1135 w1201]
              frame False {
                w1133 = TRUE
                n463 = Cluster To Array(cluster=cluster{"Message":string, "Message 3":string} {"Message"="V2", "Message 3"="V4"}) -> (array=w1138:string[])
                n464 = for {
                  tunnel: w1138 -> [w1181] mode=indexing
                  tunnel: w1137 -> [w1180]
                  tunnel: [w1179] -> w1139
                  tunnel: [w1178] -> w1141
                  tunnel: w1133 -> [w1177]
                  tunnel: w1135 -> [w1176]
                  n465 = Bundle(cluster=T4 {"Message"="", "Message Data"=variant} ("Message Cluster"), "Message"=w1181, "Message Data"=w1177) -> (w1183:T4)
                  n466 = Enqueue Element(queue=w1180, element=w1183, error in (no error)=w1176) -> (queue out=w1179:refnum<queue>, error out=w1178:errorcluster)  [unwired: 1 in, 1 out]
                }
                n467 = local write "eV4"(w1133) -> ()
                n468 = local write "eV2"(w1133) -> ()
                n469 = local write "Low Cal"(TRUE ("Low Cal")) -> ()
                n470 = local read "MFC_1 User Set Value"() -> (w1142:dbl)
                n471 = local write "MFC_1\nSLPM Value"(w1142) -> ()
                n472 = Bundle(cluster=T4 {"Message"="", "Message Data"=variant} ("Message Cluster"), "Message"="MFC_1", "Message Data"=w1142) -> (w1143:T4)
                n473 = Enqueue Element(queue=w1139, element=w1143, error in (no error)=w1141) -> (queue out=w1132:refnum<queue>, error out=w1130:errorcluster)  [unwired: 1 in, 1 out]
                n474 = for {
                  N: 45 -> [w1195]
                  tunnel: [w1186] -> w1131
                  tunnel: w1132 -> [w1186]
                  tunnel: [w1185] -> w1129
                  tunnel: w1130 -> [w1185]
                  tunnel: [w1184] -> w1126
                  i -> [w1194]
                  stop <- w1184 stop-if-true
                  n475 = local read "FGGA Calibration Abort"() -> (w1189:bool)
                  n476 = case shown="True" w1189 {
                    selector: w1189 -> [w1198 _]
                    tunnel: [w1198 w1199] -> w1187
                    frame False {
                    }
                    frame True {
                      n477 = Two Button Dialog(message="Are you sure to abort FGGA Span Cal?") -> (T button?=w1199:bool)  [unwired: 2 in]
                    }
                  }
                  n478 = Subtract(x=w1195, y=w1194) -> (x-y=w1193:i32)
                  n479 = Decrement(x=w1193) -> (x-1=w1190:i32)
                  n480 = Wait (ms)(milliseconds to wait=u32 1000) -> ()  [unwired: 1 out]
                  n481 = local read "Network disconnected"() -> (w1188:bool)
                  n482 = Or(x=w1188, y=w1187) -> (x .or. y?=w1184:bool)
                  n483 = Select(t=0, s=w1184, f=w1190) -> (s? t:f=w1191:i32)
                  n484 = local write "Low Cal\nFlush Time Remain (sec)"(w1191) -> ()
                  n485 = case shown="False" w1187 {
                    selector: w1187 -> [w1197 _]
                    frame False {
                      n486 = local write "FGGA Calibration Abort"(w1197) -> ()
                    }
                    frame True {
                    }
                  }
                }
                n487 = case shown="False" w1126 {
                  tunnel: w1131 -> [w1151 w1175]
                  tunnel: w1129 -> [w1150 w1174]
                  tunnel: [w1148 w1175] -> w1128
                  tunnel: [w1146 w1174] -> w1127
                  frame False {
                    w1152 = TRUE
                    n488 = local write "eV1"(w1152) -> ()
                    n489 = Bundle(cluster=T4 {"Message"="", "Message Data"=variant} ("Message Cluster"), "Message"="V1", "Message Data"=w1152) -> (w1154:T4)
                    n490 = Enqueue Element(queue=w1151, element=w1154, error in (no error)=w1150) -> (queue out=w1149:refnum<queue>, error out=w1147:errorcluster)  [unwired: 1 in, 1 out]
                    n491 = for {
                      N: 60 -> [w1168]
                      tunnel: [w1158] -> w1148
                      tunnel: w1149 -> [w1158]
                      tunnel: w1147 -> [w1157]
                      tunnel: [w1157] -> w1146
                      i -> [w1167]
                      stop <- w1159 stop-if-true
                      n492 = local read "FGGA Calibration Abort"() -> (w1162:bool)
                      n493 = case shown="True" w1162 {
                        selector: w1162 -> [w1171 _]
                        tunnel: [w1171 w1172] -> w1160
                        frame False {
                        }
                        frame True {
                          n494 = Two Button Dialog(message="Are you sure to abort FGGA Span Cal?") -> (T button?=w1172:bool)  [unwired: 2 in]
                        }
                      }
                      n495 = Wait (ms)(milliseconds to wait=u32 1000) -> ()  [unwired: 1 out]
                      n496 = local read "Network disconnected"() -> (w1161:bool)
                      n497 = Subtract(x=w1168, y=w1167) -> (x-y=w1166:i32)
                      n498 = Decrement(x=w1166) -> (x-1=w1163:i32)
                      n499 = Or(x=w1161, y=w1160) -> (x .or. y?=w1159:bool)
                      n500 = Select(t=0, s=w1159, f=w1163) -> (s? t:f=w1164:i32)
                      n501 = local write "Low Cal\nCal Time Remain (sec)"(w1164) -> ()
                      n502 = case shown="False" w1160 {
                        selector: w1160 -> [w1170 _]
                        frame False {
                          n503 = local write "FGGA Calibration Abort"(w1170) -> ()
                        }
                        frame True {
                        }
                      }
                    }
                  }
                  frame True {
                    # "Ignore Cal if connection problem or abort button pressed"
                  }
                }
              }
              frame True {
                # "Ignore Cal if connection problem or abort button pressed"
              }
            }
          }
          frame #10 {
            w1205 = FALSE
            n504 = Cluster To Array(cluster=T13 {"Message"="V2", "Message 3"="V4", "Message 4"="V1"}) -> (array=w1208:string[])
            n505 = local write "eV1"(w1205) -> ()
            n506 = local write "eV2"(w1205) -> ()
            n507 = local write "eV4"(w1205) -> ()
            n508 = for {
              tunnel: w1208 -> [w1215] mode=indexing
              tunnel: [w1214] -> w1204
              tunnel: [w1213] -> w1203
              tunnel: w1205 -> [w1212]
              tunnel: w1207 -> [w1211]
              tunnel: w1206 -> [w1210]
              n509 = Bundle(cluster=T4 {"Message"="", "Message Data"=variant} ("Message Cluster"), "Message"=w1215, "Message Data"=w1212) -> (w1217:T4)
              n510 = Enqueue Element(queue=w1211, element=w1217, error in (no error)=w1210) -> (queue out=w1214:refnum<queue>, error out=w1213:errorcluster)  [unwired: 1 in, 1 out]
            }
          }
          frame #11 {
            w1218 = FALSE
            w1220 = 0.0 ("MFC_1\nSLPM Value")
            n511 = local write "MFC_1\nSLPM Value"(w1220) -> ()
            n512 = local write "Span Cal - \nHigh Cal, CO Cal, Low Cal"(w1218) -> ()
            n513 = local write "FGGA Calibration Abort"(w1218) -> ()
            n514 = local write "Low Cal"(w1218) -> ()
            n515 = Bundle(cluster=T4 {"Message"="", "Message Data"=variant} ("Message Cluster"), "Message"="MFC_1", "Message Data"=w1220) -> (w1224:T4)
            n516 = Enqueue Element(queue=w1222, element=w1224, error in (no error)=w1221) -> (error out=w1219:errorcluster)  [unwired: 1 in, 2 out]
          }
        }
      }
      event "Flush High Tank": Value Change {
        n517 = event-data() -> ()  [unwired: 1 in, 6 out]
        n518 = flat-sequence {
          tunnel: w1237 -> [w1242]
          tunnel: w1236 -> [w1241]
          tunnel: [w1240] -> w1235
          tunnel: [w1239] -> w1234
          tunnel: w1235 -> [w1258]
          tunnel: w1234 -> [w1257]
          tunnel: [w1255] -> w1233
          tunnel: [w1254] -> w1232
          tunnel: w1233 -> [w1261]
          tunnel: w1232 -> [w1262]
          tunnel: [w1262] -> w1227
          tunnel: [w1261] -> w1226
          tunnel: [w1275] -> w1231
          tunnel: [w1274] -> w1230
          tunnel: w1227 -> [w1273]
          tunnel: w1226 -> [w1272]
          tunnel: w1231 -> [w1290]
          tunnel: w1230 -> [w1289]
          tunnel: [w1287] -> w1228
          tunnel: [w1295] -> w1229
          tunnel: w1228 -> [w1295]
          frame #0 {
            w1238 = TRUE
            n519 = Cluster To Array(cluster=T11 {"Message"="V2", "Message 2"="V3", "Message 3"="V4"}) -> (array=w1243:string[])
            n520 = for {
              tunnel: w1243 -> [w1250] mode=indexing
              tunnel: w1242 -> [w1249]
              tunnel: w1241 -> [w1248]
              tunnel: [w1247] -> w1240
              tunnel: [w1246] -> w1239
              tunnel: w1238 -> [w1245]
              n521 = Bundle(cluster=T4 {"Message"="", "Message Data"=variant} ("Message Cluster"), "Message"=w1250, "Message Data"=w1245) -> (w1252:T4)
              n522 = Enqueue Element(queue=w1249, element=w1252, error in (no error)=w1248) -> (queue out=w1247:refnum<queue>, error out=w1246:errorcluster)  [unwired: 1 in, 1 out]
            }
            n523 = local write "eV2"(w1238) -> ()
            n524 = local write "eV4"(w1238) -> ()
            n525 = local write "eV3"(w1238) -> ()
          }
          frame #1 {
            n526 = local read "MFC_1 User Set Value"() -> (w1253:dbl)
            n527 = local write "MFC_1\nSLPM Value"(w1253) -> ()
            n528 = Bundle(cluster=T4 {"Message"="", "Message Data"=variant} ("Message Cluster"), "Message"="MFC_1", "Message Data"=w1253) -> (w1256:T4)
            n529 = Enqueue Element(queue=w1258, element=w1256, error in (no error)=w1257) -> (queue out=w1255:refnum<queue>, error out=w1254:errorcluster)  [unwired: 1 in, 1 out]
          }
          frame #2 {
            n530 = for {
              N: 15 -> [w1270]
              i -> [w1269]
              stop <- w1265 stop-if-true
              n531 = Subtract(x=w1270, y=w1269) -> (x-y=w1268:i32)
              n532 = Decrement(x=w1268) -> (x-1=w1266:i32)
              n533 = local read "Network disconnected"() -> (w1265:bool)
              n534 = Wait (ms)(milliseconds to wait=u32 1000) -> ()  [unwired: 1 out]
              n535 = Select(t=0, s=w1265, f=w1266) -> (s? t:f=→"Flush High Tank\nTime Remain (sec)":i32)
            }
          }
          frame #3 {
            w1276 = FALSE
            n536 = Cluster To Array(cluster=T11 {"Message"="V2", "Message 2"="V3", "Message 3"="V4"}) -> (array=w1277:string[])
            n537 = for {
              tunnel: w1277 -> [w1284] mode=indexing
              tunnel: [w1283] -> w1275
              tunnel: [w1282] -> w1274
              tunnel: w1276 -> [w1281]
              tunnel: w1272 -> [w1280]
              tunnel: w1273 -> [w1279]
              n538 = Bundle(cluster=T4 {"Message"="", "Message Data"=variant} ("Message Cluster"), "Message"=w1284, "Message Data"=w1281) -> (w1286:T4)
              n539 = Enqueue Element(queue=w1280, element=w1286, error in (no error)=w1279) -> (queue out=w1283:refnum<queue>, error out=w1282:errorcluster)  [unwired: 1 in, 1 out]
            }
            n540 = local write "eV2"(w1276) -> ()
            n541 = local write "eV4"(w1276) -> ()
            n542 = local write "eV3"(w1276) -> ()
          }
          frame #4 {
            w1288 = 0.0 ("MFC_1\nSLPM Value")
            n543 = local write "MFC_1\nSLPM Value"(w1288) -> ()
            n544 = Bundle(cluster=T4 {"Message"="", "Message Data"=variant} ("Message Cluster"), "Message"="MFC_1", "Message Data"=w1288) -> (w1292:T4)
            n545 = Enqueue Element(queue=w1290, element=w1292, error in (no error)=w1289) -> (error out=w1287:errorcluster)  [unwired: 1 in, 2 out]
          }
          frame #5 {
            n546 = local write "Flush High Tank"(FALSE ("High Cal")) -> ()
          }
        }
      }
      event "Flush Low Tank": Value Change {
        n547 = event-data() -> ()  [unwired: 1 in, 1 out]
        n548 = flat-sequence {
          tunnel: w1307 -> [w1312]
          tunnel: w1306 -> [w1311]
          tunnel: [w1310] -> w1305
          tunnel: [w1309] -> w1304
          tunnel: w1305 -> [w1328]
          tunnel: w1304 -> [w1327]
          tunnel: [w1325] -> w1303
          tunnel: [w1324] -> w1302
          tunnel: w1303 -> [w1331]
          tunnel: w1302 -> [w1332]
          tunnel: [w1332] -> w1297
          tunnel: [w1331] -> w1296
          tunnel: [w1345] -> w1301
          tunnel: [w1344] -> w1300
          tunnel: w1297 -> [w1343]
          tunnel: w1296 -> [w1342]
          tunnel: w1301 -> [w1360]
          tunnel: w1300 -> [w1359]
          tunnel: [w1357] -> w1298
          tunnel: [w1365] -> w1299
          tunnel: w1298 -> [w1365]
          frame #0 {
            w1308 = TRUE
            n549 = Cluster To Array(cluster=cluster{"Message":string, "Message 3":string} {"Message"="V2", "Message 3"="V4"}) -> (array=w1313:string[])
            n550 = for {
              tunnel: w1313 -> [w1320] mode=indexing
              tunnel: w1312 -> [w1319]
              tunnel: w1311 -> [w1318]
              tunnel: [w1317] -> w1310
              tunnel: [w1316] -> w1309
              tunnel: w1308 -> [w1315]
              n551 = Bundle(cluster=T4 {"Message"="", "Message Data"=variant} ("Message Cluster"), "Message"=w1320, "Message Data"=w1315) -> (w1322:T4)
              n552 = Enqueue Element(queue=w1319, element=w1322, error in (no error)=w1318) -> (queue out=w1317:refnum<queue>, error out=w1316:errorcluster)  [unwired: 1 in, 1 out]
            }
            n553 = local write "eV2"(w1308) -> ()
            n554 = local write "eV4"(w1308) -> ()
          }
          frame #1 {
            n555 = local read "MFC_1 User Set Value"() -> (w1323:dbl)
            n556 = local write "MFC_1\nSLPM Value"(w1323) -> ()
            n557 = Bundle(cluster=T4 {"Message"="", "Message Data"=variant} ("Message Cluster"), "Message"="MFC_1", "Message Data"=w1323) -> (w1326:T4)
            n558 = Enqueue Element(queue=w1328, element=w1326, error in (no error)=w1327) -> (queue out=w1325:refnum<queue>, error out=w1324:errorcluster)  [unwired: 1 in, 1 out]
          }
          frame #2 {
            n559 = for {
              N: 15 -> [w1340]
              i -> [w1339]
              stop <- w1334 stop-if-true
              n560 = Subtract(x=w1340, y=w1339) -> (x-y=w1338:i32)
              n561 = Decrement(x=w1338) -> (x-1=w1335:i32)
              n562 = local read "Network disconnected"() -> (w1334:bool)
              n563 = Wait (ms)(milliseconds to wait=u32 1000) -> ()  [unwired: 1 out]
              n564 = Select(t=0, s=w1334, f=w1335) -> (s? t:f=→"Flush Low Tank\nTime Remain (sec)":i32)
            }
          }
          frame #3 {
            w1346 = FALSE
            n565 = Cluster To Array(cluster=cluster{"Message":string, "Message 3":string} {"Message"="V2", "Message 3"="V4"}) -> (array=w1347:string[])
            n566 = for {
              tunnel: w1347 -> [w1354] mode=indexing
              tunnel: [w1353] -> w1345
              tunnel: [w1352] -> w1344
              tunnel: w1346 -> [w1351]
              tunnel: w1342 -> [w1350]
              tunnel: w1343 -> [w1349]
              n567 = Bundle(cluster=T4 {"Message"="", "Message Data"=variant} ("Message Cluster"), "Message"=w1354, "Message Data"=w1351) -> (w1356:T4)
              n568 = Enqueue Element(queue=w1350, element=w1356, error in (no error)=w1349) -> (queue out=w1353:refnum<queue>, error out=w1352:errorcluster)  [unwired: 1 in, 1 out]
            }
            n569 = local write "eV2"(w1346) -> ()
            n570 = local write "eV4"(w1346) -> ()
          }
          frame #4 {
            w1358 = 0.0 ("MFC_1\nSLPM Value")
            n571 = local write "MFC_1\nSLPM Value"(w1358) -> ()
            n572 = Bundle(cluster=T4 {"Message"="", "Message Data"=variant} ("Message Cluster"), "Message"="MFC_1", "Message Data"=w1358) -> (w1362:T4)
            n573 = Enqueue Element(queue=w1360, element=w1362, error in (no error)=w1359) -> (error out=w1357:errorcluster)  [unwired: 1 in, 2 out]
          }
          frame #5 {
            n574 = local write "Flush Low Tank"(FALSE ("High Cal")) -> ()
          }
        }
      }
      event "Flush Target Tank": Value Change {
        n575 = event-data() -> ()  [unwired: 1 in, 1 out]
        n576 = flat-sequence {
          tunnel: w1377 -> [w1385]
          tunnel: w1376 -> [w1384]
          tunnel: [w1383] -> w1375
          tunnel: [w1382] -> w1374
          tunnel: w1375 -> [w1391]
          tunnel: w1374 -> [w1390]
          tunnel: [w1388] -> w1373
          tunnel: [w1387] -> w1372
          tunnel: w1373 -> [w1394]
          tunnel: w1372 -> [w1395]
          tunnel: [w1395] -> w1367
          tunnel: [w1394] -> w1366
          tunnel: [w1411] -> w1371
          tunnel: [w1410] -> w1370
          tunnel: w1367 -> [w1409]
          tunnel: w1366 -> [w1408]
          tunnel: w1371 -> [w1416]
          tunnel: w1370 -> [w1415]
          tunnel: [w1413] -> w1368
          tunnel: [w1421] -> w1369
          tunnel: w1368 -> [w1421]
          frame #0 {
            w1381 = TRUE
            n577 = local write "eV4"(w1381) -> ()
            n578 = Bundle(cluster=T4 {"Message"="", "Message Data"=variant} ("Message Cluster"), "Message"="V4" ("Message 3"), "Message Data"=w1381) -> (w1380:T4)
            n579 = Enqueue Element(queue=w1385, element=w1380, error in (no error)=w1384) -> (queue out=w1383:refnum<queue>, error out=w1382:errorcluster)  [unwired: 1 in, 1 out]
          }
          frame #1 {
            n580 = local read "MFC_1 User Set Value"() -> (w1386:dbl)
            n581 = local write "MFC_1\nSLPM Value"(w1386) -> ()
            n582 = Bundle(cluster=T4 {"Message"="", "Message Data"=variant} ("Message Cluster"), "Message"="MFC_1", "Message Data"=w1386) -> (w1389:T4)
            n583 = Enqueue Element(queue=w1391, element=w1389, error in (no error)=w1390) -> (queue out=w1388:refnum<queue>, error out=w1387:errorcluster)  [unwired: 1 in, 1 out]
          }
          frame #2 {
            n584 = for {
              N: 15 -> [w1403]
              i -> [w1402]
              stop <- w1398 stop-if-true
              n585 = Subtract(x=w1403, y=w1402) -> (x-y=w1401:i32)
              n586 = Decrement(x=w1401) -> (x-1=w1399:i32)
              n587 = Wait (ms)(milliseconds to wait=u32 1000) -> ()  [unwired: 1 out]
              n588 = local read "Network disconnected"() -> (w1398:bool)
              n589 = Select(t=0, s=w1398, f=w1399) -> (s? t:f=→"Flush Target Tank\nTime Remain (sec)":i32)
            }
          }
          frame #3 {
            w1412 = FALSE
            n590 = Bundle(cluster=T4 {"Message"="", "Message Data"=variant} ("Message Cluster"), "Message"="V4" ("Message 3"), "Message Data"=w1412) -> (w1407:T4)
            n591 = local write "eV4"(w1412) -> ()
            n592 = Enqueue Element(queue=w1408, element=w1407, error in (no error)=w1409) -> (queue out=w1411:refnum<queue>, error out=w1410:errorcluster)  [unwired: 1 in, 1 out]
          }
          frame #4 {
            w1414 = 0.0 ("MFC_1\nSLPM Value")
            n593 = local write "MFC_1\nSLPM Value"(w1414) -> ()
            n594 = Bundle(cluster=T4 {"Message"="", "Message Data"=variant} ("Message Cluster"), "Message"="MFC_1", "Message Data"=w1414) -> (w1418:T4)
            n595 = Enqueue Element(queue=w1416, element=w1418, error in (no error)=w1415) -> (error out=w1413:errorcluster)  [unwired: 1 in, 2 out]
          }
          frame #5 {
            n596 = local write "Flush Target Tank"(FALSE ("High Cal")) -> ()
          }
        }
      }
      event "Low Cal": Value Change {
        n597 = event-data() -> ()  [unwired: 1 in, 1 out]
        n598 = flat-sequence {
          tunnel: w1433 -> [w1438]
          tunnel: w1432 -> [w1437]
          tunnel: [w1436] -> w1431
          tunnel: [w1435] -> w1430
          tunnel: w1431 -> [w1454]
          tunnel: w1430 -> [w1453]
          tunnel: [w1451] -> w1429
          tunnel: [w1450] -> w1428
          tunnel: [w1459] -> w1427
          tunnel: [w1458] -> w1426
          tunnel: w1428 -> [w1462]
          tunnel: w1429 -> [w1463]
          tunnel: w1427 -> [w1516]
          tunnel: w1426 -> [w1515]
          tunnel: [w1513] -> w1425
          tunnel: [w1512] -> w1424
          tunnel: w1425 -> [w1530]
          tunnel: w1424 -> [w1529]
          tunnel: [w1527] -> w1422
          tunnel: [w1535] -> w1423
          tunnel: w1422 -> [w1535]
          frame #0 {
            w1434 = TRUE
            n599 = Cluster To Array(cluster=cluster{"Message":string, "Message 3":string} {"Message"="V2", "Message 3"="V4"}) -> (array=w1439:string[])
            n600 = for {
              tunnel: w1439 -> [w1446] mode=indexing
              tunnel: w1438 -> [w1445]
              tunnel: w1437 -> [w1444]
              tunnel: [w1443] -> w1436
              tunnel: [w1442] -> w1435
              tunnel: w1434 -> [w1441]
              n601 = Bundle(cluster=T4 {"Message"="", "Message Data"=variant} ("Message Cluster"), "Message"=w1446, "Message Data"=w1441) -> (w1448:T4)
              n602 = Enqueue Element(queue=w1445, element=w1448, error in (no error)=w1444) -> (queue out=w1443:refnum<queue>, error out=w1442:errorcluster)  [unwired: 1 in, 1 out]
            }
            n603 = local write "eV2"(w1434) -> ()
            n604 = local write "eV4"(w1434) -> ()
          }
          frame #1 {
            n605 = local read "MFC_1 User Set Value"() -> (w1449:dbl)
            n606 = local write "MFC_1\nSLPM Value"(w1449) -> ()
            n607 = Bundle(cluster=T4 {"Message"="", "Message Data"=variant} ("Message Cluster"), "Message"="MFC_1", "Message Data"=w1449) -> (w1452:T4)
            n608 = Enqueue Element(queue=w1454, element=w1452, error in (no error)=w1453) -> (queue out=w1451:refnum<queue>, error out=w1450:errorcluster)  [unwired: 1 in, 1 out]
          }
          frame #2 {
            n609 = for {
              N: 45 -> [w1506]
              tunnel: w1463 -> [w1497]
              tunnel: w1462 -> [w1496]
              tunnel: [w1497] -> w1461
              tunnel: [w1496] -> w1460
              tunnel: [w1495] -> w1457
              i -> [w1505]
              stop <- w1495 stop-if-true
              n610 = local read "FGGA Calibration Abort"() -> (w1500:bool)
              n611 = case shown="True" w1500 {
                selector: w1500 -> [w1509 _]
                tunnel: [w1509 w1510] -> w1498
                frame False {
                }
                frame True {
                  n612 = Two Button Dialog(message="Are you sure to abort FGGA Low Cal?") -> (T button?=w1510:bool)  [unwired: 2 in]
                }
              }
              n613 = local read "Network disconnected"() -> (w1499:bool)
              n614 = Subtract(x=w1506, y=w1505) -> (x-y=w1504:i32)
              n615 = Decrement(x=w1504) -> (x-1=w1502:i32)
              n616 = Wait (ms)(milliseconds to wait=u32 1000) -> ()  [unwired: 1 out]
              n617 = Or(x=w1499, y=w1498) -> (x .or. y?=w1495:bool)
              n618 = case shown="False" w1498 {
                selector: w1498 -> [w1508 _]
                frame False {
                  n619 = local write "FGGA Calibration Abort"(w1508) -> ()
                }
                frame True {
                }
              }
              n620 = Select(t=0, s=w1495, f=w1502) -> (s? t:f=→"Low Cal\nFlush Time Remain (sec)":i32)
            }
            n621 = case shown="False" w1457 {
              tunnel: w1461 -> [w1470 w1494]
              tunnel: w1460 -> [w1469 w1493]
              tunnel: [w1467 w1494] -> w1459
              tunnel: [w1465 w1493] -> w1458
              frame False {
                w1471 = TRUE
                # "Carry on if connection to cRIO is made\nor calibration not abort"
                n622 = Bundle(cluster=T4 {"Message"="", "Message Data"=variant} ("Message Cluster"), "Message"="V1", "Message Data"=w1471) -> (w1472:T4)
                n623 = local write "eV1"(w1471) -> ()
                n624 = Enqueue Element(queue=w1470, element=w1472, error in (no error)=w1469) -> (queue out=w1468:refnum<queue>, error out=w1466:errorcluster)  [unwired: 1 in, 1 out]
                n625 = for {
                  N: 60 -> [w1487]
                  tunnel: w1468 -> [w1477]
                  tunnel: [w1477] -> w1467
                  tunnel: w1466 -> [w1476]
                  tunnel: [w1476] -> w1465
                  i -> [w1486]
                  stop <- w1478 stop-if-true
                  n626 = Subtract(x=w1487, y=w1486) -> (x-y=w1485:i32)
                  n627 = local read "FGGA Calibration Abort"() -> (w1480:bool)
                  n628 = case shown="True" w1480 {
                    selector: w1480 -> [w1490 _]
                    tunnel: [w1490 w1491] -> w1479
                    frame False {
                    }
                    frame True {
                      n629 = Two Button Dialog(message="Are you sure to abort FGGA Low Cal?") -> (T button?=w1491:bool)  [unwired: 2 in]
                    }
                  }
                  n630 = Decrement(x=w1485) -> (x-1=w1482:i32)
                  n631 = local read "Network disconnected"() -> (w1481:bool)
                  n632 = Wait (ms)(milliseconds to wait=u32 1000) -> ()  [unwired: 1 out]
                  n633 = Or(x=w1481, y=w1479) -> (x .or. y?=w1478:bool)
                  n634 = case shown="False" w1479 {
                    selector: w1479 -> [w1489 _]
                    frame False {
                      n635 = local write "FGGA Calibration Abort"(w1489) -> ()
                    }
                    frame True {
                    }
                  }
                  n636 = Select(t=0, s=w1478, f=w1482) -> (s? t:f=→"Low Cal\nCal Time Remain (sec)":i32)
                }
              }
              frame True {
              }
            }
          }
          frame #3 {
            w1514 = FALSE
            n637 = Cluster To Array(cluster=T13 {"Message"="V2", "Message 3"="V4", "Message 4"="V1"}) -> (array=w1517:string[])
            n638 = for {
              tunnel: w1517 -> [w1524] mode=indexing
              tunnel: [w1523] -> w1513
              tunnel: [w1522] -> w1512
              tunnel: w1514 -> [w1521]
              tunnel: w1516 -> [w1520]
              tunnel: w1515 -> [w1519]
              n639 = Bundle(cluster=T4 {"Message"="", "Message Data"=variant} ("Message Cluster"), "Message"=w1524, "Message Data"=w1521) -> (w1526:T4)
              n640 = Enqueue Element(queue=w1520, element=w1526, error in (no error)=w1519) -> (queue out=w1523:refnum<queue>, error out=w1522:errorcluster)  [unwired: 1 in, 1 out]
            }
            n641 = local write "eV2"(w1514) -> ()
            n642 = local write "eV4"(w1514) -> ()
            n643 = local write "eV1"(w1514) -> ()
          }
          frame #4 {
            w1528 = 0.0 ("MFC_1\nSLPM Value")
            n644 = local write "MFC_1\nSLPM Value"(w1528) -> ()
            n645 = Bundle(cluster=T4 {"Message"="", "Message Data"=variant} ("Message Cluster"), "Message"="MFC_1", "Message Data"=w1528) -> (w1532:T4)
            n646 = Enqueue Element(queue=w1530, element=w1532, error in (no error)=w1529) -> (error out=w1527:errorcluster)  [unwired: 1 in, 2 out]
          }
          frame #5 {
            w1534 = FALSE ("High Cal")
            n647 = local write "Low Cal"(w1534) -> ()
            n648 = local write "FGGA Calibration Abort"(w1534) -> ()
          }
        }
      }
      event "Target Cal": Value Change {
        n649 = event-data() -> ()  [unwired: 1 in, 1 out]
        n650 = flat-sequence {
          tunnel: w1547 -> [w1555]
          tunnel: w1546 -> [w1554]
          tunnel: [w1553] -> w1545
          tunnel: [w1552] -> w1544
          tunnel: w1545 -> [w1561]
          tunnel: w1544 -> [w1560]
          tunnel: [w1558] -> w1543
          tunnel: [w1557] -> w1542
          tunnel: w1542 -> [w1568]
          tunnel: w1543 -> [w1569]
          tunnel: [w1566] -> w1537
          tunnel: [w1565] -> w1536
          tunnel: [w1621] -> w1541
          tunnel: [w1622] -> w1540
          tunnel: w1537 -> [w1620]
          tunnel: w1536 -> [w1619]
          tunnel: w1541 -> [w1637]
          tunnel: w1540 -> [w1636]
          tunnel: [w1634] -> w1538
          tunnel: [w1642] -> w1539
          tunnel: w1538 -> [w1642]
          frame #0 {
            w1551 = TRUE
            n651 = local write "eV4"(w1551) -> ()
            n652 = Bundle(cluster=T4 {"Message"="", "Message Data"=variant} ("Message Cluster"), "Message"="V4" ("Message 3"), "Message Data"=w1551) -> (w1550:T4)
            n653 = Enqueue Element(queue=w1555, element=w1550, error in (no error)=w1554) -> (queue out=w1553:refnum<queue>, error out=w1552:errorcluster)  [unwired: 1 in, 1 out]
          }
          frame #1 {
            n654 = local read "MFC_1 User Set Value"() -> (w1556:dbl)
            n655 = local write "MFC_1\nSLPM Value"(w1556) -> ()
            n656 = Bundle(cluster=T4 {"Message"="", "Message Data"=variant} ("Message Cluster"), "Message"="MFC_1", "Message Data"=w1556) -> (w1559:T4)
            n657 = Enqueue Element(queue=w1561, element=w1559, error in (no error)=w1560) -> (queue out=w1558:refnum<queue>, error out=w1557:errorcluster)  [unwired: 1 in, 1 out]
          }
          frame #2 {
            n658 = for {
              N: 45 -> [w1613]
              tunnel: [w1604] -> w1570
              tunnel: w1569 -> [w1604]
              tunnel: [w1603] -> w1567
              tunnel: w1568 -> [w1603]
              tunnel: [w1602] -> w1564
              i -> [w1612]
              stop <- w1602 stop-if-true
              n659 = Subtract(x=w1613, y=w1612) -> (x-y=w1611:i32)
              n660 = Decrement(x=w1611) -> (x-1=w1608:i32)
              n661 = local read "FGGA Calibration Abort"() -> (w1607:bool)
              n662 = local read "Network disconnected"() -> (w1606:bool)
              n663 = case shown="True" w1607 {
                selector: w1607 -> [w1616 _]
                tunnel: [w1616 w1617] -> w1605
                frame False {
                }
                frame True {
                  n664 = Two Button Dialog(message="Are you sure to abort FGGA Target Cal?") -> (T button?=w1617:bool)  [unwired: 2 in]
                }
              }
              n665 = Wait (ms)(milliseconds to wait=u32 1000) -> ()  [unwired: 1 out]
              n666 = Or(x=w1606, y=w1605) -> (x .or. y?=w1602:bool)
              n667 = case shown="False" w1605 {
                selector: w1605 -> [w1615 _]
                frame False {
                  n668 = local write "FGGA Calibration Abort"(w1615) -> ()
                }
                frame True {
                }
              }
              n669 = Select(t=0, s=w1602, f=w1608) -> (s? t:f=→"Target Cal\nFlush Time Remain (sec)":i32)
            }
            n670 = case shown="False" w1564 {
              tunnel: w1570 -> [w1577 w1601]
              tunnel: w1567 -> [w1576 w1600]
              tunnel: [w1573 w1601] -> w1566
              tunnel: [w1572 w1600] -> w1565
              frame False {
                w1578 = TRUE
                # "Carry on if connection to cRIO is made\nor calibration not abort"
                n671 = Bundle(cluster=T4 {"Message"="", "Message Data"=variant} ("Message Cluster"), "Message"="V1", "Message Data"=w1578) -> (w1579:T4)
                n672 = local write "eV1"(w1578) -> ()
                n673 = Enqueue Element(queue=w1577, element=w1579, error in (no error)=w1576) -> (queue out=w1575:refnum<queue>, error out=w1574:errorcluster)  [unwired: 1 in, 1 out]
                n674 = for {
                  N: 60 -> [w1594]
                  tunnel: w1575 -> [w1584]
                  tunnel: w1574 -> [w1583]
                  tunnel: [w1584] -> w1573
                  tunnel: [w1583] -> w1572
                  i -> [w1593]
                  stop <- w1585 stop-if-true
                  n675 = Subtract(x=w1594, y=w1593) -> (x-y=w1592:i32)
                  n676 = Decrement(x=w1592) -> (x-1=w1590:i32)
                  n677 = local read "FGGA Calibration Abort"() -> (w1588:bool)
                  n678 = case shown="True" w1588 {
                    selector: w1588 -> [w1597 _]
                    tunnel: [w1597 w1598] -> w1586
                    frame False {
                    }
                    frame True {
                      n679 = Two Button Dialog(message="Are you sure to abort FGGA Target Cal?") -> (T button?=w1598:bool)  [unwired: 2 in]
                    }
                  }
                  n680 = Wait (ms)(milliseconds to wait=u32 1000) -> ()  [unwired: 1 out]
                  n681 = local read "Network disconnected"() -> (w1587:bool)
                  n682 = Or(x=w1587, y=w1586) -> (x .or. y?=w1585:bool)
                  n683 = case shown="False" w1586 {
                    selector: w1586 -> [w1596 _]
                    frame False {
                      n684 = local write "FGGA Calibration Abort"(w1596) -> ()
                    }
                    frame True {
                    }
                  }
                  n685 = Select(t=0, s=w1585, f=w1590) -> (s? t:f=→"Target Cal\nCal Time Remain (sec)":i32)
                }
              }
              frame True {
              }
            }
          }
          frame #3 {
            w1625 = FALSE
            n686 = Cluster To Array(cluster=cluster{"Message 3":string, "Message":string} {"Message 3"="V4", "Message"="V1"}) -> (array=w1623:string[])
            n687 = for {
              tunnel: w1623 -> [w1631] mode=indexing
              tunnel: [w1630] -> w1621
              tunnel: [w1629] -> w1622
              tunnel: w1625 -> [w1628]
              tunnel: w1620 -> [w1627]
              tunnel: w1619 -> [w1626]
              n688 = Bundle(cluster=T4 {"Message"="", "Message Data"=variant} ("Message Cluster"), "Message"=w1631, "Message Data"=w1628) -> (w1633:T4)
              n689 = Enqueue Element(queue=w1627, element=w1633, error in (no error)=w1626) -> (queue out=w1630:refnum<queue>, error out=w1629:errorcluster)  [unwired: 1 in, 1 out]
            }
            n690 = local write "eV4"(w1625) -> ()
            n691 = local write "eV1"(w1625) -> ()
          }
          frame #4 {
            w1635 = 0.0 ("MFC_1\nSLPM Value")
            n692 = local write "MFC_1\nSLPM Value"(w1635) -> ()
            n693 = Bundle(cluster=T4 {"Message"="", "Message Data"=variant} ("Message Cluster"), "Message"="MFC_1", "Message Data"=w1635) -> (w1639:T4)
            n694 = Enqueue Element(queue=w1637, element=w1639, error in (no error)=w1636) -> (error out=w1634:errorcluster)  [unwired: 1 in, 2 out]
          }
          frame #5 {
            w1641 = FALSE ("High Cal")
            n695 = local write "Target Cal"(w1641) -> ()
            n696 = local write "FGGA Calibration Abort"(w1641) -> ()
          }
        }
      }
      event "MFC_1\nSLPM Value": Value Change {
        n697 = event-data() -> ()  [unwired: 1 in, 1 out]
        n698 = local read "MFC_1\nSLPM Value"() -> (w1643:dbl)
        n699 = Bundle(cluster=T4 {"Message"="", "Message Data"=variant} ("Message Cluster"), "Message"="MFC_1", "Message Data"=w1643) -> (w1647:T4)
        n700 = Enqueue Element(queue=w1646, element=w1647, error in (no error)=w1645) -> (error out=w1644:errorcluster)  [unwired: 1 in, 2 out]
      }
      event "FGGA UDP Time Offset": Value Change {
        n701 = event-data() -> ("NewVal"=w1650:i32)  [unwired: 1 in, 5 out]
        n702 = Bundle(cluster=T4 {"Message"="", "Message Data"=variant} ("Message Cluster"), "Message"="UDP Time Offset", "Message Data"=w1650) -> (w1654:T4)
        n703 = Enqueue Element(queue=w1653, element=w1654, error in (no error)=w1652) -> (error out=w1651:errorcluster)  [unwired: 1 in, 2 out]
      }
    }
    "FGGA Event Error out" <- w768
  }
  n704 = node-c288(w14) -> ()  [unwired: 1 out]
  n705 = Create Network Stream Writer Endpoint(6:w54, 7:10 ("writer buffer size"), 9:w56, 10:"//192.168.101.17/command/reader/FGGA" ("reader url"), 11:"/command/writer/FGGA" ("writer name")) -> (0:w53:errorcluster, 3:w52:refnum<k21>)  [unwired: 2 in]
  n706 = while {
    tunnel: w6 -> [w1664]
    shift-right: [w1659] -> _
    shift-left: w52 -> [w1661]
    shift-right: [w1657] -> w49
    shift-left: w53 -> [w1663]
    tunnel: w5 -> [w1658]
    stop <- w1657 stop-if-true
    # "FGGA UI Command Sender"
    n707 = Dequeue Element(queue=w1664, error in (no error)=w1658) -> (element=w1660:T4)  [unwired: 1 in, 3 out]
    n708 = Unbundle By Name(w1660) -> ("Message"=w1662:string)
    n709 = case shown="\"UDP Time Offset\"" w1662 {
      tunnel: w1663 -> [w1665 w1669 w1676 w1683 w1690 w1697 w1704 w1711 w1718 w1725 w1732]
      tunnel: w1661 -> [w1666 w1672 w1679 w1686 w1693 w1700 w1707 w1714 w1721 w1728 w1735]
      tunnel: w1660 -> [_ w1671 w1678 w1685 w1692 w1699 w1706 w1713 w1720 w1727 w1734]
      tunnel: [w1665 w1668 w1675 w1682 w1689 w1696 w1703 w1710 w1717 w1724 w1731] -> w1657
      tunnel: [w1666 w1667 w1674 w1681 w1688 w1695 w1702 w1709 w1716 w1723 w1730] -> w1659
      frame "False", Default {
      }
      frame "V1" {
        n710 = shared-variable-write(w1672, w1669, w1671) -> (w1670:refnum<k21>, w1673:errorcluster)  [unwired: 1 in, 1 out]
        n711 = Flush Stream(8:w1673, 11:w1670) -> (0:w1668:errorcluster, 3:w1667:refnum<k21>)  [unwired: 2 in, 1 out]
      }
      frame "MFC_1" {
        n712 = shared-variable-write(w1679, w1676, w1678) -> (w1677:refnum<k21>, w1680:errorcluster)  [unwired: 1 in, 1 out]
        n713 = Flush Stream(8:w1680, 11:w1677) -> (0:w1675:errorcluster, 3:w1674:refnum<k21>)  [unwired: 2 in, 1 out]
      }
      frame "UDP Time Offset" {
        n714 = shared-variable-write(w1686, w1683, w1685) -> (w1684:refnum<k21>, w1687:errorcluster)  [unwired: 1 in, 1 out]
        n715 = Flush Stream(8:w1687, 11:w1684) -> (0:w1682:errorcluster, 3:w1681:refnum<k21>)  [unwired: 2 in, 1 out]
      }
      frame "V2" {
        n716 = shared-variable-write(w1693, w1690, w1692) -> (w1691:refnum<k21>, w1694:errorcluster)  [unwired: 1 in, 1 out]
        n717 = Flush Stream(8:w1694, 11:w1691) -> (0:w1689:errorcluster, 3:w1688:refnum<k21>)  [unwired: 2 in, 1 out]
      }
      frame "V3" {
        n718 = shared-variable-write(w1700, w1697, w1699) -> (w1698:refnum<k21>, w1701:errorcluster)  [unwired: 1 in, 1 out]
        n719 = Flush Stream(8:w1701, 11:w1698) -> (0:w1696:errorcluster, 3:w1695:refnum<k21>)  [unwired: 2 in, 1 out]
      }
      frame "V4" {
        n720 = shared-variable-write(w1707, w1704, w1706) -> (w1705:refnum<k21>, w1708:errorcluster)  [unwired: 1 in, 1 out]
        n721 = Flush Stream(8:w1708, 11:w1705) -> (0:w1703:errorcluster, 3:w1702:refnum<k21>)  [unwired: 2 in, 1 out]
      }
      frame "FGGA_pump" {
        n722 = shared-variable-write(w1714, w1711, w1713) -> (w1712:refnum<k21>, w1715:errorcluster)  [unwired: 1 in, 1 out]
        n723 = Flush Stream(8:w1715, 11:w1712) -> (0:w1710:errorcluster, 3:w1709:refnum<k21>)  [unwired: 2 in, 1 out]
      }
      frame "Flight Number" {
        n724 = shared-variable-write(w1721, w1718, w1720) -> (w1719:refnum<k21>, w1722:errorcluster)  [unwired: 1 in, 1 out]
        n725 = Flush Stream(8:w1722, 11:w1719) -> (0:w1717:errorcluster, 3:w1716:refnum<k21>)  [unwired: 2 in, 1 out]
      }
      frame "FGGA_restart" {
        n726 = shared-variable-write(w1728, w1725, w1727) -> (w1726:refnum<k21>, w1729:errorcluster)  [unwired: 1 in, 1 out]
        n727 = Flush Stream(8:w1729, 11:w1726) -> (0:w1724:errorcluster, 3:w1723:refnum<k21>)  [unwired: 2 in, 1 out]
      }
      frame "Stop File Write" {
        n728 = shared-variable-write(w1735, w1732, w1734) -> (w1733:refnum<k21>, w1736:errorcluster)  [unwired: 1 in, 1 out]
        n729 = Flush Stream(8:w1736, 11:w1733) -> (0:w1731:errorcluster, 3:w1730:refnum<k21>)  [unwired: 2 in, 1 out]
      }
    }
  }
  "FGGA command sender error out" <- w49
  n730 = local write "FGGA Calibration Abort"(FALSE ("FGGA Calibration Abort")) -> ()
  n731 = Obtain Queue(name (unnamed)="SO2_Command", element data type=w40) -> (queue out=w4:refnum<queue>, error out=w3:errorcluster)  [unwired: 3 in, 1 out]
  n732 = while {
    tunnel: w4 -> [w1740]
    tunnel: w3 -> [w1739]
    tunnel: [w1737] -> _
    stop <- FALSE stop-if-true
    # "SO2 UI Event Handler Loop"
    n733 = event shown="[7] \"SO2 Zero Calibration\": Value Change" {
      selector: _ -> [_ _ _ _ _ _ _ _ _ _ _ _ _ _ _ _ _ _ _ _ _ _ _ _ _ _ _ _ _ _]
      dyn-events: _ -> [_ _ _ _ _ _ _ _ _ _ _ _ _ _ _ _ _ _ _ _ _ _ _ _ _ _ _ _ _ _]
      timeout: _ -> [_ _ _ _ _ _ _ _ _ _ _ _ _ _ _ _ _ _ _ _ _ _ _ _ _ _ _ _ _ _]
      tunnel: w1740 -> [w1747 w1759 w1806 w1817 w1860 w1895 w2006 w2154 w2280 w2286 w2297 w2300 w2308 w2314 w2321 w2327 w2333 w2343 w2347 w2354 w2361 w2368 w2375 w2382 w2389 w2396 w2403 w2410 w2418 w2432]
      tunnel: w1739 -> [w1746 w1758 w1805 w1816 w1859 w1894 w2005 w2153 w2279 w2285 w2296 w2299 w2306 w2313 w2320 w2326 w2332 w2342 w2346 w2353 w2360 w2367 w2374 w2381 w2388 w2395 w2402 w2409 w2417 w2431]
      tunnel: [w1741 w1757 _ w1815 w1858 _ _ _ _ _ w2291 w2298 w2305 _ w2319 _ _ w2337 w2345 w2352 w2359 w2366 w2373 w2380 w2387 w2394 w2401 w2408 w2416 w2430] -> w1737
      event "eV9": Value Change {
        n734 = event-data() -> ("NewVal"=w1744:bool)  [unwired: 1 in]
        n735 = Bundle(cluster=T4 {"Message"="", "Message Data"=variant} ("Message Cluster"), "Message"="V9", "Message Data"=w1744) -> (w1742:T4)
        n736 = Enqueue Element(queue=w1747, element=w1742, error in (no error)=w1746) -> (error out=w1741:errorcluster)  [unwired: 1 in, 2 out]
      }
      event "SO2 Flush": Value Change {
        n737 = event-data() -> ()  [unwired: 1 in, 1 out]
        n738 = flat-sequence {
          tunnel: w1759 -> [w1767]
          tunnel: w1758 -> [w1766]
          tunnel: [w1762] -> w1754
          tunnel: [w1760] -> w1752
          tunnel: w1754 -> [w1769]
          tunnel: [w1771] -> w1753
          tunnel: w1752 -> [w1770]
          tunnel: [w1772] -> w1751
          tunnel: w1753 -> [w1778]
          tunnel: [w1778] -> w1756
          tunnel: [w1776] -> w1755
          tunnel: w1751 -> [w1776]
          tunnel: w1756 -> [w1790]
          tunnel: [w1789] -> w1750
          tunnel: w1755 -> [w1791]
          tunnel: [w1787] -> w1748
          tunnel: w1750 -> [w1797]
          tunnel: [w1798] -> w1749
          tunnel: w1748 -> [w1796]
          tunnel: [w1803] -> w1757
          tunnel: w1749 -> [w1803]
          frame #0 {
            w1761 = TRUE ("SO2 Flush")
            n739 = Bundle(cluster=T4 {"Message"="", "Message Data"=variant} ("Message Cluster"), "Message"="V9", "Message Data"=w1761) -> (w1763:T4)
            n740 = local write "eV9"(w1761) -> ()
            n741 = Enqueue Element(queue=w1767, element=w1763, error in (no error)=w1766) -> (queue out=w1760:refnum<queue>, error out=w1762:errorcluster)  [unwired: 1 in, 1 out]
          }
          frame #1 {
            n742 = local read "MFC_2 User Set Value"() -> (w1768:dbl)
            n743 = local write "MFC_2\nSLPM Value"(w1768) -> ()
            n744 = Bundle(cluster=T4 {"Message"="", "Message Data"=variant} ("Message Cluster"), "Message"="MFC_2", "Message Data"=w1768) -> (w1773:T4)
            n745 = Enqueue Element(queue=w1770, element=w1773, error in (no error)=w1769) -> (queue out=w1772:refnum<queue>, error out=w1771:errorcluster)  [unwired: 1 in, 1 out]
          }
          frame #2 {
            n746 = for {
              N: "eV9 Flush User\nset time (sec)" -> [w1785]
              i -> [w1784]
              stop <- w1779 stop-if-true
              n747 = local read "Network disconnected"() -> (w1779:bool)
              n748 = Subtract(x=w1785, y=w1784) -> (x-y=w1783:i32)
              n749 = Decrement(x=w1783) -> (x-1=w1781:i32)
              n750 = Wait (ms)(milliseconds to wait=u32 1000) -> ()  [unwired: 1 out]
              n751 = Select(t=0, s=w1779, f=w1781) -> (s? t:f=w1780:i32)
              n752 = local write "SO2 Flush\nTime Remain (sec)"(w1780) -> ()
            }
          }
          frame #3 {
            w1788 = FALSE
            n753 = Bundle(cluster=T4 {"Message"="", "Message Data"=variant} ("Message Cluster"), "Message"="V9", "Message Data"=w1788) -> (w1792:T4)
            n754 = local write "eV9"(w1788) -> ()
            n755 = Enqueue Element(queue=w1791, element=w1792, error in (no error)=w1790) -> (queue out=w1787:refnum<queue>, error out=w1789:errorcluster)  [unwired: 1 in, 1 out]
          }
          frame #4 {
            w1795 = 0.0 ("MFC_2\nSLPM Value")
            n756 = local write "MFC_2\nSLPM Value"(w1795) -> ()
            n757 = Bundle(cluster=T4 {"Message"="", "Message Data"=variant} ("Message Cluster"), "Message"="MFC_2", "Message Data"=w1795) -> (w1799:T4)
            n758 = Enqueue Element(queue=w1796, element=w1799, error in (no error)=w1797) -> (error out=w1798:errorcluster)  [unwired: 1 in, 2 out]
          }
          frame #5 {
            n759 = local write "SO2 Flush"(FALSE ("SO2 Flush")) -> ()
          }
        }
      }
      event "Auto Zeroing \ninterval (sec)": Value Change {
        n760 = event-data() -> ("NewVal"=w1804:i32)  [unwired: 1 in]
        n761 = Bundle(cluster=T4 {"Message"="", "Message Data"=variant} ("Message Cluster"), "Message"="zeroing_interval", "Message Data"=w1804) -> (w1807:T4)
        n762 = Enqueue Element(queue=w1806, element=w1807, error in (no error)=w1805) -> ()  [unwired: 1 in, 3 out]
      }
      event "SO2 GND Zeroing": Value Change {
        n763 = event-data() -> ()  [unwired: 1 in, 1 out]
        n764 = flat-sequence {
          tunnel: w1817 -> [w1825]
          tunnel: w1816 -> [w1824]
          tunnel: [w1820] -> w1814
          tunnel: [w1818] -> w1810
          tunnel: w1814 -> [w1828]
          tunnel: [w1828] -> w1813
          tunnel: [w1827] -> w1811
          tunnel: w1810 -> [w1827]
          tunnel: w1813 -> [w1846]
          tunnel: [w1845] -> w1812
          tunnel: w1811 -> [w1847]
          tunnel: [w1852] -> w1815
          tunnel: w1812 -> [w1852]
          frame #0 {
            w1819 = TRUE ("SO2 Flush")
            n765 = local write "SO2 eV6"(w1819) -> ()
            n766 = Bundle(cluster=T4 {"Message"="", "Message Data"=variant} ("Message Cluster"), "Message"="V6", "Message Data"=w1819) -> (w1821:T4)
            n767 = Enqueue Element(queue=w1825, element=w1821, error in (no error)=w1824) -> (queue out=w1818:refnum<queue>, error out=w1820:errorcluster)  [unwired: 1 in, 1 out]
          }
          frame #1 {
            # "10 Mins Count down"
            n768 = for {
              N: "eV6 User\nset time (sec)" -> [w1838]
              i -> [w1837]
              stop <- w1829 stop-if-true
              n769 = local read "SO2 Calibration Abort"() -> (w1835:bool)
              n770 = case shown="True" w1835 {
                selector: w1835 -> [w1841 _]
                tunnel: [w1841 w1842] -> w1830
                frame False {
                }
                frame True {
                  n771 = Two Button Dialog(message="Are you sure to abort SO2 Zeroing?") -> (T button?=w1842:bool)  [unwired: 2 in]
                }
              }
              n772 = Subtract(x=w1838, y=w1837) -> (x-y=w1836:i32)
              n773 = Decrement(x=w1836) -> (x-1=w1832:i32)
              n774 = Wait (ms)(milliseconds to wait=u32 1000) -> ()  [unwired: 1 out]
              n775 = local read "Network disconnected"() -> (w1833:bool)
              n776 = Or(x=w1833, y=w1830) -> (x .or. y?=w1829:bool)
              n777 = case shown="False" w1830 {
                selector: w1830 -> [w1840 _]
                frame False {
                  n778 = local write "SO2 Calibration Abort"(w1840) -> ()
                }
                frame True {
                }
              }
              n779 = Select(t=0, s=w1829, f=w1832) -> (s? t:f=w1831:i32)
              n780 = local write "SO2 Zeroing\nTime Remain (sec)"(w1831) -> ()
            }
          }
          frame #2 {
            w1844 = FALSE
            n781 = Bundle(cluster=T4 {"Message"="", "Message Data"=variant} ("Message Cluster"), "Message"="V6", "Message Data"=w1844) -> (w1848:T4)
            n782 = local write "SO2 eV6"(w1844) -> ()
            n783 = Enqueue Element(queue=w1847, element=w1848, error in (no error)=w1846) -> (error out=w1845:errorcluster)  [unwired: 1 in, 2 out]
          }
          frame #3 {
            n784 = local write "SO2 GND Zeroing"(FALSE ("SO2 Flush")) -> ()
          }
        }
      }
      event "SO2 Inflight \nZeroing": Value Change {
        n785 = event-data() -> ()  [unwired: 1 in, 1 out]
        n786 = flat-sequence {
          tunnel: w1860 -> [w1868]
          tunnel: w1859 -> [w1867]
          tunnel: [w1863] -> w1857
          tunnel: [w1861] -> w1853
          tunnel: w1857 -> [w1871]
          tunnel: [w1871] -> w1856
          tunnel: [w1870] -> w1854
          tunnel: w1853 -> [w1870]
          tunnel: w1856 -> [w1879]
          tunnel: [w1878] -> w1855
          tunnel: w1854 -> [w1880]
          tunnel: [w1885] -> w1858
          tunnel: w1855 -> [w1885]
          frame #0 {
            w1862 = TRUE ("SO2 Flush")
            n787 = local write "SO2 eV6"(w1862) -> ()
            n788 = Bundle(cluster=T4 {"Message"="", "Message Data"=variant} ("Message Cluster"), "Message"="V6", "Message Data"=w1862) -> (w1864:T4)
            n789 = Enqueue Element(queue=w1868, element=w1864, error in (no error)=w1867) -> (queue out=w1861:refnum<queue>, error out=w1863:errorcluster)  [unwired: 1 in, 1 out]
          }
          frame #1 {
            n790 = for {
              N: "eV6 User set time \n(Inflight) (sec)" -> [w1875]
              i -> [w1874]
              n791 = Subtract(x=w1875, y=w1874) -> (x-y=w1873:i32)
              n792 = Decrement(x=w1873) -> (x-1=w1872:i32)
              n793 = local write "SO2 Zeroing (Inflight)\nTime Remain (sec)"(w1872) -> ()
              n794 = Wait (ms)(milliseconds to wait=u32 1000) -> ()  [unwired: 1 out]
            }
          }
          frame #2 {
            w1877 = FALSE
            n795 = Bundle(cluster=T4 {"Message"="", "Message Data"=variant} ("Message Cluster"), "Message"="V6", "Message Data"=w1877) -> (w1881:T4)
            n796 = local write "SO2 eV6"(w1877) -> ()
            n797 = Enqueue Element(queue=w1880, element=w1881, error in (no error)=w1879) -> (error out=w1878:errorcluster)  [unwired: 1 in, 2 out]
          }
          frame #3 {
            n798 = local write "SO2 Inflight \nZeroing"(FALSE ("SO2 Flush")) -> ()
          }
        }
      }
      event "SO2 Zero CAL": Value Change {
        n799 = event-data() -> ()  [unwired: 1 in, 1 out]
        n800 = flat-sequence {
          tunnel: [w1898] -> w1893
          tunnel: [w1897] -> w1891
          tunnel: w1895 -> [w1903]
          tunnel: w1894 -> [w1902]
          tunnel: w1893 -> [w1907]
          tunnel: [w1906] -> w1892
          tunnel: w1891 -> [w1908]
          tunnel: [w1904] -> w1890
          tunnel: [w1914] -> w1889
          tunnel: [w1913] -> w1888
          tunnel: w1890 -> [w1918]
          tunnel: w1892 -> [w1916]
          tunnel: w1889 -> [w1970]
          tunnel: w1888 -> [w1969]
          tunnel: [w1968] -> w1887
          tunnel: [w1967] -> w1886
          tunnel: w1887 -> [w1984]
          tunnel: w1886 -> [w1983]
          frame #0 {
            w1896 = TRUE ("SO2 Flush")
            n801 = Bundle(cluster=T4 {"Message"="", "Message Data"=variant} ("Message Cluster"), "Message"="V9", "Message Data"=w1896) -> (w1899:T4)
            n802 = local write "eV9"(w1896) -> ()
            n803 = Enqueue Element(queue=w1903, element=w1899, error in (no error)=w1902) -> (queue out=w1897:refnum<queue>, error out=w1898:errorcluster)  [unwired: 1 in, 1 out]
          }
          frame #1 {
            n804 = local read "MFC_2 User Set Value"() -> (w1905:dbl)
            n805 = local write "MFC_2\nSLPM Value"(w1905) -> ()
            n806 = Bundle(cluster=T4 {"Message"="", "Message Data"=variant} ("Message Cluster"), "Message"="MFC_2", "Message Data"=w1905) -> (w1909:T4)
            n807 = Enqueue Element(queue=w1908, element=w1909, error in (no error)=w1907) -> (queue out=w1904:refnum<queue>, error out=w1906:errorcluster)  [unwired: 1 in, 1 out]
          }
          frame #2 {
            n808 = for {
              N: "eV9 flush User\nset time (sec)" -> [w1961]
              tunnel: [w1952] -> w1917
              tunnel: w1918 -> [w1952]
              tunnel: [w1951] -> w1915
              tunnel: w1916 -> [w1951]
              tunnel: [w1950] -> w1912
              i -> [w1960]
              stop <- w1950 stop-if-true
              n809 = local read "SO2 Calibration Abort"() -> (w1957:bool)
              n810 = case shown="True" w1957 {
                selector: w1957 -> [w1964 _]
                tunnel: [w1964 w1965] -> w1955
                frame False {
                }
                frame True {
                  n811 = Two Button Dialog(message="Are you sure to abort SO2 Cal?") -> (T button?=w1965:bool)  [unwired: 2 in]
                }
              }
              n812 = Subtract(x=w1961, y=w1960) -> (x-y=w1959:i32)
              n813 = Decrement(x=w1959) -> (x-1=w1953:i32)
              n814 = Wait (ms)(milliseconds to wait=u32 1000) -> ()  [unwired: 1 out]
              n815 = local read "Network disconnected"() -> (w1956:bool)
              n816 = Or(x=w1956, y=w1955) -> (x .or. y?=w1950:bool)
              n817 = Select(t=0, s=w1950, f=w1953) -> (s? t:f=w1954:i32)
              n818 = local write "SO2 Zero CAL Flush\nTime Remain (sec)"(w1954) -> ()
              n819 = case shown="False" w1955 {
                selector: w1955 -> [w1963 _]
                frame False {
                  n820 = local write "SO2 Calibration Abort"(w1963) -> ()
                }
                frame True {
                }
              }
            }
            n821 = case shown="False" w1912 {
              tunnel: w1917 -> [w1925 w1949]
              tunnel: w1915 -> [w1924 w1948]
              tunnel: [w1922 w1949] -> w1914
              tunnel: [w1920 w1948] -> w1913
              frame False {
                w1926 = TRUE ("SO2 Flush")
                # "carry on cal when no connection problem or abort not confirmed"
                n822 = Bundle(cluster=T4 {"Message"="", "Message Data"=variant} ("Message Cluster"), "Message"="V8", "Message Data"=w1926) -> (w1927:T4)
                n823 = local write "eV8"(w1926) -> ()
                n824 = Enqueue Element(queue=w1925, element=w1927, error in (no error)=w1924) -> (queue out=w1923:refnum<queue>, error out=w1921:errorcluster)  [unwired: 1 in, 1 out]
                n825 = for {
                  N: "eV8 User\nset time (sec)" -> [w1942]
                  tunnel: [w1932] -> w1922
                  tunnel: w1923 -> [w1932]
                  tunnel: [w1931] -> w1920
                  tunnel: w1921 -> [w1931]
                  i -> [w1941]
                  stop <- w1933 stop-if-true
                  n826 = local read "SO2 Calibration Abort"() -> (w1939:bool)
                  n827 = case shown="True" w1939 {
                    selector: w1939 -> [w1945 _]
                    tunnel: [w1945 w1946] -> w1936
                    frame False {
                    }
                    frame True {
                      n828 = Two Button Dialog(message="Are you sure to abort SO2 Cal?") -> (T button?=w1946:bool)  [unwired: 2 in]
                    }
                  }
                  n829 = Subtract(x=w1942, y=w1941) -> (x-y=w1940:i32)
                  n830 = local read "Network disconnected"() -> (w1937:bool)
                  n831 = Decrement(x=w1940) -> (x-1=w1935:i32)
                  n832 = Or(x=w1937, y=w1936) -> (x .or. y?=w1933:bool)
                  n833 = Select(t=0, s=w1933, f=w1935) -> (s? t:f=w1934:i32)
                  n834 = case shown="False" w1936 {
                    selector: w1936 -> [w1944 _]
                    frame False {
                      n835 = local write "SO2 Calibration Abort"(w1944) -> ()
                    }
                    frame True {
                    }
                  }
                  n836 = local write "SO2 Zero CAL\nTime Remain (sec)"(w1934) -> ()
                  n837 = Wait (ms)(milliseconds to wait=u32 1000) -> ()  [unwired: 1 out]
                }
              }
              frame True {
                # "Ignore the rest of the cal when there is connection problem or abort confirmed"
              }
            }
          }
          frame #3 {
            n838 = Cluster To Array(cluster=cluster{"Message":string, "Message 2":string} {"Message"="V8", "Message 2"="V9"}) -> (array=w1972:string[])
            n839 = for {
              tunnel: w1972 -> [w1979] mode=indexing
              tunnel: FALSE ("SO2 Flush") -> [w1978]
              tunnel: w1970 -> [w1977]
              tunnel: w1969 -> [w1976]
              tunnel: [w1975] -> w1968
              tunnel: [w1974] -> w1967
              n840 = Bundle(cluster=T4 {"Message"="", "Message Data"=variant} ("Message Cluster"), "Message"=w1979, "Message Data"=w1978) -> (w1980:T4)
              n841 = Enqueue Element(queue=w1977, element=w1980, error in (no error)=w1976) -> (queue out=w1975:refnum<queue>, error out=w1974:errorcluster)  [unwired: 1 in, 1 out]
            }
          }
          frame #4 {
            w1982 = 0.0 ("MFC_2\nSLPM Value")
            n842 = local write "MFC_2\nSLPM Value"(w1982) -> ()
            n843 = Bundle(cluster=T4 {"Message"="", "Message Data"=variant} ("Message Cluster"), "Message"="MFC_2", "Message Data"=w1982) -> (w1985:T4)
            n844 = Enqueue Element(queue=w1984, element=w1985, error in (no error)=w1983) -> ()  [unwired: 1 in, 3 out]
          }
          frame #5 {
            w1988 = FALSE ("SO2 Flush")
            n845 = local write "eV9"(w1988) -> ()
            n846 = local write "eV8"(w1988) -> ()
            n847 = local write "SO2 Zero CAL"(w1988) -> ()
            n848 = local write "SO2 Calibration Abort"(w1988) -> ()
          }
        }
      }
      event "SO2 Span Calibration": Value Change {
        n849 = event-data() -> ()  [unwired: 1 in, 1 out]
        n850 = flat-sequence {
          tunnel: w2005 -> [w2010]
          tunnel: w2006 -> [w2011]
          tunnel: [w2008] -> w1994
          tunnel: [w2009] -> w1993
          tunnel: [w2018] -> w1992
          tunnel: [w2016] -> w1990
          tunnel: w1994 -> [w2019]
          tunnel: w1993 -> [w2020]
          tunnel: w1992 -> [w2027]
          tunnel: [w2026] -> w1991
          tunnel: w1990 -> [w2025]
          tunnel: [w2024] -> w1989
          tunnel: [w2041] -> w2004
          tunnel: [w2040] -> w2002
          tunnel: w1991 -> [w2045]
          tunnel: w1989 -> [w2038]
          tunnel: w2004 -> [w2049]
          tunnel: [w2048] -> w2003
          tunnel: w2002 -> [w2050]
          tunnel: [w2046] -> w2001
          tunnel: [w2057] -> w2000
          tunnel: [w2056] -> w1999
          tunnel: w2001 -> [w2061]
          tunnel: w2003 -> [w2059]
          tunnel: w2000 -> [w2112]
          tunnel: w1999 -> [w2111]
          tunnel: [w2110] -> w1998
          tunnel: [w2109] -> w1997
          tunnel: w1998 -> [w2128]
          tunnel: w1997 -> [w2127]
          tunnel: [w2125] -> w1996
          tunnel: [w2124] -> w1995
          tunnel: w1996 -> [w2133]
          tunnel: w1995 -> [w2132]
          frame #0 {
            n851 = local write "SO2 Auto Zeroing"(FALSE ("SO2 Auto Zeroing")) -> ()
            n852 = Bundle(cluster=T4 {"Message"="", "Message Data"=variant} ("Message Cluster"), "Message"="Auto_zero", "Message Data"=FALSE) -> (w2013:T4)
            n853 = Enqueue Element(queue=w2011, element=w2013, error in (no error)=w2010) -> (queue out=w2008:refnum<queue>, error out=w2009:errorcluster)  [unwired: 1 in, 1 out]
          }
          frame #1 {
            n854 = Bundle(cluster=T4 {"Message"="", "Message Data"=variant} ("Message Cluster"), "Message"="mean_cal_status", "Message Data"=FALSE) -> (w2021:T4)
            n855 = Enqueue Element(queue=w2019, element=w2021, error in (no error)=w2020) -> (queue out=w2016:refnum<queue>, error out=w2018:errorcluster)  [unwired: 1 in, 1 out]
          }
          frame #2 {
            n856 = node-c288() -> (w2029:T6)  [unwired: 4 in]
            n857 = timed-loop {
              timing: w2029 -> [_]
              timing-out: [_] -> w2028
              tunnel: [w2031] -> w2026
              tunnel: w2027 -> [w2031]
              tunnel: w2025 -> [w2030]
              tunnel: [w2030] -> w2024
              stop <- w2032 stop-if-true
              n858 = node-c288() -> ()  [unwired: 1 in, 1 out]
              n859 = node-c288() -> ()  [unwired: 1 in, 1 out]
              n860 = One Button Dialog(message="Is Span Gas connected to CALDECK?") -> (true=w2032:bool)  [unwired: 1 in]
            }
            n861 = node-c288(w2028) -> ()  [unwired: 1 out]
          }
          frame #3 {
            w2039 = TRUE ("SO2 Flush")
            n862 = Bundle(cluster=T4 {"Message"="", "Message Data"=variant} ("Message Cluster"), "Message"="V9", "Message Data"=w2039) -> (w2042:T4)
            n863 = local write "eV9"(w2039) -> ()
            n864 = Enqueue Element(queue=w2038, element=w2042, error in (no error)=w2045) -> (queue out=w2040:refnum<queue>, error out=w2041:errorcluster)  [unwired: 1 in, 1 out]
          }
          frame #4 {
            n865 = local read "MFC_2 User Set Value"() -> (w2047:dbl)
            n866 = local write "MFC_2\nSLPM Value"(w2047) -> ()
            n867 = Bundle(cluster=T4 {"Message"="", "Message Data"=variant} ("Message Cluster"), "Message"="MFC_2", "Message Data"=w2047) -> (w2051:T4)
            n868 = Enqueue Element(queue=w2050, element=w2051, error in (no error)=w2049) -> (queue out=w2046:refnum<queue>, error out=w2048:errorcluster)  [unwired: 1 in, 1 out]
          }
          frame #5 {
            n869 = for {
              N: "eV9 span\nflush (sec)" -> [w2103]
              tunnel: [w2094] -> w2060
              tunnel: w2061 -> [w2094]
              tunnel: [w2093] -> w2058
              tunnel: w2059 -> [w2093]
              tunnel: [w2092] -> w2055
              i -> [w2102]
              stop <- w2092 stop-if-true
              n870 = local read "SO2 Calibration Abort"() -> (w2099:bool)
              n871 = case shown="True" w2099 {
                selector: w2099 -> [w2106 _]
                tunnel: [w2106 w2107] -> w2097
                frame False {
                }
                frame True {
                  n872 = Two Button Dialog(message="Are you sure to abort SO2 Cal?") -> (T button?=w2107:bool)  [unwired: 2 in]
                }
              }
              n873 = Subtract(x=w2103, y=w2102) -> (x-y=w2101:i32)
              n874 = Decrement(x=w2101) -> (x-1=w2095:i32)
              n875 = Wait (ms)(milliseconds to wait=u32 1000) -> ()  [unwired: 1 out]
              n876 = local read "Network disconnected"() -> (w2098:bool)
              n877 = Or(x=w2098, y=w2097) -> (x .or. y?=w2092:bool)
              n878 = Select(t=0, s=w2092, f=w2095) -> (s? t:f=w2096:i32)
              n879 = local write "SO2 Zero CAL Flush\nTime Remain (sec)"(w2096) -> ()
              n880 = case shown="False" w2097 {
                selector: w2097 -> [w2105 _]
                frame False {
                  n881 = local write "SO2 Calibration Abort"(w2105) -> ()
                }
                frame True {
                }
              }
            }
            n882 = case shown="False" w2055 {
              tunnel: w2060 -> [w2068 w2091]
              tunnel: w2058 -> [w2067 w2090]
              tunnel: [w2065 w2091] -> w2057
              tunnel: [w2063 w2090] -> w2056
              frame False {
                w2069 = TRUE ("SO2 Flush")
                # "carry on cal when no connection problem or abort not confirmed"
                n883 = Bundle(cluster=T4 {"Message"="", "Message Data"=variant} ("Message Cluster"), "Message"="V8", "Message Data"=w2069) -> (w2070:T4)
                n884 = local write "eV8"(w2069) -> ()
                n885 = Enqueue Element(queue=w2068, element=w2070, error in (no error)=w2067) -> (queue out=w2066:refnum<queue>, error out=w2064:errorcluster)  [unwired: 1 in, 1 out]
                n886 = for {
                  N: "eV8 span\n(sec)" -> [w2084]
                  tunnel: [w2074] -> w2065
                  tunnel: w2066 -> [w2074]
                  tunnel: [w2073] -> w2063
                  tunnel: w2064 -> [w2073]
                  i -> [w2083]
                  stop <- w2075 stop-if-true
                  n887 = local read "SO2 Calibration Abort"() -> (w2081:bool)
                  n888 = case shown="True" w2081 {
                    selector: w2081 -> [w2087 _]
                    tunnel: [w2087 w2088] -> w2078
                    frame False {
                    }
                    frame True {
                      n889 = Two Button Dialog(message="Are you sure to abort SO2 Cal?") -> (T button?=w2088:bool)  [unwired: 2 in]
                    }
                  }
                  n890 = Subtract(x=w2084, y=w2083) -> (x-y=w2082:i32)
                  n891 = local read "Network disconnected"() -> (w2079:bool)
                  n892 = Decrement(x=w2082) -> (x-1=w2077:i32)
                  n893 = Or(x=w2079, y=w2078) -> (x .or. y?=w2075:bool)
                  n894 = Select(t=0, s=w2075, f=w2077) -> (s? t:f=w2076:i32)
                  n895 = case shown="False" w2078 {
                    selector: w2078 -> [w2086 _]
                    frame False {
                      n896 = local write "SO2 Calibration Abort"(w2086) -> ()
                    }
                    frame True {
                    }
                  }
                  n897 = local write "SO2 Zero CAL\nTime Remain (sec)"(w2076) -> ()
                  n898 = Wait (ms)(milliseconds to wait=u32 1000) -> ()  [unwired: 1 out]
                }
              }
              frame True {
                # "Ignore the rest of the cal when there is connection problem or abort confirmed"
              }
            }
          }
          frame #6 {
            n899 = Cluster To Array(cluster=cluster{"Message":string, "Message 2":string} {"Message"="V8", "Message 2"="V9"}) -> (array=w2114:string[])
            n900 = for {
              tunnel: w2114 -> [w2121] mode=indexing
              tunnel: FALSE ("SO2 Flush") -> [w2120]
              tunnel: w2112 -> [w2119]
              tunnel: w2111 -> [w2118]
              tunnel: [w2117] -> w2110
              tunnel: [w2116] -> w2109
              n901 = Bundle(cluster=T4 {"Message"="", "Message Data"=variant} ("Message Cluster"), "Message"=w2121, "Message Data"=w2120) -> (w2122:T4)
              n902 = Enqueue Element(queue=w2119, element=w2122, error in (no error)=w2118) -> (queue out=w2117:refnum<queue>, error out=w2116:errorcluster)  [unwired: 1 in, 1 out]
            }
          }
          frame #7 {
            w2126 = 0.0 ("MFC_2\nSLPM Value")
            n903 = local write "MFC_2\nSLPM Value"(w2126) -> ()
            n904 = Bundle(cluster=T4 {"Message"="", "Message Data"=variant} ("Message Cluster"), "Message"="MFC_2", "Message Data"=w2126) -> (w2129:T4)
            n905 = Enqueue Element(queue=w2128, element=w2129, error in (no error)=w2127) -> (queue out=w2125:refnum<queue>, error out=w2124:errorcluster)  [unwired: 1 in, 1 out]
          }
          frame #8 {
            n906 = Bundle(cluster=T4 {"Message"="", "Message Data"=variant} ("Message Cluster"), "Message"="mean_cal_status", "Message Data"=TRUE) -> (w2135:T4)
            n907 = Enqueue Element(queue=w2133, element=w2135, error in (no error)=w2132) -> ()  [unwired: 1 in, 3 out]
          }
          frame #9 {
            w2138 = FALSE ("SO2 Flush")
            n908 = local write "eV8"(w2138) -> ()
            n909 = local write "eV9"(w2138) -> ()
            n910 = local write "SO2 Span Calibration"(w2138) -> ()
            n911 = local write "SO2 Calibration Abort"(w2138) -> ()
          }
        }
      }
      event "SO2 Zero Calibration": Value Change {
        n912 = event-data() -> ()  [unwired: 1 in, 1 out]
        n913 = flat-sequence {
          tunnel: w2153 -> [w2159]
          tunnel: w2154 -> [w2160]
          tunnel: [w2157] -> w2144
          tunnel: [w2158] -> w2143
          tunnel: [w2166] -> w2142
          tunnel: [w2164] -> w2140
          tunnel: w2144 -> [w2167]
          tunnel: w2143 -> [w2168]
          tunnel: w2142 -> [w2174]
          tunnel: [w2173] -> w2141
          tunnel: w2140 -> [w2175]
          tunnel: [w2172] -> w2139
          tunnel: [w2189] -> w2152
          tunnel: [w2188] -> w2150
          tunnel: w2141 -> [w2193]
          tunnel: w2139 -> [w2186]
          tunnel: w2152 -> [w2197]
          tunnel: [w2196] -> w2151
          tunnel: w2150 -> [w2198]
          tunnel: [w2194] -> w2149
          tunnel: [w2205] -> w2148
          tunnel: [w2204] -> w2147
          tunnel: w2149 -> [w2209]
          tunnel: w2151 -> [w2207]
          tunnel: w2148 -> [w2260]
          tunnel: w2147 -> [w2259]
          tunnel: [w2258] -> w2146
          tunnel: [w2257] -> w2145
          tunnel: w2146 -> [w2274]
          tunnel: w2145 -> [w2273]
          frame #0 {
            n914 = local write "SO2 Auto Zeroing"(FALSE) -> ()
            n915 = Bundle(cluster=T4 {"Message"="", "Message Data"=variant} ("Message Cluster"), "Message"="Auto_zero", "Message Data"=FALSE) -> (w2163:T4)
            n916 = Enqueue Element(queue=w2160, element=w2163, error in (no error)=w2159) -> (queue out=w2157:refnum<queue>, error out=w2158:errorcluster)  [unwired: 1 in, 1 out]
          }
          frame #1 {
            n917 = Bundle(cluster=T4 {"Message"="", "Message Data"=variant} ("Message Cluster"), "Message"="mean_cal_status", "Message Data"=TRUE) -> (w2169:T4)
            n918 = Enqueue Element(queue=w2167, element=w2169, error in (no error)=w2168) -> (queue out=w2164:refnum<queue>, error out=w2166:errorcluster)  [unwired: 1 in, 1 out]
          }
          frame #2 {
            n919 = node-c288() -> (w2177:T6)  [unwired: 4 in]
            n920 = timed-loop {
              timing: w2177 -> [_]
              timing-out: [_] -> w2176
              tunnel: [w2179] -> w2173
              tunnel: w2174 -> [w2179]
              tunnel: w2175 -> [w2178]
              tunnel: [w2178] -> w2172
              stop <- w2180 stop-if-true
              n921 = node-c288() -> ()  [unwired: 1 in, 1 out]
              n922 = node-c288() -> ()  [unwired: 1 in, 1 out]
              n923 = One Button Dialog(message="Is Zero Gas connected to CALDECK?") -> (true=w2180:bool)  [unwired: 1 in]
            }
            n924 = node-c288(w2176) -> ()  [unwired: 1 out]
          }
          frame #3 {
            w2187 = TRUE ("SO2 Flush")
            n925 = Bundle(cluster=T4 {"Message"="", "Message Data"=variant} ("Message Cluster"), "Message"="V9", "Message Data"=w2187) -> (w2190:T4)
            n926 = local write "eV9"(w2187) -> ()
            n927 = Enqueue Element(queue=w2186, element=w2190, error in (no error)=w2193) -> (queue out=w2188:refnum<queue>, error out=w2189:errorcluster)  [unwired: 1 in, 1 out]
          }
          frame #4 {
            n928 = local read "MFC_2 User Set Value"() -> (w2195:dbl)
            n929 = local write "MFC_2\nSLPM Value"(w2195) -> ()
            n930 = Bundle(cluster=T4 {"Message"="", "Message Data"=variant} ("Message Cluster"), "Message"="MFC_2", "Message Data"=w2195) -> (w2199:T4)
            n931 = Enqueue Element(queue=w2198, element=w2199, error in (no error)=w2197) -> (queue out=w2194:refnum<queue>, error out=w2196:errorcluster)  [unwired: 1 in, 1 out]
          }
          frame #5 {
            n932 = for {
              N: "eV9 zero\nflush (sec)" -> [w2251]
              tunnel: [w2242] -> w2208
              tunnel: w2209 -> [w2242]
              tunnel: [w2241] -> w2206
              tunnel: w2207 -> [w2241]
              tunnel: [w2240] -> w2203
              i -> [w2250]
              stop <- w2240 stop-if-true
              n933 = local read "SO2 Calibration Abort"() -> (w2247:bool)
              n934 = case shown="True" w2247 {
                selector: w2247 -> [w2254 _]
                tunnel: [w2254 w2255] -> w2245
                frame False {
                }
                frame True {
                  n935 = Two Button Dialog(message="Are you sure to abort SO2 Cal?") -> (T button?=w2255:bool)  [unwired: 2 in]
                }
              }
              n936 = Subtract(x=w2251, y=w2250) -> (x-y=w2249:i32)
              n937 = Decrement(x=w2249) -> (x-1=w2243:i32)
              n938 = Wait (ms)(milliseconds to wait=u32 1000) -> ()  [unwired: 1 out]
              n939 = local read "Network disconnected"() -> (w2246:bool)
              n940 = Or(x=w2246, y=w2245) -> (x .or. y?=w2240:bool)
              n941 = Select(t=0, s=w2240, f=w2243) -> (s? t:f=w2244:i32)
              n942 = local write "SO2 Zero CAL Flush\nTime Remain (sec)"(w2244) -> ()
              n943 = case shown="False" w2245 {
                selector: w2245 -> [w2253 _]
                frame False {
                  n944 = local write "SO2 Calibration Abort"(w2253) -> ()
                }
                frame True {
                }
              }
            }
            n945 = case shown="False" w2203 {
              tunnel: w2208 -> [w2216 w2239]
              tunnel: w2206 -> [w2215 w2238]
              tunnel: [w2213 w2239] -> w2205
              tunnel: [w2211 w2238] -> w2204
              frame False {
                w2217 = TRUE ("SO2 Flush")
                # "carry on cal when no connection problem or abort not confirmed"
                n946 = Bundle(cluster=T4 {"Message"="", "Message Data"=variant} ("Message Cluster"), "Message"="V8", "Message Data"=w2217) -> (w2218:T4)
                n947 = local write "eV8"(w2217) -> ()
                n948 = Enqueue Element(queue=w2216, element=w2218, error in (no error)=w2215) -> (queue out=w2214:refnum<queue>, error out=w2212:errorcluster)  [unwired: 1 in, 1 out]
                n949 = for {
                  N: "eV8 zero\n(sec)" -> [w2232]
                  tunnel: [w2222] -> w2213
                  tunnel: w2214 -> [w2222]
                  tunnel: [w2221] -> w2211
                  tunnel: w2212 -> [w2221]
                  i -> [w2231]
                  stop <- w2223 stop-if-true
                  n950 = local read "SO2 Calibration Abort"() -> (w2229:bool)
                  n951 = case shown="True" w2229 {
                    selector: w2229 -> [w2235 _]
                    tunnel: [w2235 w2236] -> w2226
                    frame False {
                    }
                    frame True {
                      n952 = Two Button Dialog(message="Are you sure to abort SO2 Cal?") -> (T button?=w2236:bool)  [unwired: 2 in]
                    }
                  }
                  n953 = Subtract(x=w2232, y=w2231) -> (x-y=w2230:i32)
                  n954 = local read "Network disconnected"() -> (w2227:bool)
                  n955 = Decrement(x=w2230) -> (x-1=w2225:i32)
                  n956 = Or(x=w2227, y=w2226) -> (x .or. y?=w2223:bool)
                  n957 = Select(t=0, s=w2223, f=w2225) -> (s? t:f=w2224:i32)
                  n958 = case shown="False" w2226 {
                    selector: w2226 -> [w2234 _]
                    frame False {
                      n959 = local write "SO2 Calibration Abort"(w2234) -> ()
                    }
                    frame True {
                    }
                  }
                  n960 = local write "SO2 Zero CAL\nTime Remain (sec)"(w2224) -> ()
                  n961 = Wait (ms)(milliseconds to wait=u32 1000) -> ()  [unwired: 1 out]
                }
              }
              frame True {
                # "Ignore the rest of the cal when there is connection problem or abort confirmed"
              }
            }
          }
          frame #6 {
            n962 = Cluster To Array(cluster=cluster{"Message":string, "Message 2":string} {"Message"="V8", "Message 2"="V9"}) -> (array=w2262:string[])
            n963 = for {
              tunnel: w2262 -> [w2269] mode=indexing
              tunnel: FALSE ("SO2 Flush") -> [w2268]
              tunnel: w2260 -> [w2267]
              tunnel: w2259 -> [w2266]
              tunnel: [w2265] -> w2258
              tunnel: [w2264] -> w2257
              n964 = Bundle(cluster=T4 {"Message"="", "Message Data"=variant} ("Message Cluster"), "Message"=w2269, "Message Data"=w2268) -> (w2270:T4)
              n965 = Enqueue Element(queue=w2267, element=w2270, error in (no error)=w2266) -> (queue out=w2265:refnum<queue>, error out=w2264:errorcluster)  [unwired: 1 in, 1 out]
            }
          }
          frame #7 {
            w2272 = 0.0 ("MFC_2\nSLPM Value")
            n966 = local write "MFC_2\nSLPM Value"(w2272) -> ()
            n967 = Bundle(cluster=T4 {"Message"="", "Message Data"=variant} ("Message Cluster"), "Message"="MFC_2", "Message Data"=w2272) -> (w2275:T4)
            n968 = Enqueue Element(queue=w2274, element=w2275, error in (no error)=w2273) -> ()  [unwired: 1 in, 3 out]
          }
          frame #8 {
            w2278 = FALSE ("SO2 Flush")
            n969 = local write "eV8"(w2278) -> ()
            n970 = local write "eV9"(w2278) -> ()
            n971 = local write "SO2 Zero Calibration"(w2278) -> ()
            n972 = local write "SO2 Calibration Abort"(w2278) -> ()
          }
        }
      }
      event "eV8 User\nset time (sec)": Value Change {
        n973 = event-data() -> ("NewVal"=w2281:i32)  [unwired: 1 in]
        n974 = Bundle(cluster=T4 {"Message"="", "Message Data"=variant} ("Message Cluster"), "Message"="eV8_user_set_time", "Message Data"=w2281) -> (w2282:T4)
        n975 = Enqueue Element(queue=w2280, element=w2282, error in (no error)=w2279) -> ()  [unwired: 1 in, 3 out]
      }
      event "Offset Mean Zero Calculation (default = ON)\nOFF = User input\nOn = Mean zero calculated with ev8": Value Change {
        n976 = event-data() -> ("NewVal"=w2287:bool)  [unwired: 1 in]
        n977 = Bundle(cluster=T4 {"Message"="", "Message Data"=variant} ("Message Cluster"), "Message"="mean_cal_status", "Message Data"=w2287) -> (w2288:T4)
        n978 = Enqueue Element(queue=w2286, element=w2288, error in (no error)=w2285) -> ()  [unwired: 1 in, 3 out]
      }
      event "MFC_2\nSLPM Value": Value Change {
        n979 = event-data() -> ("NewVal"=w2294:dbl)  [unwired: 1 in]
        n980 = Bundle(cluster=T4 {"Message"="", "Message Data"=variant} ("Message Cluster"), "Message"="MFC_2", "Message Data"=w2294) -> (w2292:T4)
        n981 = Enqueue Element(queue=w2297, element=w2292, error in (no error)=w2296) -> (error out=w2291:errorcluster)  [unwired: 1 in, 2 out]
      }
      event "SO2 Inflight MOCCA Alarm\n(default = OFF)": Value Change {
        n982 = event-data() -> ("NewVal"=w2301:bool)  [unwired: 1 in]
        n983 = Bundle(cluster=T4 {"Message"="", "Message Data"=variant} ("Message Cluster"), "Message"="SO2_MOCCA_Alarm", "Message Data"=w2301) -> (w2302:T4)
        n984 = Enqueue Element(queue=w2300, element=w2302, error in (no error)=w2299) -> (error out=w2298:errorcluster)  [unwired: 1 in, 2 out]
      }
      event "MOCCA window \ndelay time (sec)": Value Change {
        n985 = event-data() -> ("NewVal"=w2307:i32)  [unwired: 1 in]
        n986 = Bundle(cluster=T4 {"Message"="", "Message Data"=variant} ("Message Cluster"), "Message"="MOCCA_window_delay_time", "Message Data"=w2307) -> (w2309:T4)
        n987 = Enqueue Element(queue=w2308, element=w2309, error in (no error)=w2306) -> (error out=w2305:errorcluster)  [unwired: 1 in, 2 out]
      }
      event "MOCCA Limit": Value Change {
        n988 = event-data() -> ("NewVal"=w2312:i32)  [unwired: 1 in]
        n989 = Bundle(cluster=T4 {"Message"="", "Message Data"=variant} ("Message Cluster"), "Message"="MOCCA_limit", "Message Data"=w2312) -> (w2315:T4)
        n990 = Enqueue Element(queue=w2314, element=w2315, error in (no error)=w2313) -> ()  [unwired: 1 in, 3 out]
      }
      event "Save Calibration gas\ncylinder concentration to file": Value Change {
        n991 = event-data() -> ("NewVal"=w2318:bool)  [unwired: 1 in]
        n992 = Bundle(cluster=T4 {"Message"="", "Message Data"=variant} ("Message Cluster"), "Message"="calcon_save", "Message Data"=w2318) -> (w2322:T4)
        n993 = Enqueue Element(queue=w2321, element=w2322, error in (no error)=w2320) -> (error out=w2319:errorcluster)  [unwired: 1 in, 2 out]
      }
      event "Calibration gas cylinder \nconcentration (ppb)": Value Change {
        n994 = event-data() -> ("NewVal"=w2325:dbl)  [unwired: 1 in]
        n995 = Bundle(cluster=T4 {"Message"="", "Message Data"=variant} ("Message Cluster"), "Message"="cal_gas_cylin_conc", "Message Data"=w2325) -> (w2328:T4)
        n996 = Enqueue Element(queue=w2327, element=w2328, error in (no error)=w2326) -> ()  [unwired: 1 in, 3 out]
      }
      event "Simulate MOCCA Conc": Value Change {
        n997 = event-data() -> ("NewVal"=w2331:dbl)  [unwired: 1 in]
        n998 = Bundle(cluster=T4 {"Message"="", "Message Data"=variant} ("Message Cluster"), "Message"="sim_MOCCA_conc", "Message Data"=w2331) -> (w2334:T4)
        n999 = Enqueue Element(queue=w2333, element=w2334, error in (no error)=w2332) -> ()  [unwired: 1 in, 3 out]
      }
      event "MFC_3\nSLPM Value": Value Change {
        n1000 = event-data() -> ("NewVal"=w2340:dbl)  [unwired: 1 in]
        n1001 = Bundle(cluster=T4 {"Message"="", "Message Data"=variant} ("Message Cluster"), "Message"="MFC_3", "Message Data"=w2340) -> (w2338:T4)
        n1002 = Enqueue Element(queue=w2343, element=w2338, error in (no error)=w2342) -> (error out=w2337:errorcluster)  [unwired: 1 in, 2 out]
      }
      event "eV8": Value Change {
        n1003 = event-data() -> ("NewVal"=w2344:bool)  [unwired: 1 in]
        n1004 = Bundle(cluster=T4 {"Message"="", "Message Data"=variant} ("Message Cluster"), "Message"="V8", "Message Data"=w2344) -> (w2348:T4)
        n1005 = Enqueue Element(queue=w2347, element=w2348, error in (no error)=w2346) -> (error out=w2345:errorcluster)  [unwired: 1 in, 2 out]
      }
      event "SO2 eV6": Value Change {
        n1006 = event-data() -> ("NewVal"=w2351:bool)  [unwired: 1 in]
        n1007 = Bundle(cluster=T4 {"Message"="", "Message Data"=variant} ("Message Cluster"), "Message"="V6", "Message Data"=w2351) -> (w2355:T4)
        n1008 = Enqueue Element(queue=w2354, element=w2355, error in (no error)=w2353) -> (error out=w2352:errorcluster)  [unwired: 1 in, 2 out]
      }
      event "Simulate Conc": Value Change {
        n1009 = event-data() -> ("NewVal"=w2358:bool)  [unwired: 1 in]
        n1010 = Bundle(cluster=T4 {"Message"="", "Message Data"=variant} ("Message Cluster"), "Message"="Simulate Conc", "Message Data"=w2358) -> (w2362:T4)
        n1011 = Enqueue Element(queue=w2361, element=w2362, error in (no error)=w2360) -> (error out=w2359:errorcluster)  [unwired: 1 in, 2 out]
      }
      event "SO2 UDP Time Offset": Value Change {
        n1012 = event-data() -> ("NewVal"=w2365:i32)  [unwired: 1 in]
        n1013 = Bundle(cluster=T4 {"Message"="", "Message Data"=variant} ("Message Cluster"), "Message"="UDP Time Offset", "Message Data"=w2365) -> (w2369:T4)
        n1014 = Enqueue Element(queue=w2368, element=w2369, error in (no error)=w2367) -> (error out=w2366:errorcluster)  [unwired: 1 in, 2 out]
      }
      event "Simulate STEL Conc": Value Change {
        n1015 = event-data() -> ("NewVal"=w2372:dbl)  [unwired: 1 in]
        n1016 = Bundle(cluster=T4 {"Message"="", "Message Data"=variant} ("Message Cluster"), "Message"="Simulate STEL Conc", "Message Data"=w2372) -> (w2376:T4)
        n1017 = Enqueue Element(queue=w2375, element=w2376, error in (no error)=w2374) -> (error out=w2373:errorcluster)  [unwired: 1 in, 2 out]
      }
      event "Simulate TWA Conc": Value Change {
        n1018 = event-data() -> ("NewVal"=w2379:dbl)  [unwired: 1 in]
        n1019 = Bundle(cluster=T4 {"Message"="", "Message Data"=variant} ("Message Cluster"), "Message"="Simulate TWA Conc", "Message Data"=w2379) -> (w2383:T4)
        n1020 = Enqueue Element(queue=w2382, element=w2383, error in (no error)=w2381) -> (error out=w2380:errorcluster)  [unwired: 1 in, 2 out]
      }
      event "10mins STEL Limit": Value Change {
        n1021 = event-data() -> ("NewVal"=w2386:i32)  [unwired: 1 in]
        n1022 = Bundle(cluster=T4 {"Message"="", "Message Data"=variant} ("Message Cluster"), "Message"="10mins STEL Limit", "Message Data"=w2386) -> (w2390:T4)
        n1023 = Enqueue Element(queue=w2389, element=w2390, error in (no error)=w2388) -> (error out=w2387:errorcluster)  [unwired: 1 in, 2 out]
      }
      event "8hr TWA Limit": Value Change {
        n1024 = event-data() -> ("NewVal"=w2393:i32)  [unwired: 1 in]
        n1025 = Bundle(cluster=T4 {"Message"="", "Message Data"=variant} ("Message Cluster"), "Message"="8hr TWA Limit", "Message Data"=w2393) -> (w2397:T4)
        n1026 = Enqueue Element(queue=w2396, element=w2397, error in (no error)=w2395) -> (error out=w2394:errorcluster)  [unwired: 1 in, 2 out]
      }
      event "SO2 Zero": Value Change {
        n1027 = event-data() -> ("NewVal"=w2400:dbl)  [unwired: 1 in]
        n1028 = Bundle(cluster=T4 {"Message"="", "Message Data"=variant} ("Message Cluster"), "Message"="Offset", "Message Data"=w2400) -> (w2404:T4)
        n1029 = Enqueue Element(queue=w2403, element=w2404, error in (no error)=w2402) -> (error out=w2401:errorcluster)  [unwired: 1 in, 2 out]
      }
      event "SO2 Sensitivity": Value Change {
        n1030 = event-data() -> ("NewVal"=w2407:dbl)  [unwired: 1 in]
        n1031 = Bundle(cluster=T4 {"Message"="", "Message Data"=variant} ("Message Cluster"), "Message"="Slope", "Message Data"=w2407) -> (w2411:T4)
        n1032 = Enqueue Element(queue=w2410, element=w2411, error in (no error)=w2409) -> (error out=w2408:errorcluster)  [unwired: 1 in, 2 out]
      }
      event "Confirm Flight Number": Value Change {
        n1033 = event-data() -> ()  [unwired: 1 in, 6 out]
        n1034 = flat-sequence {
          tunnel: w2417 -> [w2420]
          tunnel: w2418 -> [w2421]
          tunnel: [w2421] -> w2415
          tunnel: [w2420] -> w2414
          tunnel: [w2423] -> w2416
          tunnel: w2415 -> [w2425]
          tunnel: w2414 -> [w2424]
          frame #0 {
            n1035 = local write "cRIO File IO Stop\n(USB Flash Drive Unmount)"(FALSE ("cRIO File IO Stop\n(USB Flash Drive Unmount)")) -> ()
          }
          frame #1 {
            n1036 = local read "Flight Number"() -> (w2422:string)
            n1037 = Bundle(cluster=T4 {"Message"="", "Message Data"=variant} ("Message Cluster"), "Message"="Flight Number", "Message Data"=w2422) -> (w2426:T4)
            n1038 = Enqueue Element(queue=w2425, element=w2426, error in (no error)=w2424) -> (error out=w2423:errorcluster)  [unwired: 1 in, 2 out]
          }
        }
      }
      event "cRIO File IO Stop\n(USB Flash Drive Unmount)": Value Change {
        n1039 = event-data() -> ("NewVal"=w2429:bool)  [unwired: 1 in]
        n1040 = Bundle(cluster=T4 {"Message"="", "Message Data"=variant} ("Message Cluster"), "Message"="Stop File Write", "Message Data"=w2429) -> (w2433:T4)
        n1041 = Enqueue Element(queue=w2432, element=w2433, error in (no error)=w2431) -> (error out=w2430:errorcluster)  [unwired: 1 in, 2 out]
      }
    }
    "SO2 Event error out" <- w1737
  }
  n1042 = Create Network Stream Writer Endpoint(6:w45, 7:10 ("writer buffer size"), 9:w40, 10:"//192.168.101.17/command/reader/SO2" ("reader url"), 11:"/command/writer/SO2" ("writer name")) -> (0:w44:errorcluster, 3:w43:refnum<k21>)  [unwired: 2 in]
  n1043 = while {
    tunnel: w4 -> [w2440]
    tunnel: w3 -> [w2439]
    stop <- FALSE stop-if-true
    # "SO2 Auto Zero Handler Loop"
    n1044 = local read "Network disconnected"() -> (w2437:bool)
    n1045 = local read "SO2 Zero CAL"() -> (w2444:bool)
    n1046 = Equal?(x=w2444, y=FALSE) -> (x = y?=w2442:bool)
    n1047 = Equal?(x=w2437, y=FALSE) -> (x = y?=w2436:bool)
    n1048 = Compound Arithmetic op=AND("SO2 Auto Zeroing", w2442, w2436) -> (w2445:bool)
    n1049 = case shown="False" w2445 {
      tunnel: w2440 -> [_ w2464]
      tunnel: w2439 -> [_ w2463]
      frame False {
        n1050 = local write "Auto Zero\nIndicator"("Auto Zero Inactive; Manual Zero Allow" ("Auto Zero Indicator")) -> ()
        n1051 = local write "SO2 Pause\nAuto Zeroing"(FALSE ("SO2 Pause\nAuto Zeroing")) -> ()
        n1052 = property on="SO2 Zero CAL" class="Bool (strict)"("Visible"=TRUE) -> ()  [unwired: 2 in, 2 out]
      }
      frame True {
        n1053 = flat-sequence {
          tunnel: w2463 -> [w2473]
          tunnel: w2464 -> [w2474]
          tunnel: [w2474] -> w2462
          tunnel: [w2473] -> w2461
          tunnel: w2462 -> [w2483]
          tunnel: w2461 -> [w2482]
          tunnel: [w2481] -> w2460
          tunnel: [w2480] -> w2459
          tunnel: [w2489] -> w2470
          tunnel: [w2488] -> w2469
          tunnel: w2460 -> [w2493]
          tunnel: w2459 -> [w2494]
          tunnel: w2470 -> [w2498]
          tunnel: [w2497] -> w2468
          tunnel: w2469 -> [w2499]
          tunnel: [w2496] -> w2467
          tunnel: w2468 -> [w2507]
          tunnel: w2467 -> [w2509]
          tunnel: [w2505] -> w2452
          tunnel: [w2504] -> w2451
          tunnel: [w2559] -> w2466
          tunnel: [w2558] -> w2465
          tunnel: w2452 -> [w2561]
          tunnel: w2451 -> [w2560]
          tunnel: w2466 -> [w2577]
          tunnel: w2465 -> [w2576]
          tunnel: [w2574] -> w2457
          tunnel: [w2573] -> w2456
          tunnel: [w2582] -> w2458
          tunnel: w2457 -> [w2582]
          tunnel: w2456 -> [w2581]
          tunnel: [w2581] -> w2455
          tunnel: [w2587] -> w2454
          tunnel: w2455 -> [w2586]
          tunnel: w2458 -> [w2587]
          tunnel: [w2586] -> w2453
          tunnel: w2454 -> [w2621]
          tunnel: w2453 -> [w2620]
          frame #0 {
            n1054 = local write "Auto Zero\nIndicator"("Auto Zero In Progress" ("Auto Zero\nIndicator")) -> ()
            n1055 = while {
              stop <- w2475 stop-if-true
              n1056 = local read "eV9"() -> (w2477:bool)
              n1057 = Equal?(x=w2477, y=FALSE) -> (x = y?=w2475:bool)
              n1058 = Wait (ms)(milliseconds to wait=u32 1000) -> ()  [unwired: 1 out]
            }
            n1059 = property on="SO2 Zero CAL" class="Bool (strict)"("Visible"=FALSE) -> ()  [unwired: 2 in, 2 out]
          }
          frame #1 {
            n1060 = Bundle(cluster=T4 {"Message"="", "Message Data"=variant} ("Message Cluster"), "Message"="Auto_zero", "Message Data"=TRUE) -> (w2484:T4)
            n1061 = Enqueue Element(queue=w2483, element=w2484, error in (no error)=w2482) -> (queue out=w2480:refnum<queue>, error out=w2481:errorcluster)  [unwired: 1 in, 1 out]
          }
          frame #2 {
            w2487 = TRUE ("SO2 Flush")
            n1062 = Bundle(cluster=T4 {"Message"="", "Message Data"=variant} ("Message Cluster"), "Message"="V9", "Message Data"=w2487) -> (w2490:T4)
            n1063 = local write "eV9"(w2487) -> ()
            n1064 = Enqueue Element(queue=w2494, element=w2490, error in (no error)=w2493) -> (queue out=w2488:refnum<queue>, error out=w2489:errorcluster)  [unwired: 1 in, 1 out]
          }
          frame #3 {
            n1065 = local read "MFC_2 User Set Value"() -> (w2495:dbl)
            n1066 = local write "MFC_2 User Set Value"(w2495) -> ()
            n1067 = Bundle(cluster=T4 {"Message"="", "Message Data"=variant} ("Message Cluster"), "Message"="MFC_2", "Message Data"=w2495) -> (w2500:T4)
            n1068 = Enqueue Element(queue=w2499, element=w2500, error in (no error)=w2498) -> (queue out=w2496:refnum<queue>, error out=w2497:errorcluster)  [unwired: 1 in, 1 out]
          }
          frame #4 {
            n1069 = local read "eV9 flush User\nset time (sec)"() -> (w2510:i32)
            n1070 = for {
              N: w2510 -> [w2552]
              tunnel: [w2543] -> w2508
              tunnel: w2509 -> [w2543]
              tunnel: [w2542] -> w2506
              tunnel: w2507 -> [w2542]
              tunnel: [w2541] -> w2503
              i -> [w2551]
              stop <- w2541 stop-if-true
              n1071 = local read "Network disconnected"() -> (w2545:bool)
              n1072 = local read "SO2 Calibration Abort"() -> (w2546:bool)
              n1073 = case shown="True" w2546 {
                selector: w2546 -> [w2555 _]
                tunnel: [w2555 w2556] -> w2544
                frame False {
                }
                frame True {
                  n1074 = Two Button Dialog(message="Are you sure to abort SO2 Cal?") -> (T button?=w2556:bool)  [unwired: 2 in]
                }
              }
              n1075 = Subtract(x=w2552, y=w2551) -> (x-y=w2550:i32)
              n1076 = Decrement(x=w2550) -> (x-1=w2548:i32)
              n1077 = Or(x=w2544, y=w2545) -> (x .or. y?=w2541:bool)
              n1078 = Wait (ms)(milliseconds to wait=u32 1000) -> ()  [unwired: 1 out]
              n1079 = Select(t=0, s=w2541, f=w2548) -> (s? t:f=w2547:i32)
              n1080 = local write "SO2 Zero CAL Flush\nTime Remain (sec)"(w2547) -> ()
              n1081 = case shown="False" w2544 {
                selector: w2544 -> [w2554 _]
                frame False {
                  n1082 = local write "SO2 Calibration Abort"(w2554) -> ()
                }
                frame True {
                }
              }
            }
            n1083 = case shown="False" w2503 {
              tunnel: w2508 -> [w2516 w2540]
              tunnel: w2506 -> [w2515 w2539]
              tunnel: [w2514 w2540] -> w2505
              tunnel: [w2512 w2539] -> w2504
              frame False {
                w2517 = TRUE ("SO2 Flush")
                # "carry on cal when no connection problem or abort not confirmed"
                n1084 = Bundle(cluster=T4 {"Message"="", "Message Data"=variant} ("Message Cluster"), "Message"="V8", "Message Data"=w2517) -> (w2518:T4)
                n1085 = local write "eV8"(w2517) -> ()
                n1086 = Enqueue Element(queue=w2516, element=w2518, error in (no error)=w2515) -> (queue out=w2513:refnum<queue>, error out=w2511:errorcluster)  [unwired: 1 in, 1 out]
                n1087 = local read "eV8 User\nset time (sec)"() -> (w2521:i32)
                n1088 = for {
                  N: w2521 -> [w2533]
                  tunnel: w2513 -> [w2523]
                  tunnel: [w2523] -> w2514
                  tunnel: w2511 -> [w2522]
                  tunnel: [w2522] -> w2512
                  i -> [w2532]
                  stop <- w2524 stop-if-true
                  n1089 = local read "Network disconnected"() -> (w2528:bool)
                  n1090 = local read "SO2 Calibration Abort"() -> (w2530:bool)
                  n1091 = case shown="True" w2530 {
                    selector: w2530 -> [w2536 _]
                    tunnel: [w2536 w2537] -> w2525
                    frame False {
                    }
                    frame True {
                      n1092 = Two Button Dialog(message="Are you sure to abort SO2 Cal?") -> (T button?=w2537:bool)  [unwired: 2 in]
                    }
                  }
                  n1093 = Subtract(x=w2533, y=w2532) -> (x-y=w2531:i32)
                  n1094 = Decrement(x=w2531) -> (x-1=w2526:i32)
                  n1095 = Or(x=w2525, y=w2528) -> (x .or. y?=w2524:bool)
                  n1096 = Wait (ms)(milliseconds to wait=u32 1000) -> ()  [unwired: 1 out]
                  n1097 = Select(t=0, s=w2524, f=w2526) -> (s? t:f=w2527:i32)
                  n1098 = case shown="False" w2525 {
                    selector: w2525 -> [w2535 _]
                    frame False {
                      n1099 = local write "SO2 Calibration Abort"(w2535) -> ()
                    }
                    frame True {
                    }
                  }
                  n1100 = local write "SO2 Zero CAL\nTime Remain (sec)"(w2527) -> ()
                }
              }
              frame True {
                # "Ignore cal when connection problem or abort confirmed"
              }
            }
          }
          frame #5 {
            n1101 = Cluster To Array(cluster=cluster{"Message":string, "Message 2":string} {"Message"="V8", "Message 2"="V9"}) -> (array=w2563:string[])
            n1102 = for {
              tunnel: w2563 -> [w2570] mode=indexing
              tunnel: FALSE ("SO2 Flush") -> [w2569]
              tunnel: w2561 -> [w2568]
              tunnel: w2560 -> [w2567]
              tunnel: [w2566] -> w2559
              tunnel: [w2565] -> w2558
              n1103 = Bundle(cluster=T4 {"Message"="", "Message Data"=variant} ("Message Cluster"), "Message"=w2570, "Message Data"=w2569) -> (w2571:T4)
              n1104 = Enqueue Element(queue=w2568, element=w2571, error in (no error)=w2567) -> (queue out=w2566:refnum<queue>, error out=w2565:errorcluster)  [unwired: 1 in, 1 out]
            }
          }
          frame #6 {
            w2575 = 0.0 ("MFC_2\nSLPM Value")
            n1105 = local write "MFC_2\nSLPM Value"(w2575) -> ()
            n1106 = Bundle(cluster=T4 {"Message"="", "Message Data"=variant} ("Message Cluster"), "Message"="MFC_2", "Message Data"=w2575) -> (w2578:T4)
            n1107 = Enqueue Element(queue=w2577, element=w2578, error in (no error)=w2576) -> (queue out=w2574:refnum<queue>, error out=w2573:errorcluster)  [unwired: 1 in, 1 out]
          }
          frame #7 {
            w2583 = FALSE ("SO2 Flush")
            n1108 = local write "eV8"(w2583) -> ()
            n1109 = local write "eV9"(w2583) -> ()
          }
          frame #8 {
            n1110 = for {
              N: "Auto Zeroing \ninterval (sec)" -> [w2599]
              tunnel: [w2594] -> w2584
              i -> [w2598]
              stop <- w2594 stop-if-true
              n1111 = local read "SO2 Pause\nAuto Zeroing"() -> (w2592:bool)
              n1112 = Subtract(x=w2599, y=w2598) -> (x-y=w2600:i32)
              n1113 = Equal?(x=w2592, y=TRUE) -> (x = y?=w2590:bool)
              n1114 = Decrement(x=w2600) -> (x-1=→"Next Auto Zero\nStarts in (sec)":i32)
              n1115 = Wait (ms)(milliseconds to wait=u32 1000) -> ()  [unwired: 1 out]
              n1116 = case shown="True" w2590 {
                selector: w2590 -> [w2602 _]
                tunnel: [w2602 FALSE] -> w2589
                frame False {
                }
                frame True {
                  n1117 = for {
                    N: "Pause Auto Zero Count \nDown set time (sec)" -> [w2616]
                    tunnel: [w2608] -> w2604
                    i -> [w2615]
                    stop <- w2608 stop-if-true
                    w2609 = FALSE
                    n1118 = local read "SO2 Pause\nAuto Zeroing"() -> (w2611:bool)
                    n1119 = local read "SO2 Auto Zeroing"() -> (w2612:bool)
                    n1120 = Subtract(x=w2616, y=w2615) -> (x-y=w2617:i32)
                    n1121 = Decrement(x=w2617) -> (x-1=→"SO2 Resume Zeroing\nCount down timer (sec)":i32)
                    n1122 = Wait (ms)(milliseconds to wait=u32 1000) -> ()  [unwired: 1 out]
                    n1123 = Equal?(x=w2612, y=w2609) -> (x = y?=w2613:bool)
                    n1124 = Equal?(x=w2611, y=w2609) -> (x = y?=w2610:bool)
                    n1125 = Or(x=w2613, y=w2610) -> (x .or. y?=w2608:bool)
                  }
                  n1126 = case shown="True" w2604 {
                    frame False {
                    }
                    frame True {
                      n1127 = local write "SO2 Resume Zeroing\nCount down timer (sec)"(u32 0 ("SO2 Resume Zeroing\nCount down timer (sec)")) -> ()
                    }
                  }
                  n1128 = local write "Auto Zero\nIndicator"("Auto Zero Paused" ("Auto Zero\nIndicator")) -> ()
                }
              }
              n1129 = local write "Auto Zero\nIndicator"("Waiting For The Next Zeroing\nInterrupt Waiting by Pressing Pause Auto Zeroing button " ("Auto Zero\nIndicator")) -> ()
              n1130 = local read "SO2 Auto Zeroing"() -> (w2595:bool)
              n1131 = local write "SO2 Pause\nAuto Zeroing"(w2589) -> ()
              n1132 = Equal?(x=w2595, y=FALSE) -> (x = y?=w2594:bool)
            }
            n1133 = case shown="True" w2584 {
              frame False {
              }
              frame True {
                n1134 = local write "Next Auto Zero\nStarts in (sec)"(u32 0 ("Next Auto Zero\nStarts in (sec)")) -> ()
              }
            }
          }
          frame #9 {
            n1135 = local write "SO2 Calibration Abort"(FALSE) -> ()
            n1136 = Bundle(cluster=T4 {"Message"="", "Message Data"=variant} ("Message Cluster"), "Message"="Auto_zero", "Message Data"=FALSE) -> (w2624:T4)
            n1137 = Enqueue Element(queue=w2621, element=w2624, error in (no error)=w2620) -> ()  [unwired: 1 in, 3 out]
          }
        }
      }
    }
    n1138 = Wait (ms)(milliseconds to wait=u32 100) -> ()  [unwired: 1 out]
  }
  n1139 = while {
    tunnel: w4 -> [w2633]
    shift-right: [w2628] -> _
    shift-left: w43 -> [w2630]
    shift-right: [w2626] -> w41
    shift-left: w44 -> [w2632]
    tunnel: w3 -> [w2627]
    stop <- w2626 stop-if-true
    # "SO2 UI Command Sender"
    n1140 = Dequeue Element(queue=w2633, error in (no error)=w2627) -> (element=w2629:T4)  [unwired: 1 in, 3 out]
    n1141 = Unbundle By Name(w2629) -> ("Message"=w2631:string)
    n1142 = case shown="\"zeroing_interval\"" w2631 {
      tunnel: w2632 -> [w2634 w2638 w2645 w2652 w2659 w2666 w2673 w2680 w2687 w2694 w2701 w2708 w2715 w2722 w2729 w2736 w2743 w2750 w2757 w2764 w2771 w2778 w2785 w2792 w2799 w2806]
      tunnel: w2630 -> [w2635 w2641 w2648 w2655 w2662 w2669 w2676 w2683 w2690 w2697 w2704 w2711 w2718 w2725 w2732 w2739 w2746 w2753 w2760 w2767 w2774 w2781 w2788 w2795 w2802 w2809]
      tunnel: w2629 -> [_ w2640 w2647 w2654 w2661 w2668 w2675 w2682 w2689 w2696 w2703 w2710 w2717 w2724 w2731 w2738 w2745 w2752 w2759 w2766 w2773 w2780 w2787 w2794 w2801 w2808]
      tunnel: [w2634 w2637 w2644 w2651 w2658 w2665 w2672 w2679 w2686 w2693 w2700 w2707 w2714 w2721 w2728 w2735 w2742 w2749 w2756 w2763 w2770 w2777 w2784 w2791 w2798 w2805] -> w2626
      tunnel: [w2635 w2636 w2643 w2650 w2657 w2664 w2671 w2678 w2685 w2692 w2699 w2706 w2713 w2720 w2727 w2734 w2741 w2748 w2755 w2762 w2769 w2776 w2783 w2790 w2797 w2804] -> w2628
      frame "False", Default {
      }
      frame "V9" {
        n1143 = shared-variable-write(w2641, w2638, w2640) -> (w2639:refnum<k21>, w2642:errorcluster)  [unwired: 1 in, 1 out]
        n1144 = Flush Stream(8:w2642, 11:w2639) -> (0:w2637:errorcluster, 3:w2636:refnum<k21>)  [unwired: 2 in, 1 out]
      }
      frame "MFC_2" {
        n1145 = shared-variable-write(w2648, w2645, w2647) -> (w2646:refnum<k21>, w2649:errorcluster)  [unwired: 1 in, 1 out]
        n1146 = Flush Stream(8:w2649, 11:w2646) -> (0:w2644:errorcluster, 3:w2643:refnum<k21>)  [unwired: 2 in, 1 out]
      }
      frame "MFC_3" {
        n1147 = shared-variable-write(w2655, w2652, w2654) -> (w2653:refnum<k21>, w2656:errorcluster)  [unwired: 1 in, 1 out]
        n1148 = Flush Stream(8:w2656, 11:w2653) -> (0:w2651:errorcluster, 3:w2650:refnum<k21>)  [unwired: 2 in, 1 out]
      }
      frame "V6" {
        n1149 = shared-variable-write(w2662, w2659, w2661) -> (w2660:refnum<k21>, w2663:errorcluster)  [unwired: 1 in, 1 out]
        n1150 = Flush Stream(8:w2663, 11:w2660) -> (0:w2658:errorcluster, 3:w2657:refnum<k21>)  [unwired: 2 in, 1 out]
      }
      frame "Simulate Conc" {
        n1151 = shared-variable-write(w2669, w2666, w2668) -> (w2667:refnum<k21>, w2670:errorcluster)  [unwired: 1 in, 1 out]
        n1152 = Flush Stream(8:w2670, 11:w2667) -> (0:w2665:errorcluster, 3:w2664:refnum<k21>)  [unwired: 2 in, 1 out]
      }
      frame "Simulate STEL Conc" {
        n1153 = shared-variable-write(w2676, w2673, w2675) -> (w2674:refnum<k21>, w2677:errorcluster)  [unwired: 1 in, 1 out]
        n1154 = Flush Stream(8:w2677, 11:w2674) -> (0:w2672:errorcluster, 3:w2671:refnum<k21>)  [unwired: 2 in, 1 out]
      }
      frame "Simulate TWA Conc" {
        n1155 = shared-variable-write(w2683, w2680, w2682) -> (w2681:refnum<k21>, w2684:errorcluster)  [unwired: 1 in, 1 out]
        n1156 = Flush Stream(8:w2684, 11:w2681) -> (0:w2679:errorcluster, 3:w2678:refnum<k21>)  [unwired: 2 in, 1 out]
      }
      frame "10mins STEL Limit" {
        n1157 = shared-variable-write(w2690, w2687, w2689) -> (w2688:refnum<k21>, w2691:errorcluster)  [unwired: 1 in, 1 out]
        n1158 = Flush Stream(8:w2691, 11:w2688) -> (0:w2686:errorcluster, 3:w2685:refnum<k21>)  [unwired: 2 in, 1 out]
      }
      frame "8hr TWA Limit" {
        n1159 = shared-variable-write(w2697, w2694, w2696) -> (w2695:refnum<k21>, w2698:errorcluster)  [unwired: 1 in, 1 out]
        n1160 = Flush Stream(8:w2698, 11:w2695) -> (0:w2693:errorcluster, 3:w2692:refnum<k21>)  [unwired: 2 in, 1 out]
      }
      frame "Offset" {
        n1161 = shared-variable-write(w2704, w2701, w2703) -> (w2702:refnum<k21>, w2705:errorcluster)  [unwired: 1 in, 1 out]
        n1162 = Flush Stream(8:w2705, 11:w2702) -> (0:w2700:errorcluster, 3:w2699:refnum<k21>)  [unwired: 2 in, 1 out]
      }
      frame "eV8_user_set_time" {
        n1163 = shared-variable-write(w2711, w2708, w2710) -> (w2709:refnum<k21>, w2712:errorcluster)  [unwired: 1 in, 1 out]
        n1164 = Flush Stream(8:w2712, 11:w2709) -> (0:w2707:errorcluster, 3:w2706:refnum<k21>)  [unwired: 2 in, 1 out]
      }
      frame "mean_cal_status" {
        n1165 = shared-variable-write(w2718, w2715, w2717) -> (w2716:refnum<k21>, w2719:errorcluster)  [unwired: 1 in, 1 out]
        n1166 = Flush Stream(8:w2719, 11:w2716) -> (0:w2714:errorcluster, 3:w2713:refnum<k21>)  [unwired: 2 in, 1 out]
      }
      frame "SO2_MOCCA_Alarm" {
        n1167 = shared-variable-write(w2725, w2722, w2724) -> (w2723:refnum<k21>, w2726:errorcluster)  [unwired: 1 in, 1 out]
        n1168 = Flush Stream(8:w2726, 11:w2723) -> (0:w2721:errorcluster, 3:w2720:refnum<k21>)  [unwired: 2 in, 1 out]
      }
      frame "MOCCA_window_delay_time" {
        n1169 = shared-variable-write(w2732, w2729, w2731) -> (w2730:refnum<k21>, w2733:errorcluster)  [unwired: 1 in, 1 out]
        n1170 = Flush Stream(8:w2733, 11:w2730) -> (0:w2728:errorcluster, 3:w2727:refnum<k21>)  [unwired: 2 in, 1 out]
      }
      frame "MOCCA_limit" {
        n1171 = shared-variable-write(w2739, w2736, w2738) -> (w2737:refnum<k21>, w2740:errorcluster)  [unwired: 1 in, 1 out]
        n1172 = Flush Stream(8:w2740, 11:w2737) -> (0:w2735:errorcluster, 3:w2734:refnum<k21>)  [unwired: 2 in, 1 out]
      }
      frame "calcon_save" {
        n1173 = shared-variable-write(w2746, w2743, w2745) -> (w2744:refnum<k21>, w2747:errorcluster)  [unwired: 1 in, 1 out]
        n1174 = Flush Stream(8:w2747, 11:w2744) -> (0:w2742:errorcluster, 3:w2741:refnum<k21>)  [unwired: 2 in, 1 out]
      }
      frame "Auto_zero" {
        n1175 = shared-variable-write(w2753, w2750, w2752) -> (w2751:refnum<k21>, w2754:errorcluster)  [unwired: 1 in, 1 out]
        n1176 = Flush Stream(8:w2754, 11:w2751) -> (0:w2749:errorcluster, 3:w2748:refnum<k21>)  [unwired: 2 in, 1 out]
      }
      frame "zeroing_interval" {
        n1177 = shared-variable-write(w2760, w2757, w2759) -> (w2758:refnum<k21>, w2761:errorcluster)  [unwired: 1 in, 1 out]
        n1178 = Flush Stream(8:w2761, 11:w2758) -> (0:w2756:errorcluster, 3:w2755:refnum<k21>)  [unwired: 2 in, 1 out]
      }
      frame "cal_gas_cylin_conc" {
        n1179 = shared-variable-write(w2767, w2764, w2766) -> (w2765:refnum<k21>, w2768:errorcluster)  [unwired: 1 in, 1 out]
        n1180 = Flush Stream(8:w2768, 11:w2765) -> (0:w2763:errorcluster, 3:w2762:refnum<k21>)  [unwired: 2 in, 1 out]
      }
      frame "sim_MOCCA_conc" {
        n1181 = shared-variable-write(w2774, w2771, w2773) -> (w2772:refnum<k21>, w2775:errorcluster)  [unwired: 1 in, 1 out]
        n1182 = Flush Stream(8:w2775, 11:w2772) -> (0:w2770:errorcluster, 3:w2769:refnum<k21>)  [unwired: 2 in, 1 out]
      }
      frame "Slope" {
        n1183 = shared-variable-write(w2781, w2778, w2780) -> (w2779:refnum<k21>, w2782:errorcluster)  [unwired: 1 in, 1 out]
        n1184 = Flush Stream(8:w2782, 11:w2779) -> (0:w2777:errorcluster, 3:w2776:refnum<k21>)  [unwired: 2 in, 1 out]
      }
      frame "Flight Number" {
        n1185 = shared-variable-write(w2788, w2785, w2787) -> (w2786:refnum<k21>, w2789:errorcluster)  [unwired: 1 in, 1 out]
        n1186 = Flush Stream(8:w2789, 11:w2786) -> (0:w2784:errorcluster, 3:w2783:refnum<k21>)  [unwired: 2 in, 1 out]
      }
      frame "Stop File Write" {
        n1187 = shared-variable-write(w2795, w2792, w2794) -> (w2793:refnum<k21>, w2796:errorcluster)  [unwired: 1 in, 1 out]
        n1188 = Flush Stream(8:w2796, 11:w2793) -> (0:w2791:errorcluster, 3:w2790:refnum<k21>)  [unwired: 2 in, 1 out]
      }
      frame "UDP Time Offset" {
        n1189 = shared-variable-write(w2802, w2799, w2801) -> (w2800:refnum<k21>, w2803:errorcluster)  [unwired: 1 in, 1 out]
        n1190 = Flush Stream(8:w2803, 11:w2800) -> (0:w2798:errorcluster, 3:w2797:refnum<k21>)  [unwired: 2 in, 1 out]
      }
      frame "V8" {
        n1191 = shared-variable-write(w2809, w2806, w2808) -> (w2807:refnum<k21>, w2810:errorcluster)  [unwired: 1 in, 1 out]
        n1192 = Flush Stream(8:w2810, 11:w2807) -> (0:w2805:errorcluster, 3:w2804:refnum<k21>)  [unwired: 2 in, 1 out]
      }
    }
  }
  "SO2 command sender \nerror out" <- w41
  n1193 = Obtain Queue(name (unnamed)="TEi43c_Command", element data type=w29) -> (queue out=w38:refnum<queue>, error out=w31:errorcluster)  [unwired: 3 in, 1 out]
  n1194 = Create Network Stream Writer Endpoint(6:w35, 7:10 ("writer buffer size"), 9:w29, 10:"//192.168.101.17/command/reader/TEi43c" ("reader url"), 11:"/command/writer/TEi43c" ("writer name")) -> (0:w34:errorcluster, 3:w33:refnum<k21>)  [unwired: 2 in]
  n1195 = while {
    tunnel: w38 -> [w2814]
    tunnel: w31 -> [w2813]
    tunnel: [w2811] -> _
    stop <- FALSE stop-if-true
    # "TEi43c Ozone UI Event Handler Loop"
    n1196 = event shown="[0] \"Ozone Zeroing\": Value Change" {
      selector: _ -> [_ _ _ _ _]
      dyn-events: _ -> [_ _ _ _ _]
      timeout: _ -> [_ _ _ _ _]
      tunnel: w2814 -> [w2822 w2860 w2868 w2875 w2883]
      tunnel: w2813 -> [w2821 w2859 w2867 w2874 w2882]
      tunnel: [w2820 w2858 w2866 w2873 w2881] -> w2811
      event "Ozone Zeroing": Value Change {
        n1197 = event-data() -> ()  [unwired: 1 in, 6 out]
        n1198 = flat-sequence {
          tunnel: w2822 -> [w2827]
          tunnel: w2821 -> [w2826]
          tunnel: [w2825] -> w2819
          tunnel: [w2823] -> w2815
          tunnel: w2819 -> [w2833]
          tunnel: [w2833] -> w2818
          tunnel: [w2831] -> w2816
          tunnel: w2815 -> [w2831]
          tunnel: w2818 -> [w2851]
          tunnel: [w2850] -> w2817
          tunnel: w2816 -> [w2852]
          tunnel: [w2857] -> w2820
          tunnel: w2817 -> [w2857]
          frame #0 {
            w2824 = TRUE
            n1199 = local write "Ozone eV6"(w2824) -> ()
            n1200 = Bundle(cluster=T4 {"Message"="", "Message Data"=variant} ("Message Cluster"), "Message"="V6", "Message Data"=w2824) -> (w2828:T4)
            n1201 = Enqueue Element(queue=w2827, element=w2828, error in (no error)=w2826) -> (queue out=w2823:refnum<queue>, error out=w2825:errorcluster)  [unwired: 1 in, 1 out]
          }
          frame #1 {
            # "10 Mins Count down"
            n1202 = for {
              N: 600 -> [w2843]
              i -> [w2842]
              stop <- w2835 stop-if-true
              n1203 = local read "Ozone Zeroing Abort"() -> (w2837:bool)
              n1204 = Subtract(x=w2843, y=w2842) -> (x-y=w2841:i32)
              n1205 = Decrement(x=w2841) -> (x-1=w2839:i32)
              n1206 = Wait (ms)(milliseconds to wait=u32 1000) -> ()  [unwired: 1 out]
              n1207 = case shown="True" w2837 {
                selector: w2837 -> [w2846 _]
                tunnel: [w2846 w2847] -> w2834
                frame False {
                }
                frame True {
                  n1208 = Two Button Dialog(message="Are you sure to abort Ozone Zeroing?") -> (T button?=w2847:bool)  [unwired: 2 in]
                }
              }
              n1209 = local read "Network disconnected"() -> (w2836:bool)
              n1210 = Or(x=w2836, y=w2834) -> (x .or. y?=w2835:bool)
              n1211 = Select(t=0, s=w2835, f=w2839) -> (s? t:f=→"Ozone Zeroing\nTime Remain (sec)":i32)
              n1212 = case shown="False" w2834 {
                selector: w2834 -> [w2845 _]
                frame False {
                  n1213 = local write "Ozone Zeroing Abort"(w2845) -> ()
                }
                frame True {
                }
              }
            }
          }
          frame #2 {
            w2849 = FALSE
            n1214 = local write "Ozone eV6"(w2849) -> ()
            n1215 = Bundle(cluster=T4 {"Message"="", "Message Data"=variant} ("Message Cluster"), "Message"="V6", "Message Data"=w2849) -> (w2853:T4)
            n1216 = Enqueue Element(queue=w2852, element=w2853, error in (no error)=w2851) -> (error out=w2850:errorcluster)  [unwired: 1 in, 2 out]
          }
          frame #3 {
            w2856 = FALSE ("Ozone Zeroing")
            n1217 = local write "Ozone Zeroing Abort"(w2856) -> ()
            n1218 = local write "Ozone Zeroing"(w2856) -> ()
          }
        }
      }
      event "Ozone eV6": Value Change {
        n1219 = event-data() -> ("NewVal"=w2861:bool)  [unwired: 1 in]
        n1220 = Bundle(cluster=T4 {"Message"="", "Message Data"=variant} ("Message Cluster"), "Message"="V6", "Message Data"=w2861) -> (w2862:T4)
        n1221 = Enqueue Element(queue=w2860, element=w2862, error in (no error)=w2859) -> (error out=w2858:errorcluster)  [unwired: 1 in, 2 out]
      }
      event "cRIO File IO Stop\n(USB Flash Drive Unmount)": Value Change {
        n1222 = event-data() -> ("NewVal"=w2865:bool)  [unwired: 1 in]
        n1223 = Bundle(cluster=T4 {"Message"="", "Message Data"=variant} ("Message Cluster"), "Message"="Stop File Write", "Message Data"=w2865) -> (w2869:T4)
        n1224 = Enqueue Element(queue=w2868, element=w2869, error in (no error)=w2867) -> (error out=w2866:errorcluster)  [unwired: 1 in, 2 out]
      }
      event "Ozone UDP Time Offset": Value Change {
        n1225 = event-data() -> ("NewVal"=w2872:i32)  [unwired: 1 in]
        n1226 = Bundle(cluster=T4 {"Message"="", "Message Data"=variant} ("Message Cluster"), "Message"="UDP Time Offset", "Message Data"=w2872) -> (w2876:T4)
        n1227 = Enqueue Element(queue=w2875, element=w2876, error in (no error)=w2874) -> (error out=w2873:errorcluster)  [unwired: 1 in, 2 out]
      }
      event "Confirm Flight Number": Value Change {
        n1228 = event-data() -> ()  [unwired: 1 in, 5 out]
        n1229 = flat-sequence {
          tunnel: w2882 -> [w2885]
          tunnel: w2883 -> [w2886]
          tunnel: [w2886] -> w2880
          tunnel: [w2885] -> w2879
          tunnel: [w2888] -> w2881
          tunnel: w2880 -> [w2890]
          tunnel: w2879 -> [w2889]
          frame #0 {
            n1230 = local write "cRIO File IO Stop\n(USB Flash Drive Unmount)"(FALSE ("cRIO File IO Stop\n(USB Flash Drive Unmount)")) -> ()
          }
          frame #1 {
            n1231 = local read "Flight Number"() -> (w2887:string)
            n1232 = Bundle(cluster=T4 {"Message"="", "Message Data"=variant} ("Message Cluster"), "Message"="Flight Number", "Message Data"=w2887) -> (w2891:T4)
            n1233 = Enqueue Element(queue=w2890, element=w2891, error in (no error)=w2889) -> (error out=w2888:errorcluster)  [unwired: 1 in, 2 out]
          }
        }
      }
    }
    "Ozone Event error out" <- w2811
  }
  n1234 = while {
    tunnel: w38 -> [w2901]
    shift-right: [w2896] -> _
    shift-left: w33 -> [w2898]
    shift-right: [w2894] -> w30
    shift-left: w34 -> [w2900]
    tunnel: w31 -> [w2895]
    stop <- w2894 stop-if-true
    # "TEi43c Ozone UI Command Sender"
    n1235 = Dequeue Element(queue=w2901, error in (no error)=w2895) -> (element=w2897:T4)  [unwired: 1 in, 3 out]
    n1236 = Unbundle By Name(w2897) -> ("Message"=w2899:string)
    n1237 = case shown="\"UDP Time Offset\"" w2899 {
      tunnel: w2900 -> [w2902 w2906 w2913 w2920 w2927]
      tunnel: w2898 -> [w2903 w2909 w2916 w2923 w2930]
      tunnel: w2897 -> [_ w2908 w2915 w2922 w2929]
      tunnel: [w2902 w2905 w2912 w2919 w2926] -> w2894
      tunnel: [w2903 w2904 w2911 w2918 w2925] -> w2896
      frame "False", Default {
      }
      frame "V6" {
        n1238 = shared-variable-write(w2909, w2906, w2908) -> (w2907:refnum<k21>, w2910:errorcluster)  [unwired: 1 in, 1 out]
        n1239 = Flush Stream(8:w2910, 11:w2907) -> (0:w2905:errorcluster, 3:w2904:refnum<k21>)  [unwired: 2 in, 1 out]
      }
      frame "Stop File Write" {
        n1240 = shared-variable-write(w2916, w2913, w2915) -> (w2914:refnum<k21>, w2917:errorcluster)  [unwired: 1 in, 1 out]
        n1241 = Flush Stream(8:w2917, 11:w2914) -> (0:w2912:errorcluster, 3:w2911:refnum<k21>)  [unwired: 2 in, 1 out]
      }
      frame "Flight Number" {
        n1242 = shared-variable-write(w2923, w2920, w2922) -> (w2921:refnum<k21>, w2924:errorcluster)  [unwired: 1 in, 1 out]
        n1243 = Flush Stream(8:w2924, 11:w2921) -> (0:w2919:errorcluster, 3:w2918:refnum<k21>)  [unwired: 2 in, 1 out]
      }
      frame "UDP Time Offset" {
        n1244 = shared-variable-write(w2930, w2927, w2929) -> (w2928:refnum<k21>, w2931:errorcluster)  [unwired: 1 in, 1 out]
        n1245 = Flush Stream(8:w2931, 11:w2928) -> (0:w2926:errorcluster, 3:w2925:refnum<k21>)  [unwired: 2 in, 1 out]
      }
    }
  }
  "Ozone command sender error out" <- w30
  n1246 = Obtain Queue(name (unnamed)="2BOzone_Command", element data type=w17) -> (queue out=w26:refnum<queue>, error out=w19:errorcluster)  [unwired: 3 in, 1 out]
  n1247 = Create Network Stream Writer Endpoint(6:w23, 7:10 ("writer buffer size"), 9:w17, 10:"//192.168.101.17/command/reader/2BOzone" ("reader url"), 11:"/command/writer/2BOzone" ("writer name")) -> (0:w22:errorcluster, 3:w21:refnum<k21>)  [unwired: 2 in]
  n1248 = while {
    tunnel: w26 -> [w2935]
    tunnel: w19 -> [w2934]
    tunnel: [w2932] -> _
    stop <- FALSE stop-if-true
    # "2BOzone UI Event Handler Loop"
    n1249 = event shown="[2] \"Simulate Inst Conc\": Value Change" {
      selector: _ -> [_ _ _ _ _ _ _ _]
      dyn-events: _ -> [_ _ _ _ _ _ _ _]
      timeout: _ -> [_ _ _ _ _ _ _ _]
      tunnel: w2935 -> [w2939 w2946 w2953 w2960 w2967 w2974 w2981 w2989]
      tunnel: w2934 -> [w2938 w2945 w2952 w2959 w2966 w2973 w2980 w2988]
      tunnel: [w2937 w2944 w2951 w2958 w2965 w2972 w2979 w2987] -> w2932
      event "Ambient = OFF\nCabin = ON": Value Change {
        n1250 = event-data() -> ("NewVal"=w2936:bool)  [unwired: 1 in]
        n1251 = Bundle(cluster=T4 {"Message"="", "Message Data"=variant} ("Message Cluster"), "Message"="Ambient/Cabin", "Message Data"=w2936) -> (w2940:T4)
        n1252 = Enqueue Element(queue=w2939, element=w2940, error in (no error)=w2938) -> (error out=w2937:errorcluster)  [unwired: 1 in, 2 out]
      }
      event "Simulate 2B Conc": Value Change {
        n1253 = event-data() -> ("NewVal"=w2943:bool)  [unwired: 1 in]
        n1254 = Bundle(cluster=T4 {"Message"="", "Message Data"=variant} ("Message Cluster"), "Message"="Simulate_conc", "Message Data"=w2943) -> (w2947:T4)
        n1255 = Enqueue Element(queue=w2946, element=w2947, error in (no error)=w2945) -> (error out=w2944:errorcluster)  [unwired: 1 in, 2 out]
      }
      event "Simulate Inst Conc": Value Change {
        n1256 = event-data() -> ("NewVal"=w2950:i32)  [unwired: 1 in]
        n1257 = Bundle(cluster=T4 {"Message"="", "Message Data"=variant} ("Message Cluster"), "Message"="Simulate_inst_conc", "Message Data"=w2950) -> (w2954:T4)
        n1258 = Enqueue Element(queue=w2953, element=w2954, error in (no error)=w2952) -> (error out=w2951:errorcluster)  [unwired: 1 in, 2 out]
      }
      event "Inst_alm_thresh": Value Change {
        n1259 = event-data() -> ("NewVal"=w2957:i32)  [unwired: 1 in]
        n1260 = Bundle(cluster=T4 {"Message"="", "Message Data"=variant} ("Message Cluster"), "Message"="Inst_alm_thresh", "Message Data"=w2957) -> (w2961:T4)
        n1261 = Enqueue Element(queue=w2960, element=w2961, error in (no error)=w2959) -> (error out=w2958:errorcluster)  [unwired: 1 in, 2 out]
      }
      event "3hr_alm_thresh": Value Change {
        n1262 = event-data() -> ("NewVal"=w2964:i32)  [unwired: 1 in]
        n1263 = Bundle(cluster=T4 {"Message"="", "Message Data"=variant} ("Message Cluster"), "Message"="3hr_alm_thresh", "Message Data"=w2964) -> (w2968:T4)
        n1264 = Enqueue Element(queue=w2967, element=w2968, error in (no error)=w2966) -> (error out=w2965:errorcluster)  [unwired: 1 in, 2 out]
      }
      event "Simulate 3hr Average Conc": Value Change {
        n1265 = event-data() -> ("NewVal"=w2971:dbl)  [unwired: 1 in]
        n1266 = Bundle(cluster=T4 {"Message"="", "Message Data"=variant} ("Message Cluster"), "Message"="Simulate_3hr_av_conc", "Message Data"=w2971) -> (w2975:T4)
        n1267 = Enqueue Element(queue=w2974, element=w2975, error in (no error)=w2973) -> (error out=w2972:errorcluster)  [unwired: 1 in, 2 out]
      }
      event "cRIO File IO Stop\n(USB Flash Drive Unmount)": Value Change {
        n1268 = event-data() -> ("NewVal"=w2978:bool)  [unwired: 1 in]
        n1269 = Bundle(cluster=T4 {"Message"="", "Message Data"=variant} ("Message Cluster"), "Message"="Stop File Write", "Message Data"=w2978) -> (w2982:T4)
        n1270 = Enqueue Element(queue=w2981, element=w2982, error in (no error)=w2980) -> (error out=w2979:errorcluster)  [unwired: 1 in, 2 out]
      }
      event "Confirm Flight Number": Value Change {
        n1271 = event-data() -> ()  [unwired: 1 in, 5 out]
        n1272 = flat-sequence {
          tunnel: w2988 -> [w2991]
          tunnel: w2989 -> [w2992]
          tunnel: [w2992] -> w2986
          tunnel: [w2991] -> w2985
          tunnel: [w2994] -> w2987
          tunnel: w2986 -> [w2996]
          tunnel: w2985 -> [w2995]
          frame #0 {
            n1273 = local write "cRIO File IO Stop\n(USB Flash Drive Unmount)"(FALSE ("cRIO File IO Stop\n(USB Flash Drive Unmount)")) -> ()
          }
          frame #1 {
            n1274 = local read "Flight Number"() -> (w2993:string)
            n1275 = Bundle(cluster=T4 {"Message"="", "Message Data"=variant} ("Message Cluster"), "Message"="Flight Number", "Message Data"=w2993) -> (w2997:T4)
            n1276 = Enqueue Element(queue=w2996, element=w2997, error in (no error)=w2995) -> (error out=w2994:errorcluster)  [unwired: 1 in, 2 out]
          }
        }
      }
    }
    "2BOzone Event error out" <- w2932
  }
  n1277 = while {
    tunnel: w26 -> [w3007]
    shift-right: [w3002] -> _
    shift-left: w21 -> [w3004]
    shift-right: [w3000] -> w18
    shift-left: w22 -> [w3006]
    tunnel: w19 -> [w3001]
    stop <- w3000 stop-if-true
    # "2BOzone UI Command Sender"
    n1278 = Dequeue Element(queue=w3007, error in (no error)=w3001) -> (element=w3003:T4)  [unwired: 1 in, 3 out]
    n1279 = Unbundle By Name(w3003) -> ("Message"=w3005:string)
    n1280 = case shown="\"3hr_alm_thresh\"" w3005 {
      tunnel: w3006 -> [w3008 w3012 w3019 w3026 w3033 w3040 w3047 w3054 w3061]
      tunnel: w3004 -> [w3009 w3015 w3022 w3029 w3036 w3043 w3050 w3057 w3064]
      tunnel: w3003 -> [_ w3014 w3021 w3028 w3035 w3042 w3049 w3056 w3063]
      tunnel: [w3008 w3011 w3018 w3025 w3032 w3039 w3046 w3053 w3060] -> w3000
      tunnel: [w3009 w3010 w3017 w3024 w3031 w3038 w3045 w3052 w3059] -> w3002
      frame "False", Default {
      }
      frame "Ambient/Cabin" {
        n1281 = shared-variable-write(w3015, w3012, w3014) -> (w3013:refnum<k21>, w3016:errorcluster)  [unwired: 1 in, 1 out]
        n1282 = Flush Stream(8:w3016, 11:w3013) -> (0:w3011:errorcluster, 3:w3010:refnum<k21>)  [unwired: 2 in, 1 out]
      }
      frame "Simulate_conc" {
        n1283 = shared-variable-write(w3022, w3019, w3021) -> (w3020:refnum<k21>, w3023:errorcluster)  [unwired: 1 in, 1 out]
        n1284 = Flush Stream(8:w3023, 11:w3020) -> (0:w3018:errorcluster, 3:w3017:refnum<k21>)  [unwired: 2 in, 1 out]
      }
      frame "Simulate_inst_conc" {
        n1285 = shared-variable-write(w3029, w3026, w3028) -> (w3027:refnum<k21>, w3030:errorcluster)  [unwired: 1 in, 1 out]
        n1286 = Flush Stream(8:w3030, 11:w3027) -> (0:w3025:errorcluster, 3:w3024:refnum<k21>)  [unwired: 2 in, 1 out]
      }
      frame "Inst_alm_thresh" {
        n1287 = shared-variable-write(w3036, w3033, w3035) -> (w3034:refnum<k21>, w3037:errorcluster)  [unwired: 1 in, 1 out]
        n1288 = Flush Stream(8:w3037, 11:w3034) -> (0:w3032:errorcluster, 3:w3031:refnum<k21>)  [unwired: 2 in, 1 out]
      }
      frame "3hr_alm_thresh" {
        n1289 = shared-variable-write(w3043, w3040, w3042) -> (w3041:refnum<k21>, w3044:errorcluster)  [unwired: 1 in, 1 out]
        n1290 = Flush Stream(8:w3044, 11:w3041) -> (0:w3039:errorcluster, 3:w3038:refnum<k21>)  [unwired: 2 in, 1 out]
      }
      frame "Simulate_3hr_av_conc" {
        n1291 = shared-variable-write(w3050, w3047, w3049) -> (w3048:refnum<k21>, w3051:errorcluster)  [unwired: 1 in, 1 out]
        n1292 = Flush Stream(8:w3051, 11:w3048) -> (0:w3046:errorcluster, 3:w3045:refnum<k21>)  [unwired: 2 in, 1 out]
      }
      frame "Stop File Write" {
        n1293 = shared-variable-write(w3057, w3054, w3056) -> (w3055:refnum<k21>, w3058:errorcluster)  [unwired: 1 in, 1 out]
        n1294 = Flush Stream(8:w3058, 11:w3055) -> (0:w3053:errorcluster, 3:w3052:refnum<k21>)  [unwired: 2 in, 1 out]
      }
      frame "Flight Number" {
        n1295 = shared-variable-write(w3064, w3061, w3063) -> (w3062:refnum<k21>, w3065:errorcluster)  [unwired: 1 in, 1 out]
        n1296 = Flush Stream(8:w3065, 11:w3062) -> (0:w3060:errorcluster, 3:w3059:refnum<k21>)  [unwired: 2 in, 1 out]
      }
    }
  }
  "2BOzone command sender error out" <- w18
